vi "IETS_sweep routine_2021_subvis.vi"(0 "Yokogawa 7651":refnum<visa-resource-name>="GPIB0::13::INSTR", 1 "LIA1":refnum<visa-resource-name>="GPIB0::8::INSTR", 2 "Sens_LIA 1":dbl=0.2, 3 "AC amp":dbl=0.3, 4 "LIA2":refnum<visa-resource-name>="GPIB0::20::INSTR", 5 "file path 3":path=path "D:/MCBJ_DATA/IETS_new programm/ganz neu/S1_2021/AuAu/50mV/30_03_2021/cooldownsweep0128", 6 "pre-resistance":dbl=50.0 format="%#_13g", 7 "file path 2":path=path "D:/MCBJ_DATA/IETS_new programm/ganz neu/S1_2021/AuAu/50mV/30_03_2021/coolupsweep0128", 8 "Initail V":dbl=-0.52, 9 "CA gain":dbl=0.0001, 10 "LIA exp 2":dbl=100.0, 12 "Step (V)":dbl=0.001, 14 "Sensitivity 2":dbl=0.2, 15 "Set0 step (V)":dbl=0.002 format="%#.6g", 16 "Final V":dbl=0.52, 17 "Stop":bool, 18 "bias_in":dbl=0.05, 19 "Lia1_pase":dbl, 20 "file path":path=path "D:/MCBJ_DATA/IETS_new programm/ganz neu/S1_2021/AuAu/50mV/30_03_2021/coolIETS0128", 22 "LIA exp 1":dbl=1.0, 23 "Resistance":dbl=1832.6738253037915, 24 "motor-info":string="Data_Points   O/C_Cyles  Motor_Pos  lockin_phase  Temperature Voltage_drop LockAmpl timeLIA1 timeLIA2   OC_timestamp \r81800\t13\t333511\t90\t10.921\t234\t3\t8\t8\tH:06:31,1523\t", 26 "Cond (G0)":dbl=7.042390613771767) -> (13 "allchart_lia2":cluster{"x":dbl, "y":dbl}[](graph), 21 "VISA Agilent out":refnum<visa-resource-name>="GPIB0::10::INSTR", 25 "IV_allchart":cluster{"x":dbl, "y":dbl}[](graph), 27 "allchart_Lia1":cluster{"X":dbl, "Y":dbl}[](graph))   [LabVIEW 2016]
uses:
  Instance           2 12Saved   IETS .vi
  Agilent 3446X Series/Agilent 3446X Series.lvlib
  Keithley DMM6500 DAQ6500 Series/Keithley DMM6500 DAQ6500 Series.lvlib
  Agilent 34401/Agilent 34401.lvlib
panel:
  out "G_drop":dbl=0.054506536639635256
  out "Current mA":dbl=33.097697080199396
  out "LIA_DMM_G":dbl=-8.943673289039905
  out "sec ampl":dbl=-0.0004827649974186888
  out "Meas Bias":dbl=-0.0446874833
  out "Lia2_DMM":dbl=-0.168320844
  out "LIAI_1_DMM":dbl=-1.07675359
  out "stop last sweep":bool=TRUE
  out "Abort":bool=TRUE
  in  "Stop 2":bool
  out "Vspt":dbl=-0.052
  out "Vdrop":dbl=0.3437052
  in  "?":T1(tab)=enum."conditions"
  out "IV_chart":cluster{"x":dbl, "y":dbl}[](graph)=[{"x"=-0.338726307, "y"=884.433039501003}, {"x"=-0.338726307, "y"=884.433039501003}, {"x"=-0.338726307, "y"=884.433039501003}, {"x"=-0.338726307, "y"=884.433039501003}, {"x"=-0.338726307, "y"=884.433039501003}, {"x"=-0.338726307, "y"=884.433039501003}, {"x"=-0.338726307, "y"=884.433039501003}, {"x"=-0.338726307, "y"=884.433039501003}, {"x"=-0.338726307, "y"=884.433039501003}, {"x"=-0.338726307, "y"=884.433039501003}, {"x"=-0.338726307, "y"=884.433039501003}, {"x"=-0.338726307, "y"=884.433039501003}, {"x"=-0.338726307, "y"=884.433039501003}, {"x"=-0.338726307, "y"=884.433039501003}, {"x"=-0.338726307, "y"=884.433039501003}, {"x"=-0.338726307, "y"=884.433039501003}, {"x"=-0.338726307, "y"=884.433039501003}, {"x"=-0.338726307, "y"=884.433039501003}, {"x"=-0.338726307, "y"=884.433039501003}, {"x"=-0.338726307, "y"=884.433039501003}, {"x"=-0.338726307, "y"=884.433039501003}, {"x"=-0.338726307, "y"=884.433039501003}, {"x"=-0.338726307, "y"=884.433039501003}, {"x"=-0.338726307, "y"=884.433039501003}, {"x"=-0.338726307, "y"=884.433039501003}, {"x"=-0.338726307, "y"=884.433039501003}, {"x"=-0.338726307, "y"=884.433039501003}, {"x"=-0.338726307, "y"=884.433039501003}, {"x"=-0.338726307, "y"=884.433039501003}, {"x"=-0.338726307, "y"=884.433039501003}, {"x"=-0.338726307, "y"=884.433039501003}, {"x"=-0.338726307, "y"=884.433039501003}, {"x"=-0.338726307, "y"=884.433039501003}, {"x"=-0.338726307, "y"=884.433039501003}, {"x"=-0.338726307, "y"=884.433039501003}, {"x"=-0.338726307, "y"=884.433039501003}, {"x"=-0.338726307, "y"=884.433039501003}, {"x"=-0.338726307, "y"=884.433039501003}, {"x"=-0.338726307, "y"=884.433039501003}, {"x"=-0.338726307, "y"=884.433039501003}, {"x"=-0.338726307, "y"=884.433039501003}, {"x"=-0.338726307, "y"=884.433039501003}, {"x"=-0.338726307, "y"=884.433039501003}, {"x"=-0.338726307, "y"=884.433039501003}, {"x"=-0.338726307, "y"=884.433039501003}, {"x"=-0.338726307, "y"=884.433039501003}, {"x"=-0.338726307, "y"=884.433039501003}, {"x"=-0.338726307, "y"=884.433039501003}, {"x"=-0.338726307, "y"=884.433039501003}, {"x"=-0.338726307, "y"=884.433039501003}, {"x"=-0.338726307, "y"=884.433039501003}, {"x"=-0.338726307, "y"=884.433039501003}, {"x"=-0.338726307, "y"=884.433039501003}, {"x"=-0.338726307, "y"=884.433039501003}, {"x"=-0.338726307, "y"=884.433039501003}, {"x"=-0.338726307, "y"=884.433039501003}, {"x"=-0.338726307, "y"=884.433039501003}, {"x"=-0.338726307, "y"=884.433039501003}, {"x"=-0.338726307, "y"=884.433039501003}, {"x"=-0.338726307, "y"=884.433039501003}, {"x"=-0.338726307, "y"=884.433039501003}, {"x"=-0.338726307, "y"=884.433039501003}, {"x"=-0.338726307, "y"=884.433039501003}, {"x"=-0.338726307, "y"=884.433039501003}, {"x"=-0.338726307, "y"=884.433039501003}, {"x"=-0.338726307, "y"=884.433039501003}, {"x"=-0.338726307, "y"=884.433039501003}, {"x"=-0.338726307, "y"=884.433039501003}, {"x"=-0.338726307, "y"=884.433039501003}, {"x"=-0.338726307, "y"=884.433039501003}, {"x"=-0.338726307, "y"=884.433039501003}, {"x"=-0.338726307, "y"=884.433039501003}, {"x"=-0.338726307, "y"=884.433039501003}, {"x"=-0.338726307, "y"=884.433039501003}, {"x"=-0.338726307, "y"=884.433039501003}, {"x"=-0.338726307, "y"=884.433039501003}, {"x"=-0.338726307, "y"=884.433039501003}, {"x"=-0.338726307, "y"=884.433039501003}, {"x"=-0.338726307, "y"=884.433039501003}, {"x"=-0.338726307, "y"=884.433039501003}, {"x"=-0.338726307, "y"=884.433039501003}, {"x"=-0.338726307, "y"=884.433039501003}, {"x"=-0.338726307, "y"=884.433039501003}, {"x"=-0.338726307, "y"=884.433039501003}, {"x"=-0.338726307, "y"=884.433039501003}, {"x"=-0.338726307, "y"=884.433039501003}, {"x"=-0.338726307, "y"=884.433039501003}, {"x"=-0.338726307, "y"=884.433039501003}, {"x"=-0.338726307, "y"=884.433039501003}, {"x"=-0.338726307, "y"=884.433039501003}, {"x"=-0.338726307, "y"=884.433039501003}, {"x"=-0.338726307, "y"=884.433039501003}, {"x"=-0.338726307, "y"=884.433039501003}, {"x"=-0.338726307, "y"=884.433039501003}, {"x"=-0.338726307, "y"=884.433039501003}, {"x"=-0.338726307, "y"=884.433039501003}, {"x"=-0.338726307, "y"=884.433039501003}, {"x"=-0.338726307, "y"=884.433039501003}, {"x"=-0.338726307, "y"=884.433039501003}, {"x"=-0.338726307, "y"=884.433039501003}, {"x"=-0.338726307, "y"=884.433039501003}, {"x"=-0.338726307, "y"=884.433039501003}, {"x"=-0.338726307, "y"=884.433039501003}, {"x"=-0.338726307, "y"=884.433039501003}, {"x"=-0.338726307, "y"=884.433039501003}, {"x"=-0.338726307, "y"=884.433039501003}, {"x"=-0.338726307, "y"=884.433039501003}, {"x"=-0.338726307, "y"=884.433039501003}, {"x"=-0.338726307, "y"=884.433039501003}, {"x"=-0.338726307, "y"=884.433039501003}, {"x"=-0.338726307, "y"=884.433039501003}, {"x"=-0.338726307, "y"=884.433039501003}, {"x"=-0.338726307, "y"=884.433039501003}, {"x"=-0.338726307, "y"=884.433039501003}, {"x"=-0.338726307, "y"=884.433039501003}, {"x"=-0.338726307, "y"=884.433039501003}, {"x"=-0.338726307, "y"=884.433039501003}, {"x"=-0.338726307, "y"=884.433039501003}, {"x"=-0.338726307, "y"=884.433039501003}, {"x"=-0.338726307, "y"=884.433039501003}, {"x"=-0.338726307, "y"=884.433039501003}, {"x"=-0.338726307, "y"=884.433039501003}, {"x"=-0.338726307, "y"=884.433039501003}, {"x"=-0.338726307, "y"=884.433039501003}, {"x"=-0.338726307, "y"=884.433039501003}, {"x"=-0.338726307, "y"=884.433039501003}, {"x"=-0.338726307, "y"=884.433039501003}, {"x"=-0.338726307, "y"=884.433039501003}, {"x"=-0.338726307, "y"=884.433039501003}, {"x"=-0.338726307, "y"=884.433039501003}, {"x"=-0.338726307, "y"=884.433039501003}, {"x"=-0.338726307, "y"=884.433039501003}, {"x"=-0.338726307, "y"=884.433039501003}, {"x"=-0.338726307, "y"=884.433039501003}, {"x"=-0.338726307, "y"=884.433039501003}, {"x"=-0.338726307, "y"=884.433039501003}, {"x"=-0.338726307, "y"=884.433039501003}, {"x"=-0.338726307, "y"=884.433039501003}, {"x"=-0.338726307, "y"=884.433039501003}, {"x"=-0.338726307, "y"=884.433039501003}, {"x"=-0.338726307, "y"=884.433039501003}, {"x"=-0.338726307, "y"=884.433039501003}, {"x"=-0.338726307, "y"=884.433039501003}, {"x"=-0.338726307, "y"=884.433039501003}, {"x"=-0.338726307, "y"=884.433039501003}, {"x"=-0.338726307, "y"=884.433039501003}, {"x"=-0.338726307, "y"=884.433039501003}, {"x"=-0.338726307, "y"=884.433039501003}, {"x"=-0.338726307, "y"=884.433039501003}, {"x"=-0.338726307, "y"=884.433039501003}, {"x"=-0.338726307, "y"=884.433039501003}, {"x"=-0.338726307, "y"=884.433039501003}, {"x"=-0.338726307, "y"=884.433039501003}, {"x"=-0.338726307, "y"=884.433039501003}, {"x"=-0.338726307, "y"=884.433039501003}, {"x"=-0.338726307, "y"=884.433039501003}, {"x"=-0.338726307, "y"=884.433039501003}, {"x"=-0.338726307, "y"=884.433039501003}, {"x"=-0.338726307, "y"=884.433039501003}, {"x"=-0.338726307, "y"=884.433039501003}, {"x"=-0.338726307, "y"=884.433039501003}, {"x"=-0.338726307, "y"=884.433039501003}, {"x"=-0.338726307, "y"=884.433039501003}, {"x"=-0.338726307, "y"=884.433039501003}, {"x"=-0.338726307, "y"=884.433039501003}, {"x"=-0.338726307, "y"=884.433039501003}, {"x"=-0.338726307, "y"=884.433039501003}, {"x"=-0.338726307, "y"=884.433039501003}, {"x"=-0.338726307, "y"=884.433039501003}, {"x"=-0.338726307, "y"=884.433039501003}, {"x"=-0.338726307, "y"=884.433039501003}, {"x"=-0.338726307, "y"=884.433039501003}, {"x"=-0.338726307, "y"=884.433039501003}, {"x"=-0.338726307, "y"=884.433039501003}, {"x"=-0.338726307, "y"=884.433039501003}, {"x"=-0.338726307, "y"=884.433039501003}, {"x"=-0.338726307, "y"=884.433039501003}, {"x"=-0.338726307, "y"=884.433039501003}, {"x"=-0.338726307, "y"=884.433039501003}, {"x"=-0.338726307, "y"=884.433039501003}, {"x"=-0.338726307, "y"=884.433039501003}, {"x"=-0.338726307, "y"=884.433039501003}, {"x"=-0.338726307, "y"=884.433039501003}, {"x"=-0.338726307, "y"=884.433039501003}, {"x"=-0.338726307, "y"=884.433039501003}, {"x"=-0.338726307, "y"=884.433039501003}, {"x"=-0.338726307, "y"=884.433039501003}, {"x"=-0.338726307, "y"=884.433039501003}, {"x"=-0.338726307, "y"=884.433039501003}, {"x"=-0.338726307, "y"=884.433039501003}, {"x"=-0.338726307, "y"=884.433039501003}, {"x"=-0.338726307, "y"=884.433039501003}, {"x"=-0.338726307, "y"=884.433039501003}, {"x"=-0.338726307, "y"=884.433039501003}, {"x"=-0.338726307, "y"=884.433039501003}, {"x"=-0.338726307, "y"=884.433039501003}, {"x"=-0.338726307, "y"=884.433039501003}, {"x"=-0.338726307, "y"=884.433039501003}, {"x"=-0.338726307, "y"=884.433039501003}, {"x"=-0.338726307, "y"=884.433039501003}, {"x"=-0.338726307, "y"=884.433039501003}, {"x"=-0.338726307, "y"=884.433039501003}, {"x"=-0.338726307, "y"=884.433039501003}, {"x"=-0.338726307, "y"=884.433039501003}, {"x"=-0.338726307, "y"=884.433039501003}, {"x"=-0.338726307, "y"=884.433039501003}, {"x"=-0.338726307, "y"=884.433039501003}, {"x"=-0.338726307, "y"=884.433039501003}, {"x"=-0.338726307, "y"=884.433039501003}, {"x"=-0.338726307, "y"=884.433039501003}, {"x"=-0.338726307, "y"=884.433039501003}, {"x"=-0.338726307, "y"=884.433039501003}, {"x"=-0.338726307, "y"=884.433039501003}, {"x"=-0.338726307, "y"=884.433039501003}, {"x"=-0.338726307, "y"=884.433039501003}, {"x"=-0.338726307, "y"=884.433039501003}, {"x"=-0.338726307, "y"=884.433039501003}, {"x"=-0.338726307, "y"=884.433039501003}, {"x"=-0.338726307, "y"=884.433039501003}, {"x"=-0.338726307, "y"=884.433039501003}, {"x"=-0.338726307, "y"=884.433039501003}, {"x"=-0.338726307, "y"=884.433039501003}, {"x"=-0.338726307, "y"=884.433039501003}, {"x"=-0.338726307, "y"=884.433039501003}, {"x"=-0.338726307, "y"=884.433039501003}, {"x"=-0.338726307, "y"=884.433039501003}, {"x"=-0.338726307, "y"=884.433039501003}, {"x"=-0.338726307, "y"=884.433039501003}, {"x"=-0.338726307, "y"=884.433039501003}, {"x"=-0.338726307, "y"=884.433039501003}, {"x"=-0.338726307, "y"=884.433039501003}, {"x"=-0.338726307, "y"=884.433039501003}, {"x"=-0.338726307, "y"=884.433039501003}, {"x"=-0.338726307, "y"=884.433039501003}, {"x"=-0.338726307, "y"=884.433039501003}, {"x"=-0.338726307, "y"=884.433039501003}, {"x"=-0.338726307, "y"=884.433039501003}, {"x"=-0.338726307, "y"=884.433039501003}, {"x"=-0.338726307, "y"=884.433039501003}, {"x"=-0.338726307, "y"=884.433039501003}, {"x"=-0.338726307, "y"=884.433039501003}, {"x"=-0.338726307, "y"=884.433039501003}, {"x"=-0.338726307, "y"=884.433039501003}, {"x"=-0.338726307, "y"=884.433039501003}, {"x"=-0.338726307, "y"=884.433039501003}, {"x"=-0.338726307, "y"=884.433039501003}, {"x"=-0.338726307, "y"=884.433039501003}, {"x"=-0.338726307, "y"=884.433039501003}, {"x"=-0.338726307, "y"=884.433039501003}, {"x"=-0.338726307, "y"=884.433039501003}, {"x"=-0.338726307, "y"=884.433039501003}, {"x"=-0.338726307, "y"=884.433039501003}, {"x"=-0.338726307, "y"=884.433039501003}, {"x"=-0.338726307, "y"=884.433039501003}, {"x"=-0.338726307, "y"=884.433039501003}, {"x"=-0.338726307, "y"=884.433039501003}, {"x"=-0.338726307, "y"=884.433039501003}, {"x"=-0.338726307, "y"=884.433039501003}, {"x"=-0.338726307, "y"=884.433039501003}, {"x"=-0.338726307, "y"=884.433039501003}, {"x"=-0.338726307, "y"=884.433039501003}, {"x"=-0.338726307, "y"=884.433039501003}, {"x"=-0.338726307, "y"=884.433039501003}, {"x"=-0.338726307, "y"=884.433039501003}, {"x"=-0.338726307, "y"=884.433039501003}, {"x"=-0.338726307, "y"=884.433039501003}, {"x"=-0.338726307, "y"=884.433039501003}, {"x"=-0.338726307, "y"=884.433039501003}, {"x"=-0.338726307, "y"=884.433039501003}, {"x"=-0.338726307, "y"=884.433039501003}, {"x"=-0.338726307, "y"=884.433039501003}, {"x"=-0.338726307, "y"=884.433039501003}, {"x"=-0.338726307, "y"=884.433039501003}, {"x"=-0.338726307, "y"=884.433039501003}, {"x"=-0.338726307, "y"=884.433039501003}, {"x"=-0.338726307, "y"=884.433039501003}, {"x"=-0.338726307, "y"=884.433039501003}, {"x"=-0.338726307, "y"=884.433039501003}, {"x"=-0.338726307, "y"=884.433039501003}, {"x"=-0.338726307, "y"=884.433039501003}, {"x"=-0.338726307, "y"=884.433039501003}, {"x"=-0.338726307, "y"=884.433039501003}, {"x"=-0.338726307, "y"=884.433039501003}, {"x"=-0.338726307, "y"=884.433039501003}, {"x"=-0.338726307, "y"=884.433039501003}, {"x"=-0.338726307, "y"=884.433039501003}, {"x"=-0.338726307, "y"=884.433039501003}, {"x"=-0.338726307, "y"=884.433039501003}, {"x"=-0.338726307, "y"=884.433039501003}, {"x"=-0.338726307, "y"=884.433039501003}, {"x"=-0.338726307, "y"=884.433039501003}, {"x"=-0.338726307, "y"=884.433039501003}, {"x"=-0.338726307, "y"=884.433039501003}, {"x"=-0.338726307, "y"=884.433039501003}, {"x"=-0.338726307, "y"=884.433039501003}, {"x"=-0.338726307, "y"=884.433039501003}, {"x"=-0.338726307, "y"=884.433039501003}, {"x"=-0.338726307, "y"=884.433039501003}, {"x"=-0.338726307, "y"=884.433039501003}, {"x"=-0.338726307, "y"=884.433039501003}, {"x"=-0.338726307, "y"=884.433039501003}, {"x"=-0.338726307, "y"=884.433039501003}, {"x"=-0.338726307, "y"=884.433039501003}, {"x"=-0.338726307, "y"=884.433039501003}, {"x"=-0.338726307, "y"=884.433039501003}, {"x"=-0.338726307, "y"=884.433039501003}, {"x"=-0.338726307, "y"=884.433039501003}, {"x"=-0.338726307, "y"=884.433039501003}, {"x"=-0.338726307, "y"=884.433039501003}, {"x"=-0.338726307, "y"=884.433039501003}, {"x"=-0.338726307, "y"=884.433039501003}, {"x"=-0.338726307, "y"=884.433039501003}, {"x"=-0.338726307, "y"=884.433039501003}, {"x"=-0.338726307, "y"=884.433039501003}, {"x"=-0.338726307, "y"=884.433039501003}, {"x"=-0.338726307, "y"=884.433039501003}, {"x"=-0.338726307, "y"=884.433039501003}, {"x"=-0.338726307, "y"=884.433039501003}, {"x"=-0.338726307, "y"=884.433039501003}, {"x"=-0.338726307, "y"=884.433039501003}, {"x"=-0.338726307, "y"=884.433039501003}, {"x"=-0.338726307, "y"=884.433039501003}, {"x"=-0.338726307, "y"=884.433039501003}, {"x"=-0.338726307, "y"=884.433039501003}, {"x"=-0.338726307, "y"=884.433039501003}, {"x"=-0.338726307, "y"=884.433039501003}, {"x"=-0.338726307, "y"=884.433039501003}, {"x"=-0.338726307, "y"=884.433039501003}, {"x"=-0.338726307, "y"=884.433039501003}, {"x"=-0.338726307, "y"=884.433039501003}, {"x"=-0.338726307, "y"=884.433039501003}, {"x"=-0.338726307, "y"=884.433039501003}, {"x"=-0.338726307, "y"=884.433039501003}, {"x"=-0.338726307, "y"=884.433039501003}, {"x"=-0.338726307, "y"=884.433039501003}, {"x"=-0.338726307, "y"=884.433039501003}, {"x"=-0.338726307, "y"=884.433039501003}, {"x"=-0.338726307, "y"=884.433039501003}, {"x"=-0.338726307, "y"=884.433039501003}, {"x"=-0.338726307, "y"=884.433039501003}, {"x"=-0.338726307, "y"=884.433039501003}, {"x"=-0.338726307, "y"=884.433039501003}, {"x"=-0.338726307, "y"=884.433039501003}, {"x"=-0.338726307, "y"=884.433039501003}, {"x"=-0.338726307, "y"=884.433039501003}, {"x"=-0.338726307, "y"=884.433039501003}, {"x"=-0.338726307, "y"=884.433039501003}, {"x"=-0.338726307, "y"=884.433039501003}, {"x"=-0.338726307, "y"=884.433039501003}, {"x"=-0.338726307, "y"=884.433039501003}, {"x"=-0.338726307, "y"=884.433039501003}, {"x"=-0.338726307, "y"=884.433039501003}, {"x"=-0.338726307, "y"=884.433039501003}, {"x"=-0.338726307, "y"=884.433039501003}, {"x"=-0.338726307, "y"=884.433039501003}, {"x"=-0.338726307, "y"=884.433039501003}, {"x"=-0.338726307, "y"=884.433039501003}, {"x"=-0.338726307, "y"=884.433039501003}, {"x"=-0.338726307, "y"=884.433039501003}, {"x"=-0.338726307, "y"=884.433039501003}, {"x"=-0.338726307, "y"=884.433039501003}, {"x"=-0.338726307, "y"=884.433039501003}, {"x"=-0.338726307, "y"=884.433039501003}, {"x"=-0.338726307, "y"=884.433039501003}, {"x"=-0.338726307, "y"=884.433039501003}, {"x"=-0.338726307, "y"=884.433039501003}, {"x"=-0.338726307, "y"=884.433039501003}, {"x"=-0.338726307, "y"=884.433039501003}, {"x"=-0.338726307, "y"=884.433039501003}, {"x"=-0.338726307, "y"=884.433039501003}, {"x"=-0.338726307, "y"=884.433039501003}, {"x"=-0.338726307, "y"=884.433039501003}, {"x"=-0.338726307, "y"=884.433039501003}, {"x"=-0.338726307, "y"=884.433039501003}, {"x"=-0.338726307, "y"=884.433039501003}, {"x"=-0.338726307, "y"=884.433039501003}, {"x"=-0.338726307, "y"=884.433039501003}, {"x"=-0.338726307, "y"=884.433039501003}, {"x"=-0.338726307, "y"=884.433039501003}, {"x"=-0.338726307, "y"=884.433039501003}, {"x"=-0.338726307, "y"=884.433039501003}, {"x"=-0.338726307, "y"=884.433039501003}, {"x"=-0.338726307, "y"=884.433039501003}, {"x"=-0.338726307, "y"=884.433039501003}, {"x"=-0.338726307, "y"=884.433039501003}, {"x"=-0.338726307, "y"=884.433039501003}, {"x"=-0.338726307, "y"=884.433039501003}, {"x"=-0.338726307, "y"=884.433039501003}, {"x"=-0.338726307, "y"=884.433039501003}, {"x"=-0.338726307, "y"=884.433039501003}, {"x"=-0.338726307, "y"=884.433039501003}, {"x"=-0.338726307, "y"=884.433039501003}, {"x"=-0.338726307, "y"=884.433039501003}, {"x"=-0.338726307, "y"=884.433039501003}, {"x"=-0.338726307, "y"=884.433039501003}, {"x"=-0.338726307, "y"=884.433039501003}, {"x"=-0.338726307, "y"=884.433039501003}, {"x"=-0.338726307, "y"=884.433039501003}, {"x"=-0.338726307, "y"=884.433039501003}, {"x"=-0.338726307, "y"=884.433039501003}, {"x"=-0.338726307, "y"=884.433039501003}, {"x"=-0.338726307, "y"=884.433039501003}, {"x"=-0.338726307, "y"=884.433039501003}, {"x"=-0.338726307, "y"=884.433039501003}, {"x"=-0.338726307, "y"=884.433039501003}, {"x"=-0.338726307, "y"=884.433039501003}, {"x"=-0.338726307, "y"=884.433039501003}, {"x"=-0.338726307, "y"=884.433039501003}, {"x"=-0.338726307, "y"=884.433039501003}, {"x"=-0.338726307, "y"=884.433039501003}, {"x"=-0.338726307, "y"=884.433039501003}, {"x"=-0.338726307, "y"=884.433039501003}, {"x"=-0.338726307, "y"=884.433039501003}, {"x"=-0.338726307, "y"=884.433039501003}, {"x"=-0.338726307, "y"=884.433039501003}, {"x"=-0.338726307, "y"=884.433039501003}, {"x"=-0.338726307, "y"=884.433039501003}, {"x"=-0.338726307, "y"=884.433039501003}, {"x"=-0.338726307, "y"=884.433039501003}, {"x"=-0.338726307, "y"=884.433039501003}, {"x"=-0.338726307, "y"=884.433039501003}, {"x"=-0.338726307, "y"=884.433039501003}, {"x"=-0.338726307, "y"=884.433039501003}, {"x"=-0.338726307, "y"=884.433039501003}, {"x"=-0.338726307, "y"=884.433039501003}, {"x"=-0.338726307, "y"=884.433039501003}, {"x"=-0.338726307, "y"=884.433039501003}, {"x"=-0.338726307, "y"=884.433039501003}, {"x"=-0.338726307, "y"=884.433039501003}, {"x"=-0.338726307, "y"=884.433039501003}, {"x"=-0.338726307, "y"=884.433039501003}, {"x"=-0.338726307, "y"=884.433039501003}, {"x"=-0.338726307, "y"=884.433039501003}, {"x"=-0.338726307, "y"=884.433039501003}, {"x"=-0.338726307, "y"=884.433039501003}, {"x"=-0.338726307, "y"=884.433039501003}, {"x"=-0.338726307, "y"=884.433039501003}, {"x"=-0.338726307, "y"=884.433039501003}, {"x"=-0.338726307, "y"=884.433039501003}, {"x"=-0.338726307, "y"=884.433039501003}, {"x"=-0.338726307, "y"=884.433039501003}, {"x"=-0.338726307, "y"=884.433039501003}, {"x"=-0.338726307, "y"=884.433039501003}, {"x"=-0.338726307, "y"=884.433039501003}, {"x"=-0.338726307, "y"=884.433039501003}, {"x"=-0.338726307, "y"=884.433039501003}, {"x"=-0.338726307, "y"=884.433039501003}, {"x"=-0.338726307, "y"=884.433039501003}, {"x"=-0.338726307, "y"=884.433039501003}, {"x"=-0.338726307, "y"=884.433039501003}, {"x"=-0.338726307, "y"=884.433039501003}, {"x"=-0.338726307, "y"=884.433039501003}, {"x"=-0.338726307, "y"=884.433039501003}, {"x"=-0.338726307, "y"=884.433039501003}, {"x"=-0.338726307, "y"=884.433039501003}, {"x"=-0.338726307, "y"=884.433039501003}, {"x"=-0.338726307, "y"=884.433039501003}, {"x"=-0.338726307, "y"=884.433039501003}, {"x"=-0.338726307, "y"=884.433039501003}, {"x"=-0.338726307, "y"=884.433039501003}, {"x"=-0.338726307, "y"=884.433039501003}, {"x"=-0.338726307, "y"=884.433039501003}, {"x"=-0.338726307, "y"=884.433039501003}, {"x"=-0.338726307, "y"=884.433039501003}, {"x"=-0.338726307, "y"=884.433039501003}, {"x"=-0.338726307, "y"=884.433039501003}, {"x"=-0.338726307, "y"=884.433039501003}, {"x"=-0.338726307, "y"=884.433039501003}, {"x"=-0.338726307, "y"=884.433039501003}, {"x"=-0.338726307, "y"=884.433039501003}, {"x"=-0.338726307, "y"=884.433039501003}, {"x"=-0.338726307, "y"=884.433039501003}, {"x"=-0.338726307, "y"=884.433039501003}, {"x"=-0.338726307, "y"=884.433039501003}, {"x"=-0.338726307, "y"=884.433039501003}, {"x"=-0.338726307, "y"=884.433039501003}, {"x"=-0.338726307, "y"=884.433039501003}, {"x"=-0.338726307, "y"=884.433039501003}, {"x"=-0.338726307, "y"=884.433039501003}, {"x"=-0.338726307, "y"=884.433039501003}, {"x"=-0.338726307, "y"=884.433039501003}, {"x"=-0.338726307, "y"=884.433039501003}, {"x"=-0.338726307, "y"=884.433039501003}, {"x"=-0.338726307, "y"=884.433039501003}, {"x"=-0.338726307, "y"=884.433039501003}, {"x"=-0.338726307, "y"=884.433039501003}, {"x"=-0.338726307, "y"=884.433039501003}, {"x"=-0.338726307, "y"=884.433039501003}, {"x"=-0.338726307, "y"=884.433039501003}, {"x"=-0.338726307, "y"=884.433039501003}, {"x"=-0.338726307, "y"=884.433039501003}, {"x"=-0.338726307, "y"=884.433039501003}, {"x"=-0.338726307, "y"=884.433039501003}, {"x"=-0.338726307, "y"=884.433039501003}, {"x"=-0.338726307, "y"=884.433039501003}, {"x"=-0.338726307, "y"=884.433039501003}, {"x"=-0.338726307, "y"=884.433039501003}, {"x"=-0.338726307, "y"=884.433039501003}, {"x"=-0.338726307, "y"=884.433039501003}, {"x"=-0.338726307, "y"=884.433039501003}, {"x"=-0.338726307, "y"=884.433039501003}, {"x"=-0.338726307, "y"=884.433039501003}, {"x"=-0.338726307, "y"=884.433039501003}, {"x"=-0.338726307, "y"=884.433039501003}, {"x"=-0.338726307, "y"=884.433039501003}, {"x"=-0.338726307, "y"=884.433039501003}, {"x"=-0.338726307, "y"=884.433039501003}, {"x"=-0.338726307, "y"=884.433039501003}, {"x"=-0.338726307, "y"=884.433039501003}, {"x"=-0.338726307, "y"=884.433039501003}, {"x"=-0.338726307, "y"=884.433039501003}, {"x"=-0.338726307, "y"=884.433039501003}, {"x"=-0.338726307, "y"=884.433039501003}, {"x"=-0.338726307, "y"=884.433039501003}, {"x"=-0.338726307, "y"=884.433039501003}, {"x"=-0.338726307, "y"=884.433039501003}, {"x"=-0.338726307, "y"=884.433039501003}, {"x"=-0.338726307, "y"=884.433039501003}, {"x"=-0.338726307, "y"=884.433039501003}, {"x"=-0.338726307, "y"=884.433039501003}, {"x"=-0.338726307, "y"=884.433039501003}, {"x"=-0.338726307, "y"=884.433039501003}, {"x"=-0.338726307, "y"=884.433039501003}, {"x"=-0.338726307, "y"=884.433039501003}, {"x"=-0.338726307, "y"=884.433039501003}, {"x"=-0.338726307, "y"=884.433039501003}, {"x"=-0.338726307, "y"=884.433039501003}, {"x"=-0.338726307, "y"=884.433039501003}, {"x"=-0.338726307, "y"=884.433039501003}, {"x"=-0.338726307, "y"=884.433039501003}, {"x"=-0.338726307, "y"=884.433039501003}, {"x"=-0.338726307, "y"=884.433039501003}, {"x"=-0.338726307, "y"=884.433039501003}, {"x"=-0.338726307, "y"=884.433039501003}, {"x"=-0.338726307, "y"=884.433039501003}, {"x"=-0.338726307, "y"=884.433039501003}, {"x"=-0.338726307, "y"=884.433039501003}, {"x"=-0.338726307, "y"=884.433039501003}, {"x"=-0.338726307, "y"=884.433039501003}, {"x"=-0.338726307, "y"=884.433039501003}, {"x"=-0.338726307, "y"=884.433039501003}, {"x"=-0.338726307, "y"=884.433039501003}, {"x"=-0.338726307, "y"=884.433039501003}, {"x"=-0.338726307, "y"=884.433039501003}, {"x"=-0.338726307, "y"=884.433039501003}, {"x"=-0.338726307, "y"=884.433039501003}, {"x"=-0.338726307, "y"=884.433039501003}, {"x"=-0.338726307, "y"=884.433039501003}, {"x"=-0.338726307, "y"=884.433039501003}, {"x"=-0.338726307, "y"=884.433039501003}, {"x"=-0.338726307, "y"=884.433039501003}, {"x"=-0.338726307, "y"=884.433039501003}, {"x"=-0.338726307, "y"=884.433039501003}, {"x"=-0.338726307, "y"=884.433039501003}, {"x"=-0.338726307, "y"=884.433039501003}, {"x"=-0.338726307, "y"=884.433039501003}, {"x"=-0.338726307, "y"=884.433039501003}, {"x"=-0.338726307, "y"=884.433039501003}, {"x"=-0.338726307, "y"=884.433039501003}, {"x"=-0.338726307, "y"=884.433039501003}, {"x"=-0.338726307, "y"=884.433039501003}, {"x"=-0.338726307, "y"=884.433039501003}, {"x"=-0.338726307, "y"=884.433039501003}, {"x"=-0.338726307, "y"=884.433039501003}, {"x"=-0.338726307, "y"=884.433039501003}, {"x"=-0.338726307, "y"=884.433039501003}, {"x"=-0.338726307, "y"=884.433039501003}, {"x"=-0.338726307, "y"=884.433039501003}, {"x"=-0.338726307, "y"=884.433039501003}, {"x"=-0.338726307, "y"=884.433039501003}, {"x"=-0.338726307, "y"=884.433039501003}, {"x"=-0.338726307, "y"=884.433039501003}, {"x"=-0.338726307, "y"=884.433039501003}, {"x"=-0.338726307, "y"=884.433039501003}, {"x"=-0.338726307, "y"=884.433039501003}, {"x"=-0.338726307, "y"=884.433039501003}, {"x"=-0.338726307, "y"=884.433039501003}, {"x"=-0.338726307, "y"=884.433039501003}, {"x"=-0.338726307, "y"=884.433039501003}, {"x"=-0.338726307, "y"=884.433039501003}, {"x"=-0.336933848, "y"=878.6315369129212}, {"x"=-0.335312612, "y"=870.2341761881793}, {"x"=-0.333588895, "y"=868.8284717376354}, {"x"=-0.331523407, "y"=864.9467907076084}, {"x"=-0.32981741, "y"=856.3034258660856}, {"x"=-0.328028071, "y"=851.4532355828264}, {"x"=-0.326401821, "y"=849.2069663743162}, {"x"=-0.324984329, "y"=843.4416914313405}, {"x"=-0.323264419, "y"=841.27699630987}, {"x"=-0.321215795, "y"=836.2042971720443}, {"x"=-0.319429341, "y"=827.7556209399958}, {"x"=-0.317705652, "y"=823.465213421341}, {"x"=-0.316252294, "y"=819.2137418357268}, {"x"=-0.314273418, "y"=816.7089313501546}, {"x"=-0.312616976, "y"=810.4377738352456}, {"x"=-0.311250279, "y"=807.151900897537}, {"x"=-0.309309309, "y"=801.9697038340424}, {"x"=-0.307867444, "y"=793.7500524601983}, {"x"=-0.306006106, "y"=792.2596298269306}, {"x"=-0.304098247, "y"=783.6878259685263}, {"x"=-0.302632408, "y"=782.0449362480502}, {"x"=-0.300806821, "y"=779.3858612529581}, {"x"=-0.298836948, "y"=768.389686546151}, {"x"=-0.297571904, "y"=761.601659519925}, {"x"=-0.295886637, "y"=757.027500643989}, {"x"=-0.294614436, "y"=750.4714902752004}, {"x"=-0.293054135, "y"=743.5964132428034}, {"x"=-0.291070233, "y"=740.3679999962712}, {"x"=-0.289213666, "y"=733.2359858337485}, {"x"=-0.287506173, "y"=726.6372672848719}, {"x"=-0.286004532, "y"=724.1858820319453}, {"x"=-0.284008765, "y"=717.4925726626853}, {"x"=-0.282480195, "y"=715.2206920381815}, {"x"=-0.281034734, "y"=709.2766484696162}, {"x"=-0.278962449, "y"=701.4105996989882}, {"x"=-0.277211169, "y"=697.7460783305388}, {"x"=-0.275869818, "y"=692.9338443400146}, {"x"=-0.275858707, "y"=656.812131569311}, {"x"=-0.274265871, "y"=651.9570324753463}, {"x"=-0.272790832, "y"=650.3414574320853}, {"x"=-0.271063181, "y"=645.5461485391778}, {"x"=-0.2691099, "y"=641.7852878364986}, {"x"=-0.267199649, "y"=637.6817084240137}, {"x"=-0.265874043, "y"=633.434404621396}, {"x"=-0.26388427, "y"=627.8543056844669}, {"x"=-0.262478602, "y"=621.1195700605116}, {"x"=-0.260488689, "y"=616.1956585273862}, {"x"=-0.261151761, "y"=569.7271362953551}, {"x"=-0.260207725, "y"=559.1766129217405}, {"x"=-0.258501565, "y"=558.2552349952078}, {"x"=-0.256827198, "y"=553.8490674131216}, {"x"=-0.254823982, "y"=547.4679157419873}, {"x"=-0.257024388, "y"=476.6525346227702}, {"x"=-0.255086829, "y"=476.0674076303325}, {"x"=-0.253267682, "y"=471.57516553726913}, {"x"=-0.251461911, "y"=468.3739488640223}, {"x"=-0.250102396, "y"=464.5242209686317}, {"x"=-0.25231274, "y"=392.29336822120626}, {"x"=-0.250012497, "y"=397.2081087829067}, {"x"=-0.248991208, "y"=384.77785120881987}, {"x"=-0.248949448, "y"=351.2979233538393}, {"x"=-0.246512783, "y"=354.1023849578145}, {"x"=-0.244667033, "y"=350.43285381813115}, {"x"=-0.243755129, "y"=334.0716336780838}, {"x"=-0.241992414, "y"=331.8495016063616}, {"x"=-0.239839622, "y"=332.61098600567306}, {"x"=-0.239282604, "y"=300.7760053233296}, {"x"=-0.239071311, "y"=278.11074601327704}, {"x"=-0.237169503, "y"=276.63379913569963}, {"x"=-0.235139523, "y"=273.64566188343497}, {"x"=-0.233476595, "y"=273.29937333732425}, {"x"=-0.231414947, "y"=270.9825325456654}, {"x"=-0.229720153, "y"=268.35668825992377}, {"x"=-0.227508415, "y"=266.1578875520864}, {"x"=-0.225529067, "y"=262.03990366716744}, {"x"=-0.223780059, "y"=258.22605303456197}, {"x"=-0.22195849, "y"=259.5725321192493}, {"x"=-0.219702213, "y"=260.3257782483435}, {"x"=-0.218086488, "y"=257.40323165302226}, {"x"=-0.216224865, "y"=255.6425981475356}, {"x"=-0.214102332, "y"=250.63126761883427}, {"x"=-0.212315332, "y"=248.55661023533193}, {"x"=-0.210746278, "y"=245.52401700210828}, {"x"=-0.208862816, "y"=245.13763637143063}, {"x"=-0.206678716, "y"=241.53982789700575}, {"x"=-0.205282319, "y"=238.79461272479952}, {"x"=-0.203265687, "y"=236.2560099513591}, {"x"=-0.2015471, "y"=234.2936817559461}, {"x"=-0.199490385, "y"=231.11328706150005}, {"x"=-0.199987848, "y"=189.59262801142557}, {"x"=-0.19790616, "y"=183.6388721456731}, {"x"=-0.196052649, "y"=183.70235996298914}, {"x"=-0.194518356, "y"=181.6136734463117}, {"x"=-0.19240891, "y"=179.79870540579597}, {"x"=-0.190259549, "y"=177.00383496541102}, {"x"=-0.188408297, "y"=175.04089472846053}, {"x"=-0.186784842, "y"=173.04569516827976}, {"x"=-0.185015955, "y"=172.1818032639124}, {"x"=-0.182885565, "y"=170.27643456927112}, {"x"=-0.18075409, "y"=168.2637476055619}, {"x"=-0.178960146, "y"=165.64333944558462}, {"x"=-0.176972854, "y"=164.5934150575789}, {"x"=-0.17499795, "y"=163.59436038866156}, {"x"=-0.173542057, "y"=161.61717696512895}, {"x"=-0.171253542, "y"=161.24454958621828}, {"x"=-0.169640817, "y"=158.4490123635685}, {"x"=-0.167536408, "y"=156.6010898208051}, {"x"=-0.165963029, "y"=154.3672572482624}, {"x"=-0.163859733, "y"=152.5098843911307}, {"x"=-0.162155989, "y"=150.9579961504818}, {"x"=-0.16020872, "y"=148.07993776324042}, {"x"=-0.158036963, "y"=145.7504395072006}, {"x"=-0.15598597, "y"=144.11481510573208}, {"x"=-0.155628749, "y"=117.73567482270747}, {"x"=-0.153581019, "y"=116.39902388642128}, {"x"=-0.151648848, "y"=115.34923542660412}, {"x"=-0.149635681, "y"=113.44684701785175}, {"x"=-0.147979192, "y"=111.62248815187075}, {"x"=-0.145805958, "y"=111.55579752109708}, {"x"=-0.144300464, "y"=108.68465837109206}, {"x"=-0.142056117, "y"=106.95790848873648}, {"x"=-0.140047045, "y"=106.49555771905415}, {"x"=-0.138373454, "y"=104.73814025025277}, {"x"=-0.136218379, "y"=104.21907977365443}, {"x"=-0.134380383, "y"=100.61334709416637}, {"x"=-0.132730532, "y"=101.26051979500001}, {"x"=-0.130530307, "y"=98.16114706336471}, {"x"=-0.128886387, "y"=96.75645391958109}, {"x"=-0.126604636, "y"=95.68279145746963}, {"x"=-0.124698588, "y"=95.04740194524018}, {"x"=-0.122838797, "y"=93.47118636020363}, {"x"=-0.121222399, "y"=90.18477155087398}, {"x"=-0.118909575, "y"=90.45232786178038}, {"x"=-0.117473761, "y"=87.24684115974961}, {"x"=-0.115477579, "y"=87.33224137389547}, {"x"=-0.110103078, "y"=82.29670344693739}, {"x"=-0.108224772, "y"=80.24829648793096}, {"x"=-0.105929355, "y"=80.77725976576434}, {"x"=-0.104081993, "y"=77.63467176812065}, {"x"=-0.102250618, "y"=76.14571250090528}, {"x"=-0.100195133, "y"=75.0904213439085}, {"x"=-0.098527987, "y"=73.94544533856087}, {"x"=-0.0965328678, "y"=71.80756604913604}, {"x"=-0.0942980484, "y"=70.6516825421272}, {"x"=-0.0922350638, "y"=69.55625774576487}, {"x"=-0.0906668875, "y"=66.86516145735212}, {"x"=-0.088716553, "y"=65.75792223441633}, {"x"=-0.0863975638, "y"=64.61812762593823}, {"x"=-0.0846814559, "y"=63.71176382058571}, {"x"=-0.083004609, "y"=62.489492327253366}, {"x"=-0.0810332006, "y"=61.10906351947249}, {"x"=-0.0788357726, "y"=58.94394208569196}, {"x"=-0.0772556174, "y"=57.054852364518965}, {"x"=-0.075003195, "y"=55.79258741343977}, {"x"=-0.0734207429, "y"=54.213390544110126}, {"x"=-0.0712544511, "y"=53.80434816292922}, {"x"=-0.069650716, "y"=51.589419468513135}, {"x"=-0.0674068702, "y"=50.91918936208645}, {"x"=-0.0658028379, "y"=49.19151681473346}, {"x"=-0.0638702748, "y"=47.76309444621361}, {"x"=-0.0619029191, "y"=46.45586011453577}, {"x"=-0.0597272892, "y"=43.69222224725441}, {"x"=-0.0578072933, "y"=43.081868185747716}, {"x"=-0.0562117806, "y"=41.59481648220949}, {"x"=-0.05445193, "y"=39.84913494778545}, {"x"=-0.0525810858, "y"=39.435874891246385}, {"x"=-0.0502857008, "y"=37.59417718014978}, {"x"=-0.0486110902, "y"=36.68503622500141}, {"x"=-0.0464787007, "y"=35.04369485697346}, {"x"=-0.0446874833, "y"=33.097697080199396}]
  out "LIA1_chart":cluster{"x":dbl, "y":dbl}[](graph)=[{"x"=-0.338726307, "y"=-31.443668419022938}, {"x"=-0.338726307, "y"=-31.443668419022938}, {"x"=-0.338726307, "y"=-31.443668419022938}, {"x"=-0.338726307, "y"=-31.443668419022938}, {"x"=-0.338726307, "y"=-31.443668419022938}, {"x"=-0.338726307, "y"=-31.443668419022938}, {"x"=-0.338726307, "y"=-31.443668419022938}, {"x"=-0.338726307, "y"=-31.443668419022938}, {"x"=-0.338726307, "y"=-31.443668419022938}, {"x"=-0.338726307, "y"=-31.443668419022938}, {"x"=-0.338726307, "y"=-31.443668419022938}, {"x"=-0.338726307, "y"=-31.443668419022938}, {"x"=-0.338726307, "y"=-31.443668419022938}, {"x"=-0.338726307, "y"=-31.443668419022938}, {"x"=-0.338726307, "y"=-31.443668419022938}, {"x"=-0.338726307, "y"=-31.443668419022938}, {"x"=-0.338726307, "y"=-31.443668419022938}, {"x"=-0.338726307, "y"=-31.443668419022938}, {"x"=-0.338726307, "y"=-31.443668419022938}, {"x"=-0.338726307, "y"=-31.443668419022938}, {"x"=-0.338726307, "y"=-31.443668419022938}, {"x"=-0.338726307, "y"=-31.443668419022938}, {"x"=-0.338726307, "y"=-31.443668419022938}, {"x"=-0.338726307, "y"=-31.443668419022938}, {"x"=-0.338726307, "y"=-31.443668419022938}, {"x"=-0.338726307, "y"=-31.443668419022938}, {"x"=-0.338726307, "y"=-31.443668419022938}, {"x"=-0.338726307, "y"=-31.443668419022938}, {"x"=-0.338726307, "y"=-31.443668419022938}, {"x"=-0.338726307, "y"=-31.443668419022938}, {"x"=-0.338726307, "y"=-31.443668419022938}, {"x"=-0.338726307, "y"=-31.443668419022938}, {"x"=-0.338726307, "y"=-31.443668419022938}, {"x"=-0.338726307, "y"=-31.443668419022938}, {"x"=-0.338726307, "y"=-31.443668419022938}, {"x"=-0.338726307, "y"=-31.443668419022938}, {"x"=-0.338726307, "y"=-31.443668419022938}, {"x"=-0.338726307, "y"=-31.443668419022938}, {"x"=-0.338726307, "y"=-31.443668419022938}, {"x"=-0.338726307, "y"=-31.443668419022938}, {"x"=-0.338726307, "y"=-31.443668419022938}, {"x"=-0.338726307, "y"=-31.443668419022938}, {"x"=-0.338726307, "y"=-31.443668419022938}, {"x"=-0.338726307, "y"=-31.443668419022938}, {"x"=-0.338726307, "y"=-31.443668419022938}, {"x"=-0.338726307, "y"=-31.443668419022938}, {"x"=-0.338726307, "y"=-31.443668419022938}, {"x"=-0.338726307, "y"=-31.443668419022938}, {"x"=-0.338726307, "y"=-31.443668419022938}, {"x"=-0.338726307, "y"=-31.443668419022938}, {"x"=-0.338726307, "y"=-31.443668419022938}, {"x"=-0.338726307, "y"=-31.443668419022938}, {"x"=-0.338726307, "y"=-31.443668419022938}, {"x"=-0.338726307, "y"=-31.443668419022938}, {"x"=-0.338726307, "y"=-31.443668419022938}, {"x"=-0.338726307, "y"=-31.443668419022938}, {"x"=-0.338726307, "y"=-31.443668419022938}, {"x"=-0.338726307, "y"=-31.443668419022938}, {"x"=-0.338726307, "y"=-31.443668419022938}, {"x"=-0.338726307, "y"=-31.443668419022938}, {"x"=-0.338726307, "y"=-31.443668419022938}, {"x"=-0.338726307, "y"=-31.443668419022938}, {"x"=-0.338726307, "y"=-31.443668419022938}, {"x"=-0.338726307, "y"=-31.443668419022938}, {"x"=-0.338726307, "y"=-31.443668419022938}, {"x"=-0.338726307, "y"=-31.443668419022938}, {"x"=-0.338726307, "y"=-31.443668419022938}, {"x"=-0.338726307, "y"=-31.443668419022938}, {"x"=-0.338726307, "y"=-31.443668419022938}, {"x"=-0.338726307, "y"=-31.443668419022938}, {"x"=-0.338726307, "y"=-31.443668419022938}, {"x"=-0.338726307, "y"=-31.443668419022938}, {"x"=-0.338726307, "y"=-31.443668419022938}, {"x"=-0.338726307, "y"=-31.443668419022938}, {"x"=-0.338726307, "y"=-31.443668419022938}, {"x"=-0.338726307, "y"=-31.443668419022938}, {"x"=-0.338726307, "y"=-31.443668419022938}, {"x"=-0.338726307, "y"=-31.443668419022938}, {"x"=-0.338726307, "y"=-31.443668419022938}, {"x"=-0.338726307, "y"=-31.443668419022938}, {"x"=-0.338726307, "y"=-31.443668419022938}, {"x"=-0.338726307, "y"=-31.443668419022938}, {"x"=-0.338726307, "y"=-31.443668419022938}, {"x"=-0.338726307, "y"=-31.443668419022938}, {"x"=-0.338726307, "y"=-31.443668419022938}, {"x"=-0.338726307, "y"=-31.443668419022938}, {"x"=-0.338726307, "y"=-31.443668419022938}, {"x"=-0.338726307, "y"=-31.443668419022938}, {"x"=-0.338726307, "y"=-31.443668419022938}, {"x"=-0.338726307, "y"=-31.443668419022938}, {"x"=-0.338726307, "y"=-31.443668419022938}, {"x"=-0.338726307, "y"=-31.443668419022938}, {"x"=-0.338726307, "y"=-31.443668419022938}, {"x"=-0.338726307, "y"=-31.443668419022938}, {"x"=-0.338726307, "y"=-31.443668419022938}, {"x"=-0.338726307, "y"=-31.443668419022938}, {"x"=-0.338726307, "y"=-31.443668419022938}, {"x"=-0.338726307, "y"=-31.443668419022938}, {"x"=-0.338726307, "y"=-31.443668419022938}, {"x"=-0.338726307, "y"=-31.443668419022938}, {"x"=-0.338726307, "y"=-31.443668419022938}, {"x"=-0.338726307, "y"=-31.443668419022938}, {"x"=-0.338726307, "y"=-31.443668419022938}, {"x"=-0.338726307, "y"=-31.443668419022938}, {"x"=-0.338726307, "y"=-31.443668419022938}, {"x"=-0.338726307, "y"=-31.443668419022938}, {"x"=-0.338726307, "y"=-31.443668419022938}, {"x"=-0.338726307, "y"=-31.443668419022938}, {"x"=-0.338726307, "y"=-31.443668419022938}, {"x"=-0.338726307, "y"=-31.443668419022938}, {"x"=-0.338726307, "y"=-31.443668419022938}, {"x"=-0.338726307, "y"=-31.443668419022938}, {"x"=-0.338726307, "y"=-31.443668419022938}, {"x"=-0.338726307, "y"=-31.443668419022938}, {"x"=-0.338726307, "y"=-31.443668419022938}, {"x"=-0.338726307, "y"=-31.443668419022938}, {"x"=-0.338726307, "y"=-31.443668419022938}, {"x"=-0.338726307, "y"=-31.443668419022938}, {"x"=-0.338726307, "y"=-31.443668419022938}, {"x"=-0.338726307, "y"=-31.443668419022938}, {"x"=-0.338726307, "y"=-31.443668419022938}, {"x"=-0.338726307, "y"=-31.443668419022938}, {"x"=-0.338726307, "y"=-31.443668419022938}, {"x"=-0.338726307, "y"=-31.443668419022938}, {"x"=-0.338726307, "y"=-31.443668419022938}, {"x"=-0.338726307, "y"=-31.443668419022938}, {"x"=-0.338726307, "y"=-31.443668419022938}, {"x"=-0.338726307, "y"=-31.443668419022938}, {"x"=-0.338726307, "y"=-31.443668419022938}, {"x"=-0.338726307, "y"=-31.443668419022938}, {"x"=-0.338726307, "y"=-31.443668419022938}, {"x"=-0.338726307, "y"=-31.443668419022938}, {"x"=-0.338726307, "y"=-31.443668419022938}, {"x"=-0.338726307, "y"=-31.443668419022938}, {"x"=-0.338726307, "y"=-31.443668419022938}, {"x"=-0.338726307, "y"=-31.443668419022938}, {"x"=-0.338726307, "y"=-31.443668419022938}, {"x"=-0.338726307, "y"=-31.443668419022938}, {"x"=-0.338726307, "y"=-31.443668419022938}, {"x"=-0.338726307, "y"=-31.443668419022938}, {"x"=-0.338726307, "y"=-31.443668419022938}, {"x"=-0.338726307, "y"=-31.443668419022938}, {"x"=-0.338726307, "y"=-31.443668419022938}, {"x"=-0.338726307, "y"=-31.443668419022938}, {"x"=-0.338726307, "y"=-31.443668419022938}, {"x"=-0.338726307, "y"=-31.443668419022938}, {"x"=-0.338726307, "y"=-31.443668419022938}, {"x"=-0.338726307, "y"=-31.443668419022938}, {"x"=-0.338726307, "y"=-31.443668419022938}, {"x"=-0.338726307, "y"=-31.443668419022938}, {"x"=-0.338726307, "y"=-31.443668419022938}, {"x"=-0.338726307, "y"=-31.443668419022938}, {"x"=-0.338726307, "y"=-31.443668419022938}, {"x"=-0.338726307, "y"=-31.443668419022938}, {"x"=-0.338726307, "y"=-31.443668419022938}, {"x"=-0.338726307, "y"=-31.443668419022938}, {"x"=-0.338726307, "y"=-31.443668419022938}, {"x"=-0.338726307, "y"=-31.443668419022938}, {"x"=-0.338726307, "y"=-31.443668419022938}, {"x"=-0.338726307, "y"=-31.443668419022938}, {"x"=-0.338726307, "y"=-31.443668419022938}, {"x"=-0.338726307, "y"=-31.443668419022938}, {"x"=-0.338726307, "y"=-31.443668419022938}, {"x"=-0.338726307, "y"=-31.443668419022938}, {"x"=-0.338726307, "y"=-31.443668419022938}, {"x"=-0.338726307, "y"=-31.443668419022938}, {"x"=-0.338726307, "y"=-31.443668419022938}, {"x"=-0.338726307, "y"=-31.443668419022938}, {"x"=-0.338726307, "y"=-31.443668419022938}, {"x"=-0.338726307, "y"=-31.443668419022938}, {"x"=-0.338726307, "y"=-31.443668419022938}, {"x"=-0.338726307, "y"=-31.443668419022938}, {"x"=-0.338726307, "y"=-31.443668419022938}, {"x"=-0.338726307, "y"=-31.443668419022938}, {"x"=-0.338726307, "y"=-31.443668419022938}, {"x"=-0.338726307, "y"=-31.443668419022938}, {"x"=-0.338726307, "y"=-31.443668419022938}, {"x"=-0.338726307, "y"=-31.443668419022938}, {"x"=-0.338726307, "y"=-31.443668419022938}, {"x"=-0.338726307, "y"=-31.443668419022938}, {"x"=-0.338726307, "y"=-31.443668419022938}, {"x"=-0.338726307, "y"=-31.443668419022938}, {"x"=-0.338726307, "y"=-31.443668419022938}, {"x"=-0.338726307, "y"=-31.443668419022938}, {"x"=-0.338726307, "y"=-31.443668419022938}, {"x"=-0.338726307, "y"=-31.443668419022938}, {"x"=-0.338726307, "y"=-31.443668419022938}, {"x"=-0.338726307, "y"=-31.443668419022938}, {"x"=-0.338726307, "y"=-31.443668419022938}, {"x"=-0.338726307, "y"=-31.443668419022938}, {"x"=-0.338726307, "y"=-31.443668419022938}, {"x"=-0.338726307, "y"=-31.443668419022938}, {"x"=-0.338726307, "y"=-31.443668419022938}, {"x"=-0.338726307, "y"=-31.443668419022938}, {"x"=-0.338726307, "y"=-31.443668419022938}, {"x"=-0.338726307, "y"=-31.443668419022938}, {"x"=-0.338726307, "y"=-31.443668419022938}, {"x"=-0.338726307, "y"=-31.443668419022938}, {"x"=-0.338726307, "y"=-31.443668419022938}, {"x"=-0.338726307, "y"=-31.443668419022938}, {"x"=-0.338726307, "y"=-31.443668419022938}, {"x"=-0.338726307, "y"=-31.443668419022938}, {"x"=-0.338726307, "y"=-31.443668419022938}, {"x"=-0.338726307, "y"=-31.443668419022938}, {"x"=-0.338726307, "y"=-31.443668419022938}, {"x"=-0.338726307, "y"=-31.443668419022938}, {"x"=-0.338726307, "y"=-31.443668419022938}, {"x"=-0.338726307, "y"=-31.443668419022938}, {"x"=-0.338726307, "y"=-31.443668419022938}, {"x"=-0.338726307, "y"=-31.443668419022938}, {"x"=-0.338726307, "y"=-31.443668419022938}, {"x"=-0.338726307, "y"=-31.443668419022938}, {"x"=-0.338726307, "y"=-31.443668419022938}, {"x"=-0.338726307, "y"=-31.443668419022938}, {"x"=-0.338726307, "y"=-31.443668419022938}, {"x"=-0.338726307, "y"=-31.443668419022938}, {"x"=-0.338726307, "y"=-31.443668419022938}, {"x"=-0.338726307, "y"=-31.443668419022938}, {"x"=-0.338726307, "y"=-31.443668419022938}, {"x"=-0.338726307, "y"=-31.443668419022938}, {"x"=-0.338726307, "y"=-31.443668419022938}, {"x"=-0.338726307, "y"=-31.443668419022938}, {"x"=-0.338726307, "y"=-31.443668419022938}, {"x"=-0.338726307, "y"=-31.443668419022938}, {"x"=-0.338726307, "y"=-31.443668419022938}, {"x"=-0.338726307, "y"=-31.443668419022938}, {"x"=-0.338726307, "y"=-31.443668419022938}, {"x"=-0.338726307, "y"=-31.443668419022938}, {"x"=-0.338726307, "y"=-31.443668419022938}, {"x"=-0.338726307, "y"=-31.443668419022938}, {"x"=-0.338726307, "y"=-31.443668419022938}, {"x"=-0.338726307, "y"=-31.443668419022938}, {"x"=-0.338726307, "y"=-31.443668419022938}, {"x"=-0.338726307, "y"=-31.443668419022938}, {"x"=-0.338726307, "y"=-31.443668419022938}, {"x"=-0.338726307, "y"=-31.443668419022938}, {"x"=-0.338726307, "y"=-31.443668419022938}, {"x"=-0.338726307, "y"=-31.443668419022938}, {"x"=-0.338726307, "y"=-31.443668419022938}, {"x"=-0.338726307, "y"=-31.443668419022938}, {"x"=-0.338726307, "y"=-31.443668419022938}, {"x"=-0.338726307, "y"=-31.443668419022938}, {"x"=-0.338726307, "y"=-31.443668419022938}, {"x"=-0.338726307, "y"=-31.443668419022938}, {"x"=-0.338726307, "y"=-31.443668419022938}, {"x"=-0.338726307, "y"=-31.443668419022938}, {"x"=-0.338726307, "y"=-31.443668419022938}, {"x"=-0.338726307, "y"=-31.443668419022938}, {"x"=-0.338726307, "y"=-31.443668419022938}, {"x"=-0.338726307, "y"=-31.443668419022938}, {"x"=-0.338726307, "y"=-31.443668419022938}, {"x"=-0.338726307, "y"=-31.443668419022938}, {"x"=-0.338726307, "y"=-31.443668419022938}, {"x"=-0.338726307, "y"=-31.443668419022938}, {"x"=-0.338726307, "y"=-31.443668419022938}, {"x"=-0.338726307, "y"=-31.443668419022938}, {"x"=-0.338726307, "y"=-31.443668419022938}, {"x"=-0.338726307, "y"=-31.443668419022938}, {"x"=-0.338726307, "y"=-31.443668419022938}, {"x"=-0.338726307, "y"=-31.443668419022938}, {"x"=-0.338726307, "y"=-31.443668419022938}, {"x"=-0.338726307, "y"=-31.443668419022938}, {"x"=-0.338726307, "y"=-31.443668419022938}, {"x"=-0.338726307, "y"=-31.443668419022938}, {"x"=-0.338726307, "y"=-31.443668419022938}, {"x"=-0.338726307, "y"=-31.443668419022938}, {"x"=-0.338726307, "y"=-31.443668419022938}, {"x"=-0.338726307, "y"=-31.443668419022938}, {"x"=-0.338726307, "y"=-31.443668419022938}, {"x"=-0.338726307, "y"=-31.443668419022938}, {"x"=-0.338726307, "y"=-31.443668419022938}, {"x"=-0.338726307, "y"=-31.443668419022938}, {"x"=-0.338726307, "y"=-31.443668419022938}, {"x"=-0.338726307, "y"=-31.443668419022938}, {"x"=-0.338726307, "y"=-31.443668419022938}, {"x"=-0.338726307, "y"=-31.443668419022938}, {"x"=-0.338726307, "y"=-31.443668419022938}, {"x"=-0.338726307, "y"=-31.443668419022938}, {"x"=-0.338726307, "y"=-31.443668419022938}, {"x"=-0.338726307, "y"=-31.443668419022938}, {"x"=-0.338726307, "y"=-31.443668419022938}, {"x"=-0.338726307, "y"=-31.443668419022938}, {"x"=-0.338726307, "y"=-31.443668419022938}, {"x"=-0.338726307, "y"=-31.443668419022938}, {"x"=-0.338726307, "y"=-31.443668419022938}, {"x"=-0.338726307, "y"=-31.443668419022938}, {"x"=-0.338726307, "y"=-31.443668419022938}, {"x"=-0.338726307, "y"=-31.443668419022938}, {"x"=-0.338726307, "y"=-31.443668419022938}, {"x"=-0.338726307, "y"=-31.443668419022938}, {"x"=-0.338726307, "y"=-31.443668419022938}, {"x"=-0.338726307, "y"=-31.443668419022938}, {"x"=-0.338726307, "y"=-31.443668419022938}, {"x"=-0.338726307, "y"=-31.443668419022938}, {"x"=-0.338726307, "y"=-31.443668419022938}, {"x"=-0.338726307, "y"=-31.443668419022938}, {"x"=-0.338726307, "y"=-31.443668419022938}, {"x"=-0.338726307, "y"=-31.443668419022938}, {"x"=-0.338726307, "y"=-31.443668419022938}, {"x"=-0.338726307, "y"=-31.443668419022938}, {"x"=-0.338726307, "y"=-31.443668419022938}, {"x"=-0.338726307, "y"=-31.443668419022938}, {"x"=-0.338726307, "y"=-31.443668419022938}, {"x"=-0.338726307, "y"=-31.443668419022938}, {"x"=-0.338726307, "y"=-31.443668419022938}, {"x"=-0.338726307, "y"=-31.443668419022938}, {"x"=-0.338726307, "y"=-31.443668419022938}, {"x"=-0.338726307, "y"=-31.443668419022938}, {"x"=-0.338726307, "y"=-31.443668419022938}, {"x"=-0.338726307, "y"=-31.443668419022938}, {"x"=-0.338726307, "y"=-31.443668419022938}, {"x"=-0.338726307, "y"=-31.443668419022938}, {"x"=-0.338726307, "y"=-31.443668419022938}, {"x"=-0.338726307, "y"=-31.443668419022938}, {"x"=-0.338726307, "y"=-31.443668419022938}, {"x"=-0.338726307, "y"=-31.443668419022938}, {"x"=-0.338726307, "y"=-31.443668419022938}, {"x"=-0.338726307, "y"=-31.443668419022938}, {"x"=-0.338726307, "y"=-31.443668419022938}, {"x"=-0.338726307, "y"=-31.443668419022938}, {"x"=-0.338726307, "y"=-31.443668419022938}, {"x"=-0.338726307, "y"=-31.443668419022938}, {"x"=-0.338726307, "y"=-31.443668419022938}, {"x"=-0.338726307, "y"=-31.443668419022938}, {"x"=-0.338726307, "y"=-31.443668419022938}, {"x"=-0.338726307, "y"=-31.443668419022938}, {"x"=-0.338726307, "y"=-31.443668419022938}, {"x"=-0.338726307, "y"=-31.443668419022938}, {"x"=-0.338726307, "y"=-31.443668419022938}, {"x"=-0.338726307, "y"=-31.443668419022938}, {"x"=-0.338726307, "y"=-31.443668419022938}, {"x"=-0.338726307, "y"=-31.443668419022938}, {"x"=-0.338726307, "y"=-31.443668419022938}, {"x"=-0.338726307, "y"=-31.443668419022938}, {"x"=-0.338726307, "y"=-31.443668419022938}, {"x"=-0.338726307, "y"=-31.443668419022938}, {"x"=-0.338726307, "y"=-31.443668419022938}, {"x"=-0.338726307, "y"=-31.443668419022938}, {"x"=-0.338726307, "y"=-31.443668419022938}, {"x"=-0.338726307, "y"=-31.443668419022938}, {"x"=-0.338726307, "y"=-31.443668419022938}, {"x"=-0.338726307, "y"=-31.443668419022938}, {"x"=-0.338726307, "y"=-31.443668419022938}, {"x"=-0.338726307, "y"=-31.443668419022938}, {"x"=-0.338726307, "y"=-31.443668419022938}, {"x"=-0.338726307, "y"=-31.443668419022938}, {"x"=-0.338726307, "y"=-31.443668419022938}, {"x"=-0.338726307, "y"=-31.443668419022938}, {"x"=-0.338726307, "y"=-31.443668419022938}, {"x"=-0.338726307, "y"=-31.443668419022938}, {"x"=-0.338726307, "y"=-31.443668419022938}, {"x"=-0.338726307, "y"=-31.443668419022938}, {"x"=-0.338726307, "y"=-31.443668419022938}, {"x"=-0.338726307, "y"=-31.443668419022938}, {"x"=-0.338726307, "y"=-31.443668419022938}, {"x"=-0.338726307, "y"=-31.443668419022938}, {"x"=-0.338726307, "y"=-31.443668419022938}, {"x"=-0.338726307, "y"=-31.443668419022938}, {"x"=-0.338726307, "y"=-31.443668419022938}, {"x"=-0.338726307, "y"=-31.443668419022938}, {"x"=-0.338726307, "y"=-31.443668419022938}, {"x"=-0.338726307, "y"=-31.443668419022938}, {"x"=-0.338726307, "y"=-31.443668419022938}, {"x"=-0.338726307, "y"=-31.443668419022938}, {"x"=-0.338726307, "y"=-31.443668419022938}, {"x"=-0.338726307, "y"=-31.443668419022938}, {"x"=-0.338726307, "y"=-31.443668419022938}, {"x"=-0.338726307, "y"=-31.443668419022938}, {"x"=-0.338726307, "y"=-31.443668419022938}, {"x"=-0.338726307, "y"=-31.443668419022938}, {"x"=-0.338726307, "y"=-31.443668419022938}, {"x"=-0.338726307, "y"=-31.443668419022938}, {"x"=-0.338726307, "y"=-31.443668419022938}, {"x"=-0.338726307, "y"=-31.443668419022938}, {"x"=-0.338726307, "y"=-31.443668419022938}, {"x"=-0.338726307, "y"=-31.443668419022938}, {"x"=-0.338726307, "y"=-31.443668419022938}, {"x"=-0.338726307, "y"=-31.443668419022938}, {"x"=-0.338726307, "y"=-31.443668419022938}, {"x"=-0.338726307, "y"=-31.443668419022938}, {"x"=-0.338726307, "y"=-31.443668419022938}, {"x"=-0.338726307, "y"=-31.443668419022938}, {"x"=-0.338726307, "y"=-31.443668419022938}, {"x"=-0.338726307, "y"=-31.443668419022938}, {"x"=-0.338726307, "y"=-31.443668419022938}, {"x"=-0.338726307, "y"=-31.443668419022938}, {"x"=-0.338726307, "y"=-31.443668419022938}, {"x"=-0.338726307, "y"=-31.443668419022938}, {"x"=-0.338726307, "y"=-31.443668419022938}, {"x"=-0.338726307, "y"=-31.443668419022938}, {"x"=-0.338726307, "y"=-31.443668419022938}, {"x"=-0.338726307, "y"=-31.443668419022938}, {"x"=-0.338726307, "y"=-31.443668419022938}, {"x"=-0.338726307, "y"=-31.443668419022938}, {"x"=-0.338726307, "y"=-31.443668419022938}, {"x"=-0.338726307, "y"=-31.443668419022938}, {"x"=-0.338726307, "y"=-31.443668419022938}, {"x"=-0.338726307, "y"=-31.443668419022938}, {"x"=-0.338726307, "y"=-31.443668419022938}, {"x"=-0.338726307, "y"=-31.443668419022938}, {"x"=-0.338726307, "y"=-31.443668419022938}, {"x"=-0.338726307, "y"=-31.443668419022938}, {"x"=-0.338726307, "y"=-31.443668419022938}, {"x"=-0.338726307, "y"=-31.443668419022938}, {"x"=-0.338726307, "y"=-31.443668419022938}, {"x"=-0.338726307, "y"=-31.443668419022938}, {"x"=-0.338726307, "y"=-31.443668419022938}, {"x"=-0.338726307, "y"=-31.443668419022938}, {"x"=-0.338726307, "y"=-31.443668419022938}, {"x"=-0.338726307, "y"=-31.443668419022938}, {"x"=-0.338726307, "y"=-31.443668419022938}, {"x"=-0.338726307, "y"=-31.443668419022938}, {"x"=-0.338726307, "y"=-31.443668419022938}, {"x"=-0.338726307, "y"=-31.443668419022938}, {"x"=-0.338726307, "y"=-31.443668419022938}, {"x"=-0.338726307, "y"=-31.443668419022938}, {"x"=-0.338726307, "y"=-31.443668419022938}, {"x"=-0.338726307, "y"=-31.443668419022938}, {"x"=-0.338726307, "y"=-31.443668419022938}, {"x"=-0.338726307, "y"=-31.443668419022938}, {"x"=-0.338726307, "y"=-31.443668419022938}, {"x"=-0.338726307, "y"=-31.443668419022938}, {"x"=-0.338726307, "y"=-31.443668419022938}, {"x"=-0.338726307, "y"=-31.443668419022938}, {"x"=-0.338726307, "y"=-31.443668419022938}, {"x"=-0.338726307, "y"=-31.443668419022938}, {"x"=-0.338726307, "y"=-31.443668419022938}, {"x"=-0.338726307, "y"=-31.443668419022938}, {"x"=-0.338726307, "y"=-31.443668419022938}, {"x"=-0.338726307, "y"=-31.443668419022938}, {"x"=-0.338726307, "y"=-31.443668419022938}, {"x"=-0.338726307, "y"=-31.443668419022938}, {"x"=-0.338726307, "y"=-31.443668419022938}, {"x"=-0.338726307, "y"=-31.443668419022938}, {"x"=-0.338726307, "y"=-31.443668419022938}, {"x"=-0.338726307, "y"=-31.443668419022938}, {"x"=-0.338726307, "y"=-31.443668419022938}, {"x"=-0.338726307, "y"=-31.443668419022938}, {"x"=-0.338726307, "y"=-31.443668419022938}, {"x"=-0.338726307, "y"=-31.443668419022938}, {"x"=-0.338726307, "y"=-31.443668419022938}, {"x"=-0.338726307, "y"=-31.443668419022938}, {"x"=-0.338726307, "y"=-31.443668419022938}, {"x"=-0.338726307, "y"=-31.443668419022938}, {"x"=-0.338726307, "y"=-31.443668419022938}, {"x"=-0.338726307, "y"=-31.443668419022938}, {"x"=-0.338726307, "y"=-31.443668419022938}, {"x"=-0.338726307, "y"=-31.443668419022938}, {"x"=-0.338726307, "y"=-31.443668419022938}, {"x"=-0.338726307, "y"=-31.443668419022938}, {"x"=-0.338726307, "y"=-31.443668419022938}, {"x"=-0.338726307, "y"=-31.443668419022938}, {"x"=-0.338726307, "y"=-31.443668419022938}, {"x"=-0.338726307, "y"=-31.443668419022938}, {"x"=-0.338726307, "y"=-31.443668419022938}, {"x"=-0.338726307, "y"=-31.443668419022938}, {"x"=-0.338726307, "y"=-31.443668419022938}, {"x"=-0.338726307, "y"=-31.443668419022938}, {"x"=-0.338726307, "y"=-31.443668419022938}, {"x"=-0.338726307, "y"=-31.443668419022938}, {"x"=-0.338726307, "y"=-31.443668419022938}, {"x"=-0.338726307, "y"=-31.443668419022938}, {"x"=-0.338726307, "y"=-31.443668419022938}, {"x"=-0.338726307, "y"=-31.443668419022938}, {"x"=-0.338726307, "y"=-31.443668419022938}, {"x"=-0.338726307, "y"=-31.443668419022938}, {"x"=-0.338726307, "y"=-31.443668419022938}, {"x"=-0.338726307, "y"=-31.443668419022938}, {"x"=-0.338726307, "y"=-31.443668419022938}, {"x"=-0.338726307, "y"=-31.443668419022938}, {"x"=-0.338726307, "y"=-31.443668419022938}, {"x"=-0.338726307, "y"=-31.443668419022938}, {"x"=-0.338726307, "y"=-31.443668419022938}, {"x"=-0.338726307, "y"=-31.443668419022938}, {"x"=-0.338726307, "y"=-31.443668419022938}, {"x"=-0.338726307, "y"=-31.443668419022938}, {"x"=-0.338726307, "y"=-31.443668419022938}, {"x"=-0.338726307, "y"=-31.443668419022938}, {"x"=-0.338726307, "y"=-31.443668419022938}, {"x"=-0.338726307, "y"=-31.443668419022938}, {"x"=-0.338726307, "y"=-31.443668419022938}, {"x"=-0.338726307, "y"=-31.443668419022938}, {"x"=-0.338726307, "y"=-31.443668419022938}, {"x"=-0.338726307, "y"=-31.443668419022938}, {"x"=-0.338726307, "y"=-31.443668419022938}, {"x"=-0.338726307, "y"=-31.443668419022938}, {"x"=-0.338726307, "y"=-31.443668419022938}, {"x"=-0.338726307, "y"=-31.443668419022938}, {"x"=-0.338726307, "y"=-31.443668419022938}, {"x"=-0.338726307, "y"=-31.443668419022938}, {"x"=-0.338726307, "y"=-31.443668419022938}, {"x"=-0.338726307, "y"=-31.443668419022938}, {"x"=-0.338726307, "y"=-31.443668419022938}, {"x"=-0.338726307, "y"=-31.443668419022938}, {"x"=-0.338726307, "y"=-31.443668419022938}, {"x"=-0.338726307, "y"=-31.443668419022938}, {"x"=-0.338726307, "y"=-31.443668419022938}, {"x"=-0.338726307, "y"=-31.443668419022938}, {"x"=-0.338726307, "y"=-31.443668419022938}, {"x"=-0.338726307, "y"=-31.443668419022938}, {"x"=-0.338726307, "y"=-31.443668419022938}, {"x"=-0.338726307, "y"=-31.443668419022938}, {"x"=-0.338726307, "y"=-31.443668419022938}, {"x"=-0.338726307, "y"=-31.443668419022938}, {"x"=-0.338726307, "y"=-31.443668419022938}, {"x"=-0.338726307, "y"=-31.443668419022938}, {"x"=-0.338726307, "y"=-31.443668419022938}, {"x"=-0.338726307, "y"=-31.443668419022938}, {"x"=-0.338726307, "y"=-31.443668419022938}, {"x"=-0.338726307, "y"=-31.443668419022938}, {"x"=-0.338726307, "y"=-31.443668419022938}, {"x"=-0.338726307, "y"=-31.443668419022938}, {"x"=-0.338726307, "y"=-31.443668419022938}, {"x"=-0.338726307, "y"=-31.443668419022938}, {"x"=-0.338726307, "y"=-31.443668419022938}, {"x"=-0.338726307, "y"=-31.443668419022938}, {"x"=-0.338726307, "y"=-31.443668419022938}, {"x"=-0.338726307, "y"=-31.443668419022938}, {"x"=-0.338726307, "y"=-31.443668419022938}, {"x"=-0.338726307, "y"=-31.443668419022938}, {"x"=-0.338726307, "y"=-31.443668419022938}, {"x"=-0.338726307, "y"=-31.443668419022938}, {"x"=-0.338726307, "y"=-31.443668419022938}, {"x"=-0.338726307, "y"=-31.443668419022938}, {"x"=-0.338726307, "y"=-31.443668419022938}, {"x"=-0.338726307, "y"=-31.443668419022938}, {"x"=-0.338726307, "y"=-31.443668419022938}, {"x"=-0.338726307, "y"=-31.443668419022938}, {"x"=-0.338726307, "y"=-31.443668419022938}, {"x"=-0.338726307, "y"=-31.443668419022938}, {"x"=-0.338726307, "y"=-31.443668419022938}, {"x"=-0.338726307, "y"=-31.443668419022938}, {"x"=-0.338726307, "y"=-31.443668419022938}, {"x"=-0.338726307, "y"=-31.443668419022938}, {"x"=-0.338726307, "y"=-31.443668419022938}, {"x"=-0.338726307, "y"=-31.443668419022938}, {"x"=-0.338726307, "y"=-31.443668419022938}, {"x"=-0.338726307, "y"=-31.443668419022938}, {"x"=-0.338726307, "y"=-31.443668419022938}, {"x"=-0.338726307, "y"=-31.443668419022938}, {"x"=-0.338726307, "y"=-31.443668419022938}, {"x"=-0.338726307, "y"=-31.443668419022938}, {"x"=-0.338726307, "y"=-31.443668419022938}, {"x"=-0.338726307, "y"=-31.443668419022938}, {"x"=-0.338726307, "y"=-31.443668419022938}, {"x"=-0.338726307, "y"=-31.443668419022938}, {"x"=-0.338726307, "y"=-31.443668419022938}, {"x"=-0.338726307, "y"=-31.443668419022938}, {"x"=-0.338726307, "y"=-31.443668419022938}, {"x"=-0.338726307, "y"=-31.443668419022938}, {"x"=-0.338726307, "y"=-31.443668419022938}, {"x"=-0.338726307, "y"=-31.443668419022938}, {"x"=-0.338726307, "y"=-31.443668419022938}, {"x"=-0.338726307, "y"=-31.443668419022938}, {"x"=-0.338726307, "y"=-31.443668419022938}, {"x"=-0.338726307, "y"=-31.443668419022938}, {"x"=-0.338726307, "y"=-31.443668419022938}, {"x"=-0.338726307, "y"=-31.443668419022938}, {"x"=-0.338726307, "y"=-31.443668419022938}, {"x"=-0.338726307, "y"=-31.443668419022938}, {"x"=-0.338726307, "y"=-31.443668419022938}, {"x"=-0.338726307, "y"=-31.443668419022938}, {"x"=-0.338726307, "y"=-31.443668419022938}, {"x"=-0.338726307, "y"=-31.443668419022938}, {"x"=-0.338726307, "y"=-31.443668419022938}, {"x"=-0.338726307, "y"=-31.443668419022938}, {"x"=-0.338726307, "y"=-31.443668419022938}, {"x"=-0.338726307, "y"=-31.443668419022938}, {"x"=-0.338726307, "y"=-31.443668419022938}, {"x"=-0.338726307, "y"=-31.443668419022938}, {"x"=-0.338726307, "y"=-31.443668419022938}, {"x"=-0.338726307, "y"=-31.443668419022938}, {"x"=-0.338726307, "y"=-31.443668419022938}, {"x"=-0.338726307, "y"=-31.443668419022938}, {"x"=-0.338726307, "y"=-31.443668419022938}, {"x"=-0.338726307, "y"=-31.443668419022938}, {"x"=-0.338726307, "y"=-31.443668419022938}, {"x"=-0.338726307, "y"=-31.443668419022938}, {"x"=-0.338726307, "y"=-31.443668419022938}, {"x"=-0.338726307, "y"=-31.443668419022938}, {"x"=-0.336933848, "y"=-31.687398408578932}, {"x"=-0.335312612, "y"=-31.81384306962391}, {"x"=-0.333588895, "y"=-31.814611553058327}, {"x"=-0.331523407, "y"=-31.619710251749}, {"x"=-0.32981741, "y"=-31.388083851011785}, {"x"=-0.328028071, "y"=-31.193573995063158}, {"x"=-0.326401821, "y"=-31.151938553210528}, {"x"=-0.324984329, "y"=-31.13248132945212}, {"x"=-0.323264419, "y"=-31.255403678115563}, {"x"=-0.321215795, "y"=-31.18358732230867}, {"x"=-0.319429341, "y"=-31.213743248380514}, {"x"=-0.317705652, "y"=-31.24711869507252}, {"x"=-0.316252294, "y"=-31.330343101384567}, {"x"=-0.314273418, "y"=-31.34573660278746}, {"x"=-0.312616976, "y"=-31.404666549614237}, {"x"=-0.311250279, "y"=-31.462738084144487}, {"x"=-0.309309309, "y"=-31.499930900697308}, {"x"=-0.307867444, "y"=-31.46661460550039}, {"x"=-0.306006106, "y"=-31.53802276885712}, {"x"=-0.304098247, "y"=-31.56168757897241}, {"x"=-0.302632408, "y"=-31.586661654067818}, {"x"=-0.300806821, "y"=-31.69429873106421}, {"x"=-0.298836948, "y"=-31.777823127787805}, {"x"=-0.297571904, "y"=-31.62017429369452}, {"x"=-0.295886637, "y"=-31.73691111080999}, {"x"=-0.294614436, "y"=-31.47034212427606}, {"x"=-0.293054135, "y"=-31.6096301872449}, {"x"=-0.291070233, "y"=-31.60442025184292}, {"x"=-0.289213666, "y"=-31.677155969514594}, {"x"=-0.287506173, "y"=-31.663907476083885}, {"x"=-0.286004532, "y"=-31.793193852720535}, {"x"=-0.284008765, "y"=-31.865199602157134}, {"x"=-0.282480195, "y"=-31.95773422101328}, {"x"=-0.281034734, "y"=-32.027163726132656}, {"x"=-0.278962449, "y"=-32.10755575533051}, {"x"=-0.277211169, "y"=-32.256522548973514}, {"x"=-0.275869818, "y"=-32.34927004612998}, {"x"=-0.275858707, "y"=-30.741544920324372}, {"x"=-0.274265871, "y"=-30.749621176651807}, {"x"=-0.272790832, "y"=-30.685697544685272}, {"x"=-0.271063181, "y"=-30.71551069031757}, {"x"=-0.2691099, "y"=-30.878168505751063}, {"x"=-0.267199649, "y"=-30.983174218773573}, {"x"=-0.265874043, "y"=-31.02417619462207}, {"x"=-0.26388427, "y"=-31.128628437833633}, {"x"=-0.262478602, "y"=-31.183256969829074}, {"x"=-0.260488689, "y"=-31.356575438798753}, {"x"=-0.261151761, "y"=-29.04139971090095}, {"x"=-0.260207725, "y"=-28.904900989375047}, {"x"=-0.258501565, "y"=-28.628217133220407}, {"x"=-0.256827198, "y"=-28.599323338391198}, {"x"=-0.254823982, "y"=-28.807732796689834}, {"x"=-0.257024388, "y"=-12.557498454606375}, {"x"=-0.255086829, "y"=-25.819879895991118}, {"x"=-0.253267682, "y"=-25.64589927565081}, {"x"=-0.251461911, "y"=-25.858305111650743}, {"x"=-0.250102396, "y"=-25.881491064801253}, {"x"=-0.25231274, "y"=-18.97034535510902}, {"x"=-0.250012497, "y"=-22.998376832344686}, {"x"=-0.248991208, "y"=-22.086778356110106}, {"x"=-0.248949448, "y"=-19.088305394180544}, {"x"=-0.246512783, "y"=-19.39654251676086}, {"x"=-0.244667033, "y"=-19.644351286387284}, {"x"=-0.243755129, "y"=-22.00523188781722}, {"x"=-0.241992414, "y"=-20.20003869618346}, {"x"=-0.239839622, "y"=-27.414064594586257}, {"x"=-0.239282604, "y"=-17.1800117151204}, {"x"=-0.239071311, "y"=-15.636676906376605}, {"x"=-0.237169503, "y"=-15.637713704538129}, {"x"=-0.235139523, "y"=-15.627070497397005}, {"x"=-0.233476595, "y"=-15.628164028447836}, {"x"=-0.231414947, "y"=-15.607055010709452}, {"x"=-0.229720153, "y"=-15.626905099966917}, {"x"=-0.227508415, "y"=-15.637658728792582}, {"x"=-0.225529067, "y"=-15.595247006620788}, {"x"=-0.223780059, "y"=-15.645978310547974}, {"x"=-0.22195849, "y"=-15.851516475563567}, {"x"=-0.219702213, "y"=-16.186268830780307}, {"x"=-0.218086488, "y"=-16.207980688482966}, {"x"=-0.216224865, "y"=-16.443836271207775}, {"x"=-0.214102332, "y"=-16.698924698968135}, {"x"=-0.212315332, "y"=-16.65307668447819}, {"x"=-0.210746278, "y"=-16.647570487434987}, {"x"=-0.208862816, "y"=-16.40818470296183}, {"x"=-0.206678716, "y"=-16.25995911924522}, {"x"=-0.205282319, "y"=-16.155328462407144}, {"x"=-0.203265687, "y"=-16.115913611715634}, {"x"=-0.2015471, "y"=-16.162704625503345}, {"x"=-0.199490385, "y"=-16.273920531166386}, {"x"=-0.199987848, "y"=-13.657293833790169}, {"x"=-0.19790616, "y"=-12.247681682151477}, {"x"=-0.196052649, "y"=-12.233474933152753}, {"x"=-0.194518356, "y"=-12.199575132637067}, {"x"=-0.19240891, "y"=-12.203130042354495}, {"x"=-0.190259549, "y"=-12.160331057380922}, {"x"=-0.188408297, "y"=-12.136818748978692}, {"x"=-0.186784842, "y"=-12.124647264781446}, {"x"=-0.185015955, "y"=-12.099285003701898}, {"x"=-0.182885565, "y"=-12.027083411343195}, {"x"=-0.18075409, "y"=-11.963146010325628}, {"x"=-0.178960146, "y"=-11.925224456962443}, {"x"=-0.176972854, "y"=-12.321740426012932}, {"x"=-0.17499795, "y"=-12.298729698874375}, {"x"=-0.173542057, "y"=-12.28963830298726}, {"x"=-0.171253542, "y"=-13.780167130703385}, {"x"=-0.169640817, "y"=-13.67881522436341}, {"x"=-0.167536408, "y"=-13.279035230212866}, {"x"=-0.165963029, "y"=-12.654090983830391}, {"x"=-0.163859733, "y"=-12.266557712321813}, {"x"=-0.162155989, "y"=-12.041059469488694}, {"x"=-0.16020872, "y"=-11.967680243269623}, {"x"=-0.158036963, "y"=-11.937987666696385}, {"x"=-0.15598597, "y"=-11.87896479510058}, {"x"=-0.155628749, "y"=-9.867622982843738}, {"x"=-0.153581019, "y"=-9.855987491632385}, {"x"=-0.151648848, "y"=-9.841394665559763}, {"x"=-0.149635681, "y"=-9.827464996962604}, {"x"=-0.147979192, "y"=-9.813314478664438}, {"x"=-0.145805958, "y"=-9.788467131444659}, {"x"=-0.144300464, "y"=-9.77802475128812}, {"x"=-0.142056117, "y"=-9.758111126897195}, {"x"=-0.140047045, "y"=-9.750913614985409}, {"x"=-0.138373454, "y"=-9.730787285232527}, {"x"=-0.136218379, "y"=-9.7123359680795}, {"x"=-0.134380383, "y"=-9.706943175202188}, {"x"=-0.132730532, "y"=-9.683489919672118}, {"x"=-0.130530307, "y"=-9.679373405248999}, {"x"=-0.128886387, "y"=-9.660026256076684}, {"x"=-0.126604636, "y"=-9.645155319278135}, {"x"=-0.124698588, "y"=-9.63200390693386}, {"x"=-0.122838797, "y"=-9.618219723182417}, {"x"=-0.121222399, "y"=-9.609306143847354}, {"x"=-0.118909575, "y"=-9.594134481712851}, {"x"=-0.117473761, "y"=-9.57768615270607}, {"x"=-0.115477579, "y"=-9.559831394561952}, {"x"=-0.110103078, "y"=-9.853801725713708}, {"x"=-0.108224772, "y"=-9.785489725331223}, {"x"=-0.105929355, "y"=-9.744056511483272}, {"x"=-0.104081993, "y"=-9.687758375648313}, {"x"=-0.102250618, "y"=-9.64453778782022}, {"x"=-0.100195133, "y"=-9.603012061093347}, {"x"=-0.098527987, "y"=-9.565131644119583}, {"x"=-0.0965328678, "y"=-9.531304812453788}, {"x"=-0.0942980484, "y"=-9.498858162931938}, {"x"=-0.0922350638, "y"=-9.467645383179287}, {"x"=-0.0906668875, "y"=-9.438656541481148}, {"x"=-0.088716553, "y"=-9.408184516535403}, {"x"=-0.0863975638, "y"=-9.381075347256218}, {"x"=-0.0846814559, "y"=-9.352956472251948}, {"x"=-0.083004609, "y"=-9.330056144735604}, {"x"=-0.0810332006, "y"=-9.30484974523799}, {"x"=-0.0788357726, "y"=-9.28312341103608}, {"x"=-0.0772556174, "y"=-9.254622939510874}, {"x"=-0.075003195, "y"=-9.239707754113846}, {"x"=-0.0734207429, "y"=-9.210458268226876}, {"x"=-0.0712544511, "y"=-9.199372841160555}, {"x"=-0.069650716, "y"=-9.177946053402758}, {"x"=-0.0674068702, "y"=-9.152724671265235}, {"x"=-0.0658028379, "y"=-9.134563658305348}, {"x"=-0.0638702748, "y"=-9.124918047931322}, {"x"=-0.0619029191, "y"=-9.096713517293592}, {"x"=-0.0597272892, "y"=-9.07634461508018}, {"x"=-0.0578072933, "y"=-9.05732409085398}, {"x"=-0.0562117806, "y"=-9.038383828425308}, {"x"=-0.05445193, "y"=-9.028159925841303}, {"x"=-0.0525810858, "y"=-9.010033628377995}, {"x"=-0.0502857008, "y"=-8.993484087714844}, {"x"=-0.0486110902, "y"=-8.978788007462112}, {"x"=-0.0464787007, "y"=-8.960562806217089}, {"x"=-0.0446874833, "y"=-8.943673289039905}]
  in  "invert":bool
  out "XY Graph  sec":cluster{"x":dbl, "y":dbl}[](graph)=[{"x"=-0.338726307, "y"=2.71843765}, {"x"=-0.338726307, "y"=2.71843765}, {"x"=-0.338726307, "y"=2.71843765}, {"x"=-0.338726307, "y"=2.71843765}, {"x"=-0.338726307, "y"=2.71843765}, {"x"=-0.338726307, "y"=2.71843765}, {"x"=-0.338726307, "y"=2.71843765}, {"x"=-0.338726307, "y"=2.71843765}, {"x"=-0.338726307, "y"=2.71843765}, {"x"=-0.338726307, "y"=2.71843765}, {"x"=-0.338726307, "y"=2.71843765}, {"x"=-0.338726307, "y"=2.71843765}, {"x"=-0.338726307, "y"=2.71843765}, {"x"=-0.338726307, "y"=2.71843765}, {"x"=-0.338726307, "y"=2.71843765}, {"x"=-0.338726307, "y"=2.71843765}, {"x"=-0.338726307, "y"=2.71843765}, {"x"=-0.338726307, "y"=2.71843765}, {"x"=-0.338726307, "y"=2.71843765}, {"x"=-0.338726307, "y"=2.71843765}, {"x"=-0.338726307, "y"=2.71843765}, {"x"=-0.338726307, "y"=2.71843765}, {"x"=-0.338726307, "y"=2.71843765}, {"x"=-0.338726307, "y"=2.71843765}, {"x"=-0.338726307, "y"=2.71843765}, {"x"=-0.338726307, "y"=2.71843765}, {"x"=-0.338726307, "y"=2.71843765}, {"x"=-0.338726307, "y"=2.71843765}, {"x"=-0.338726307, "y"=2.71843765}, {"x"=-0.338726307, "y"=2.71843765}, {"x"=-0.338726307, "y"=2.71843765}, {"x"=-0.338726307, "y"=2.71843765}, {"x"=-0.338726307, "y"=2.71843765}, {"x"=-0.338726307, "y"=2.71843765}, {"x"=-0.338726307, "y"=2.71843765}, {"x"=-0.338726307, "y"=2.71843765}, {"x"=-0.338726307, "y"=2.71843765}, {"x"=-0.338726307, "y"=2.71843765}, {"x"=-0.338726307, "y"=2.71843765}, {"x"=-0.338726307, "y"=2.71843765}, {"x"=-0.338726307, "y"=2.71843765}, {"x"=-0.338726307, "y"=2.71843765}, {"x"=-0.338726307, "y"=2.71843765}, {"x"=-0.338726307, "y"=2.71843765}, {"x"=-0.338726307, "y"=2.71843765}, {"x"=-0.338726307, "y"=2.71843765}, {"x"=-0.338726307, "y"=2.71843765}, {"x"=-0.338726307, "y"=2.71843765}, {"x"=-0.338726307, "y"=2.71843765}, {"x"=-0.338726307, "y"=2.71843765}, {"x"=-0.338726307, "y"=2.71843765}, {"x"=-0.338726307, "y"=2.71843765}, {"x"=-0.338726307, "y"=2.71843765}, {"x"=-0.338726307, "y"=2.71843765}, {"x"=-0.338726307, "y"=2.71843765}, {"x"=-0.338726307, "y"=2.71843765}, {"x"=-0.338726307, "y"=2.71843765}, {"x"=-0.338726307, "y"=2.71843765}, {"x"=-0.338726307, "y"=2.71843765}, {"x"=-0.338726307, "y"=2.71843765}, {"x"=-0.338726307, "y"=2.71843765}, {"x"=-0.338726307, "y"=2.71843765}, {"x"=-0.338726307, "y"=2.71843765}, {"x"=-0.338726307, "y"=2.71843765}, {"x"=-0.338726307, "y"=2.71843765}, {"x"=-0.338726307, "y"=2.71843765}, {"x"=-0.338726307, "y"=2.71843765}, {"x"=-0.338726307, "y"=2.71843765}, {"x"=-0.338726307, "y"=2.71843765}, {"x"=-0.338726307, "y"=2.71843765}, {"x"=-0.338726307, "y"=2.71843765}, {"x"=-0.338726307, "y"=2.71843765}, {"x"=-0.338726307, "y"=2.71843765}, {"x"=-0.338726307, "y"=2.71843765}, {"x"=-0.338726307, "y"=2.71843765}, {"x"=-0.338726307, "y"=2.71843765}, {"x"=-0.338726307, "y"=2.71843765}, {"x"=-0.338726307, "y"=2.71843765}, {"x"=-0.338726307, "y"=2.71843765}, {"x"=-0.338726307, "y"=2.71843765}, {"x"=-0.338726307, "y"=2.71843765}, {"x"=-0.338726307, "y"=2.71843765}, {"x"=-0.338726307, "y"=2.71843765}, {"x"=-0.338726307, "y"=2.71843765}, {"x"=-0.338726307, "y"=2.71843765}, {"x"=-0.338726307, "y"=2.71843765}, {"x"=-0.338726307, "y"=2.71843765}, {"x"=-0.338726307, "y"=2.71843765}, {"x"=-0.338726307, "y"=2.71843765}, {"x"=-0.338726307, "y"=2.71843765}, {"x"=-0.338726307, "y"=2.71843765}, {"x"=-0.338726307, "y"=2.71843765}, {"x"=-0.338726307, "y"=2.71843765}, {"x"=-0.338726307, "y"=2.71843765}, {"x"=-0.338726307, "y"=2.71843765}, {"x"=-0.338726307, "y"=2.71843765}, {"x"=-0.338726307, "y"=2.71843765}, {"x"=-0.338726307, "y"=2.71843765}, {"x"=-0.338726307, "y"=2.71843765}, {"x"=-0.338726307, "y"=2.71843765}, {"x"=-0.338726307, "y"=2.71843765}, {"x"=-0.338726307, "y"=2.71843765}, {"x"=-0.338726307, "y"=2.71843765}, {"x"=-0.338726307, "y"=2.71843765}, {"x"=-0.338726307, "y"=2.71843765}, {"x"=-0.338726307, "y"=2.71843765}, {"x"=-0.338726307, "y"=2.71843765}, {"x"=-0.338726307, "y"=2.71843765}, {"x"=-0.338726307, "y"=2.71843765}, {"x"=-0.338726307, "y"=2.71843765}, {"x"=-0.338726307, "y"=2.71843765}, {"x"=-0.338726307, "y"=2.71843765}, {"x"=-0.338726307, "y"=2.71843765}, {"x"=-0.338726307, "y"=2.71843765}, {"x"=-0.338726307, "y"=2.71843765}, {"x"=-0.338726307, "y"=2.71843765}, {"x"=-0.338726307, "y"=2.71843765}, {"x"=-0.338726307, "y"=2.71843765}, {"x"=-0.338726307, "y"=2.71843765}, {"x"=-0.338726307, "y"=2.71843765}, {"x"=-0.338726307, "y"=2.71843765}, {"x"=-0.338726307, "y"=2.71843765}, {"x"=-0.338726307, "y"=2.71843765}, {"x"=-0.338726307, "y"=2.71843765}, {"x"=-0.338726307, "y"=2.71843765}, {"x"=-0.338726307, "y"=2.71843765}, {"x"=-0.338726307, "y"=2.71843765}, {"x"=-0.338726307, "y"=2.71843765}, {"x"=-0.338726307, "y"=2.71843765}, {"x"=-0.338726307, "y"=2.71843765}, {"x"=-0.338726307, "y"=2.71843765}, {"x"=-0.338726307, "y"=2.71843765}, {"x"=-0.338726307, "y"=2.71843765}, {"x"=-0.338726307, "y"=2.71843765}, {"x"=-0.338726307, "y"=2.71843765}, {"x"=-0.338726307, "y"=2.71843765}, {"x"=-0.338726307, "y"=2.71843765}, {"x"=-0.338726307, "y"=2.71843765}, {"x"=-0.338726307, "y"=2.71843765}, {"x"=-0.338726307, "y"=2.71843765}, {"x"=-0.338726307, "y"=2.71843765}, {"x"=-0.338726307, "y"=2.71843765}, {"x"=-0.338726307, "y"=2.71843765}, {"x"=-0.338726307, "y"=2.71843765}, {"x"=-0.338726307, "y"=2.71843765}, {"x"=-0.338726307, "y"=2.71843765}, {"x"=-0.338726307, "y"=2.71843765}, {"x"=-0.338726307, "y"=2.71843765}, {"x"=-0.338726307, "y"=2.71843765}, {"x"=-0.338726307, "y"=2.71843765}, {"x"=-0.338726307, "y"=2.71843765}, {"x"=-0.338726307, "y"=2.71843765}, {"x"=-0.338726307, "y"=2.71843765}, {"x"=-0.338726307, "y"=2.71843765}, {"x"=-0.338726307, "y"=2.71843765}, {"x"=-0.338726307, "y"=2.71843765}, {"x"=-0.338726307, "y"=2.71843765}, {"x"=-0.338726307, "y"=2.71843765}, {"x"=-0.338726307, "y"=2.71843765}, {"x"=-0.338726307, "y"=2.71843765}, {"x"=-0.338726307, "y"=2.71843765}, {"x"=-0.338726307, "y"=2.71843765}, {"x"=-0.338726307, "y"=2.71843765}, {"x"=-0.338726307, "y"=2.71843765}, {"x"=-0.338726307, "y"=2.71843765}, {"x"=-0.338726307, "y"=2.71843765}, {"x"=-0.338726307, "y"=2.71843765}, {"x"=-0.338726307, "y"=2.71843765}, {"x"=-0.338726307, "y"=2.71843765}, {"x"=-0.338726307, "y"=2.71843765}, {"x"=-0.338726307, "y"=2.71843765}, {"x"=-0.338726307, "y"=2.71843765}, {"x"=-0.338726307, "y"=2.71843765}, {"x"=-0.338726307, "y"=2.71843765}, {"x"=-0.338726307, "y"=2.71843765}, {"x"=-0.338726307, "y"=2.71843765}, {"x"=-0.338726307, "y"=2.71843765}, {"x"=-0.338726307, "y"=2.71843765}, {"x"=-0.338726307, "y"=2.71843765}, {"x"=-0.338726307, "y"=2.71843765}, {"x"=-0.338726307, "y"=2.71843765}, {"x"=-0.338726307, "y"=2.71843765}, {"x"=-0.338726307, "y"=2.71843765}, {"x"=-0.338726307, "y"=2.71843765}, {"x"=-0.338726307, "y"=2.71843765}, {"x"=-0.338726307, "y"=2.71843765}, {"x"=-0.338726307, "y"=2.71843765}, {"x"=-0.338726307, "y"=2.71843765}, {"x"=-0.338726307, "y"=2.71843765}, {"x"=-0.338726307, "y"=2.71843765}, {"x"=-0.338726307, "y"=2.71843765}, {"x"=-0.338726307, "y"=2.71843765}, {"x"=-0.338726307, "y"=2.71843765}, {"x"=-0.338726307, "y"=2.71843765}, {"x"=-0.338726307, "y"=2.71843765}, {"x"=-0.338726307, "y"=2.71843765}, {"x"=-0.338726307, "y"=2.71843765}, {"x"=-0.338726307, "y"=2.71843765}, {"x"=-0.338726307, "y"=2.71843765}, {"x"=-0.338726307, "y"=2.71843765}, {"x"=-0.338726307, "y"=2.71843765}, {"x"=-0.338726307, "y"=2.71843765}, {"x"=-0.338726307, "y"=2.71843765}, {"x"=-0.338726307, "y"=2.71843765}, {"x"=-0.338726307, "y"=2.71843765}, {"x"=-0.338726307, "y"=2.71843765}, {"x"=-0.338726307, "y"=2.71843765}, {"x"=-0.338726307, "y"=2.71843765}, {"x"=-0.338726307, "y"=2.71843765}, {"x"=-0.338726307, "y"=2.71843765}, {"x"=-0.338726307, "y"=2.71843765}, {"x"=-0.338726307, "y"=2.71843765}, {"x"=-0.338726307, "y"=2.71843765}, {"x"=-0.338726307, "y"=2.71843765}, {"x"=-0.338726307, "y"=2.71843765}, {"x"=-0.338726307, "y"=2.71843765}, {"x"=-0.338726307, "y"=2.71843765}, {"x"=-0.338726307, "y"=2.71843765}, {"x"=-0.338726307, "y"=2.71843765}, {"x"=-0.338726307, "y"=2.71843765}, {"x"=-0.338726307, "y"=2.71843765}, {"x"=-0.338726307, "y"=2.71843765}, {"x"=-0.338726307, "y"=2.71843765}, {"x"=-0.338726307, "y"=2.71843765}, {"x"=-0.338726307, "y"=2.71843765}, {"x"=-0.338726307, "y"=2.71843765}, {"x"=-0.338726307, "y"=2.71843765}, {"x"=-0.338726307, "y"=2.71843765}, {"x"=-0.338726307, "y"=2.71843765}, {"x"=-0.338726307, "y"=2.71843765}, {"x"=-0.338726307, "y"=2.71843765}, {"x"=-0.338726307, "y"=2.71843765}, {"x"=-0.338726307, "y"=2.71843765}, {"x"=-0.338726307, "y"=2.71843765}, {"x"=-0.338726307, "y"=2.71843765}, {"x"=-0.338726307, "y"=2.71843765}, {"x"=-0.338726307, "y"=2.71843765}, {"x"=-0.338726307, "y"=2.71843765}, {"x"=-0.338726307, "y"=2.71843765}, {"x"=-0.338726307, "y"=2.71843765}, {"x"=-0.338726307, "y"=2.71843765}, {"x"=-0.338726307, "y"=2.71843765}, {"x"=-0.338726307, "y"=2.71843765}, {"x"=-0.338726307, "y"=2.71843765}, {"x"=-0.338726307, "y"=2.71843765}, {"x"=-0.338726307, "y"=2.71843765}, {"x"=-0.338726307, "y"=2.71843765}, {"x"=-0.338726307, "y"=2.71843765}, {"x"=-0.338726307, "y"=2.71843765}, {"x"=-0.338726307, "y"=2.71843765}, {"x"=-0.338726307, "y"=2.71843765}, {"x"=-0.338726307, "y"=2.71843765}, {"x"=-0.338726307, "y"=2.71843765}, {"x"=-0.338726307, "y"=2.71843765}, {"x"=-0.338726307, "y"=2.71843765}, {"x"=-0.338726307, "y"=2.71843765}, {"x"=-0.338726307, "y"=2.71843765}, {"x"=-0.338726307, "y"=2.71843765}, {"x"=-0.338726307, "y"=2.71843765}, {"x"=-0.338726307, "y"=2.71843765}, {"x"=-0.338726307, "y"=2.71843765}, {"x"=-0.338726307, "y"=2.71843765}, {"x"=-0.338726307, "y"=2.71843765}, {"x"=-0.338726307, "y"=2.71843765}, {"x"=-0.338726307, "y"=2.71843765}, {"x"=-0.338726307, "y"=2.71843765}, {"x"=-0.338726307, "y"=2.71843765}, {"x"=-0.338726307, "y"=2.71843765}, {"x"=-0.338726307, "y"=2.71843765}, {"x"=-0.338726307, "y"=2.71843765}, {"x"=-0.338726307, "y"=2.71843765}, {"x"=-0.338726307, "y"=2.71843765}, {"x"=-0.338726307, "y"=2.71843765}, {"x"=-0.338726307, "y"=2.71843765}, {"x"=-0.338726307, "y"=2.71843765}, {"x"=-0.338726307, "y"=2.71843765}, {"x"=-0.338726307, "y"=2.71843765}, {"x"=-0.338726307, "y"=2.71843765}, {"x"=-0.338726307, "y"=2.71843765}, {"x"=-0.338726307, "y"=2.71843765}, {"x"=-0.338726307, "y"=2.71843765}, {"x"=-0.338726307, "y"=2.71843765}, {"x"=-0.338726307, "y"=2.71843765}, {"x"=-0.338726307, "y"=2.71843765}, {"x"=-0.338726307, "y"=2.71843765}, {"x"=-0.338726307, "y"=2.71843765}, {"x"=-0.338726307, "y"=2.71843765}, {"x"=-0.338726307, "y"=2.71843765}, {"x"=-0.338726307, "y"=2.71843765}, {"x"=-0.338726307, "y"=2.71843765}, {"x"=-0.338726307, "y"=2.71843765}, {"x"=-0.338726307, "y"=2.71843765}, {"x"=-0.338726307, "y"=2.71843765}, {"x"=-0.338726307, "y"=2.71843765}, {"x"=-0.338726307, "y"=2.71843765}, {"x"=-0.338726307, "y"=2.71843765}, {"x"=-0.338726307, "y"=2.71843765}, {"x"=-0.338726307, "y"=2.71843765}, {"x"=-0.338726307, "y"=2.71843765}, {"x"=-0.338726307, "y"=2.71843765}, {"x"=-0.338726307, "y"=2.71843765}, {"x"=-0.338726307, "y"=2.71843765}, {"x"=-0.338726307, "y"=2.71843765}, {"x"=-0.338726307, "y"=2.71843765}, {"x"=-0.338726307, "y"=2.71843765}, {"x"=-0.338726307, "y"=2.71843765}, {"x"=-0.338726307, "y"=2.71843765}, {"x"=-0.338726307, "y"=2.71843765}, {"x"=-0.338726307, "y"=2.71843765}, {"x"=-0.338726307, "y"=2.71843765}, {"x"=-0.338726307, "y"=2.71843765}, {"x"=-0.338726307, "y"=2.71843765}, {"x"=-0.338726307, "y"=2.71843765}, {"x"=-0.338726307, "y"=2.71843765}, {"x"=-0.338726307, "y"=2.71843765}, {"x"=-0.338726307, "y"=2.71843765}, {"x"=-0.338726307, "y"=2.71843765}, {"x"=-0.338726307, "y"=2.71843765}, {"x"=-0.338726307, "y"=2.71843765}, {"x"=-0.338726307, "y"=2.71843765}, {"x"=-0.338726307, "y"=2.71843765}, {"x"=-0.338726307, "y"=2.71843765}, {"x"=-0.338726307, "y"=2.71843765}, {"x"=-0.338726307, "y"=2.71843765}, {"x"=-0.338726307, "y"=2.71843765}, {"x"=-0.338726307, "y"=2.71843765}, {"x"=-0.338726307, "y"=2.71843765}, {"x"=-0.338726307, "y"=2.71843765}, {"x"=-0.338726307, "y"=2.71843765}, {"x"=-0.338726307, "y"=2.71843765}, {"x"=-0.338726307, "y"=2.71843765}, {"x"=-0.338726307, "y"=2.71843765}, {"x"=-0.338726307, "y"=2.71843765}, {"x"=-0.338726307, "y"=2.71843765}, {"x"=-0.338726307, "y"=2.71843765}, {"x"=-0.338726307, "y"=2.71843765}, {"x"=-0.338726307, "y"=2.71843765}, {"x"=-0.338726307, "y"=2.71843765}, {"x"=-0.338726307, "y"=2.71843765}, {"x"=-0.338726307, "y"=2.71843765}, {"x"=-0.338726307, "y"=2.71843765}, {"x"=-0.338726307, "y"=2.71843765}, {"x"=-0.338726307, "y"=2.71843765}, {"x"=-0.338726307, "y"=2.71843765}, {"x"=-0.338726307, "y"=2.71843765}, {"x"=-0.338726307, "y"=2.71843765}, {"x"=-0.338726307, "y"=2.71843765}, {"x"=-0.338726307, "y"=2.71843765}, {"x"=-0.338726307, "y"=2.71843765}, {"x"=-0.338726307, "y"=2.71843765}, {"x"=-0.338726307, "y"=2.71843765}, {"x"=-0.338726307, "y"=2.71843765}, {"x"=-0.338726307, "y"=2.71843765}, {"x"=-0.338726307, "y"=2.71843765}, {"x"=-0.338726307, "y"=2.71843765}, {"x"=-0.338726307, "y"=2.71843765}, {"x"=-0.338726307, "y"=2.71843765}, {"x"=-0.338726307, "y"=2.71843765}, {"x"=-0.338726307, "y"=2.71843765}, {"x"=-0.338726307, "y"=2.71843765}, {"x"=-0.338726307, "y"=2.71843765}, {"x"=-0.338726307, "y"=2.71843765}, {"x"=-0.338726307, "y"=2.71843765}, {"x"=-0.338726307, "y"=2.71843765}, {"x"=-0.338726307, "y"=2.71843765}, {"x"=-0.338726307, "y"=2.71843765}, {"x"=-0.338726307, "y"=2.71843765}, {"x"=-0.338726307, "y"=2.71843765}, {"x"=-0.338726307, "y"=2.71843765}, {"x"=-0.338726307, "y"=2.71843765}, {"x"=-0.338726307, "y"=2.71843765}, {"x"=-0.338726307, "y"=2.71843765}, {"x"=-0.338726307, "y"=2.71843765}, {"x"=-0.338726307, "y"=2.71843765}, {"x"=-0.338726307, "y"=2.71843765}, {"x"=-0.338726307, "y"=2.71843765}, {"x"=-0.338726307, "y"=2.71843765}, {"x"=-0.338726307, "y"=2.71843765}, {"x"=-0.338726307, "y"=2.71843765}, {"x"=-0.338726307, "y"=2.71843765}, {"x"=-0.338726307, "y"=2.71843765}, {"x"=-0.338726307, "y"=2.71843765}, {"x"=-0.338726307, "y"=2.71843765}, {"x"=-0.338726307, "y"=2.71843765}, {"x"=-0.338726307, "y"=2.71843765}, {"x"=-0.338726307, "y"=2.71843765}, {"x"=-0.338726307, "y"=2.71843765}, {"x"=-0.338726307, "y"=2.71843765}, {"x"=-0.338726307, "y"=2.71843765}, {"x"=-0.338726307, "y"=2.71843765}, {"x"=-0.338726307, "y"=2.71843765}, {"x"=-0.338726307, "y"=2.71843765}, {"x"=-0.338726307, "y"=2.71843765}, {"x"=-0.338726307, "y"=2.71843765}, {"x"=-0.338726307, "y"=2.71843765}, {"x"=-0.338726307, "y"=2.71843765}, {"x"=-0.338726307, "y"=2.71843765}, {"x"=-0.338726307, "y"=2.71843765}, {"x"=-0.338726307, "y"=2.71843765}, {"x"=-0.338726307, "y"=2.71843765}, {"x"=-0.338726307, "y"=2.71843765}, {"x"=-0.338726307, "y"=2.71843765}, {"x"=-0.338726307, "y"=2.71843765}, {"x"=-0.338726307, "y"=2.71843765}, {"x"=-0.338726307, "y"=2.71843765}, {"x"=-0.338726307, "y"=2.71843765}, {"x"=-0.338726307, "y"=2.71843765}, {"x"=-0.338726307, "y"=2.71843765}, {"x"=-0.338726307, "y"=2.71843765}, {"x"=-0.338726307, "y"=2.71843765}, {"x"=-0.338726307, "y"=2.71843765}, {"x"=-0.338726307, "y"=2.71843765}, {"x"=-0.338726307, "y"=2.71843765}, {"x"=-0.338726307, "y"=2.71843765}, {"x"=-0.338726307, "y"=2.71843765}, {"x"=-0.338726307, "y"=2.71843765}, {"x"=-0.338726307, "y"=2.71843765}, {"x"=-0.338726307, "y"=2.71843765}, {"x"=-0.338726307, "y"=2.71843765}, {"x"=-0.338726307, "y"=2.71843765}, {"x"=-0.338726307, "y"=2.71843765}, {"x"=-0.338726307, "y"=2.71843765}, {"x"=-0.338726307, "y"=2.71843765}, {"x"=-0.338726307, "y"=2.71843765}, {"x"=-0.338726307, "y"=2.71843765}, {"x"=-0.338726307, "y"=2.71843765}, {"x"=-0.338726307, "y"=2.71843765}, {"x"=-0.338726307, "y"=2.71843765}, {"x"=-0.338726307, "y"=2.71843765}, {"x"=-0.338726307, "y"=2.71843765}, {"x"=-0.338726307, "y"=2.71843765}, {"x"=-0.338726307, "y"=2.71843765}, {"x"=-0.338726307, "y"=2.71843765}, {"x"=-0.338726307, "y"=2.71843765}, {"x"=-0.338726307, "y"=2.71843765}, {"x"=-0.338726307, "y"=2.71843765}, {"x"=-0.338726307, "y"=2.71843765}, {"x"=-0.338726307, "y"=2.71843765}, {"x"=-0.338726307, "y"=2.71843765}, {"x"=-0.338726307, "y"=2.71843765}, {"x"=-0.338726307, "y"=2.71843765}, {"x"=-0.338726307, "y"=2.71843765}, {"x"=-0.338726307, "y"=2.71843765}, {"x"=-0.338726307, "y"=2.71843765}, {"x"=-0.338726307, "y"=2.71843765}, {"x"=-0.338726307, "y"=2.71843765}, {"x"=-0.338726307, "y"=2.71843765}, {"x"=-0.338726307, "y"=2.71843765}, {"x"=-0.338726307, "y"=2.71843765}, {"x"=-0.338726307, "y"=2.71843765}, {"x"=-0.338726307, "y"=2.71843765}, {"x"=-0.338726307, "y"=2.71843765}, {"x"=-0.338726307, "y"=2.71843765}, {"x"=-0.338726307, "y"=2.71843765}, {"x"=-0.338726307, "y"=2.71843765}, {"x"=-0.338726307, "y"=2.71843765}, {"x"=-0.338726307, "y"=2.71843765}, {"x"=-0.338726307, "y"=2.71843765}, {"x"=-0.338726307, "y"=2.71843765}, {"x"=-0.338726307, "y"=2.71843765}, {"x"=-0.338726307, "y"=2.71843765}, {"x"=-0.338726307, "y"=2.71843765}, {"x"=-0.338726307, "y"=2.71843765}, {"x"=-0.338726307, "y"=2.71843765}, {"x"=-0.338726307, "y"=2.71843765}, {"x"=-0.338726307, "y"=2.71843765}, {"x"=-0.338726307, "y"=2.71843765}, {"x"=-0.338726307, "y"=2.71843765}, {"x"=-0.338726307, "y"=2.71843765}, {"x"=-0.338726307, "y"=2.71843765}, {"x"=-0.338726307, "y"=2.71843765}, {"x"=-0.338726307, "y"=2.71843765}, {"x"=-0.338726307, "y"=2.71843765}, {"x"=-0.338726307, "y"=2.71843765}, {"x"=-0.338726307, "y"=2.71843765}, {"x"=-0.338726307, "y"=2.71843765}, {"x"=-0.338726307, "y"=2.71843765}, {"x"=-0.338726307, "y"=2.71843765}, {"x"=-0.338726307, "y"=2.71843765}, {"x"=-0.338726307, "y"=2.71843765}, {"x"=-0.338726307, "y"=2.71843765}, {"x"=-0.338726307, "y"=2.71843765}, {"x"=-0.338726307, "y"=2.71843765}, {"x"=-0.338726307, "y"=2.71843765}, {"x"=-0.338726307, "y"=2.71843765}, {"x"=-0.338726307, "y"=2.71843765}, {"x"=-0.338726307, "y"=2.71843765}, {"x"=-0.338726307, "y"=2.71843765}, {"x"=-0.338726307, "y"=2.71843765}, {"x"=-0.338726307, "y"=2.71843765}, {"x"=-0.338726307, "y"=2.71843765}, {"x"=-0.338726307, "y"=2.71843765}, {"x"=-0.338726307, "y"=2.71843765}, {"x"=-0.338726307, "y"=2.71843765}, {"x"=-0.338726307, "y"=2.71843765}, {"x"=-0.338726307, "y"=2.71843765}, {"x"=-0.338726307, "y"=2.71843765}, {"x"=-0.338726307, "y"=2.71843765}, {"x"=-0.338726307, "y"=2.71843765}, {"x"=-0.338726307, "y"=2.71843765}, {"x"=-0.338726307, "y"=2.71843765}, {"x"=-0.338726307, "y"=2.71843765}, {"x"=-0.338726307, "y"=2.71843765}, {"x"=-0.338726307, "y"=2.71843765}, {"x"=-0.338726307, "y"=2.71843765}, {"x"=-0.338726307, "y"=2.71843765}, {"x"=-0.338726307, "y"=2.71843765}, {"x"=-0.338726307, "y"=2.71843765}, {"x"=-0.338726307, "y"=2.71843765}, {"x"=-0.338726307, "y"=2.71843765}, {"x"=-0.338726307, "y"=2.71843765}, {"x"=-0.338726307, "y"=2.71843765}, {"x"=-0.338726307, "y"=2.71843765}, {"x"=-0.338726307, "y"=2.71843765}, {"x"=-0.338726307, "y"=2.71843765}, {"x"=-0.338726307, "y"=2.71843765}, {"x"=-0.338726307, "y"=2.71843765}, {"x"=-0.338726307, "y"=2.71843765}, {"x"=-0.338726307, "y"=2.71843765}, {"x"=-0.338726307, "y"=2.71843765}, {"x"=-0.338726307, "y"=2.71843765}, {"x"=-0.338726307, "y"=2.71843765}, {"x"=-0.338726307, "y"=2.71843765}, {"x"=-0.338726307, "y"=2.71843765}, {"x"=-0.338726307, "y"=2.71843765}, {"x"=-0.338726307, "y"=2.71843765}, {"x"=-0.338726307, "y"=2.71843765}, {"x"=-0.338726307, "y"=2.71843765}, {"x"=-0.338726307, "y"=2.71843765}, {"x"=-0.338726307, "y"=2.71843765}, {"x"=-0.338726307, "y"=2.71843765}, {"x"=-0.338726307, "y"=2.71843765}, {"x"=-0.338726307, "y"=2.71843765}, {"x"=-0.338726307, "y"=2.71843765}, {"x"=-0.338726307, "y"=2.71843765}, {"x"=-0.338726307, "y"=2.71843765}, {"x"=-0.338726307, "y"=2.71843765}, {"x"=-0.338726307, "y"=2.71843765}, {"x"=-0.338726307, "y"=2.71843765}, {"x"=-0.338726307, "y"=2.71843765}, {"x"=-0.338726307, "y"=2.71843765}, {"x"=-0.338726307, "y"=2.71843765}, {"x"=-0.338726307, "y"=2.71843765}, {"x"=-0.338726307, "y"=2.71843765}, {"x"=-0.338726307, "y"=2.71843765}, {"x"=-0.338726307, "y"=2.71843765}, {"x"=-0.338726307, "y"=2.71843765}, {"x"=-0.338726307, "y"=2.71843765}, {"x"=-0.338726307, "y"=2.71843765}, {"x"=-0.338726307, "y"=2.71843765}, {"x"=-0.338726307, "y"=2.71843765}, {"x"=-0.338726307, "y"=2.71843765}, {"x"=-0.338726307, "y"=2.71843765}, {"x"=-0.338726307, "y"=2.71843765}, {"x"=-0.338726307, "y"=2.71843765}, {"x"=-0.338726307, "y"=2.71843765}, {"x"=-0.338726307, "y"=2.71843765}, {"x"=-0.338726307, "y"=2.71843765}, {"x"=-0.338726307, "y"=2.71843765}, {"x"=-0.338726307, "y"=2.71843765}, {"x"=-0.338726307, "y"=2.71843765}, {"x"=-0.338726307, "y"=2.71843765}, {"x"=-0.338726307, "y"=2.71843765}, {"x"=-0.338726307, "y"=2.71843765}, {"x"=-0.338726307, "y"=2.71843765}, {"x"=-0.338726307, "y"=2.71843765}, {"x"=-0.338726307, "y"=2.71843765}, {"x"=-0.338726307, "y"=2.71843765}, {"x"=-0.338726307, "y"=2.71843765}, {"x"=-0.338726307, "y"=2.71843765}, {"x"=-0.338726307, "y"=2.71843765}, {"x"=-0.338726307, "y"=2.71843765}, {"x"=-0.338726307, "y"=2.71843765}, {"x"=-0.338726307, "y"=2.71843765}, {"x"=-0.338726307, "y"=2.71843765}, {"x"=-0.338726307, "y"=2.71843765}, {"x"=-0.338726307, "y"=2.71843765}, {"x"=-0.338726307, "y"=2.71843765}, {"x"=-0.338726307, "y"=2.71843765}, {"x"=-0.338726307, "y"=2.71843765}, {"x"=-0.336933848, "y"=2.53841287}, {"x"=-0.335312612, "y"=0.957440033}, {"x"=-0.333588895, "y"=-2.11920563}, {"x"=-0.331523407, "y"=-3.29997227}, {"x"=-0.32981741, "y"=-2.50462157}, {"x"=-0.328028071, "y"=-0.600986385}, {"x"=-0.326401821, "y"=0.185229271}, {"x"=-0.324984329, "y"=-0.311110549}, {"x"=-0.323264419, "y"=0.0920550346}, {"x"=-0.321215795, "y"=0.285897603}, {"x"=-0.319429341, "y"=0.22674854}, {"x"=-0.317705652, "y"=0.419837853}, {"x"=-0.316252294, "y"=0.314007692}, {"x"=-0.314273418, "y"=0.420077193}, {"x"=-0.312616976, "y"=0.530936767}, {"x"=-0.311250279, "y"=0.248903901}, {"x"=-0.309309309, "y"=0.165523235}, {"x"=-0.307867444, "y"=0.389272628}, {"x"=-0.306006106, "y"=0.364371082}, {"x"=-0.304098247, "y"=0.357789935}, {"x"=-0.302632408, "y"=0.430571969}, {"x"=-0.300806821, "y"=0.337107933}, {"x"=-0.298836948, "y"=0.680734923}, {"x"=-0.297571904, "y"=0.937623806}, {"x"=-0.295886637, "y"=0.711285838}, {"x"=-0.294614436, "y"=0.423014721}, {"x"=-0.293054135, "y"=0.789236856}, {"x"=-0.291070233, "y"=0.58537723}, {"x"=-0.289213666, "y"=0.693597183}, {"x"=-0.287506173, "y"=0.621446269}, {"x"=-0.286004532, "y"=0.892992474}, {"x"=-0.284008765, "y"=0.661426689}, {"x"=-0.282480195, "y"=0.476718609}, {"x"=-0.281034734, "y"=0.885150794}, {"x"=-0.278962449, "y"=0.905555931}, {"x"=-0.277211169, "y"=0.952591217}, {"x"=-0.275869818, "y"=1.35292651}, {"x"=-0.275858707, "y"=0.668744253}, {"x"=-0.274265871, "y"=0.155038672}, {"x"=-0.272790832, "y"=0.659625967}, {"x"=-0.271063181, "y"=0.449749147}, {"x"=-0.2691099, "y"=0.645274129}, {"x"=-0.267199649, "y"=0.771423289}, {"x"=-0.265874043, "y"=0.769640096}, {"x"=-0.26388427, "y"=0.99062462}, {"x"=-0.262478602, "y"=1.2144784}, {"x"=-0.260488689, "y"=1.17029433}, {"x"=-0.261151761, "y"=0.577930014}, {"x"=-0.260207725, "y"=0.863591163}, {"x"=-0.258501565, "y"=0.433013753}, {"x"=-0.256827198, "y"=0.931273417}, {"x"=-0.254823982, "y"=2.74699644}, {"x"=-0.257024388, "y"=-2.34465656}, {"x"=-0.255086829, "y"=0.190576651}, {"x"=-0.253267682, "y"=0.289655606}, {"x"=-0.251461911, "y"=0.650823613}, {"x"=-0.250102396, "y"=2.47684618}, {"x"=-0.25231274, "y"=-1.20387603}, {"x"=-0.250012497, "y"=1.41505565}, {"x"=-0.248991208, "y"=0.707675098}, {"x"=-0.248949448, "y"=-0.58390308}, {"x"=-0.246512783, "y"=1.2636665}, {"x"=-0.244667033, "y"=0.163295648}, {"x"=-0.243755129, "y"=-10.9455898}, {"x"=-0.241992414, "y"=1.45615999}, {"x"=-0.239839622, "y"=12.7631946}, {"x"=-0.239282604, "y"=0.236264971}, {"x"=-0.239071311, "y"=-0.182707639}, {"x"=-0.237169503, "y"=-0.165837769}, {"x"=-0.235139523, "y"=-0.318912661}, {"x"=-0.233476595, "y"=-0.176520131}, {"x"=-0.231414947, "y"=-0.0611011856}, {"x"=-0.229720153, "y"=0.172041676}, {"x"=-0.227508415, "y"=-0.123725396}, {"x"=-0.225529067, "y"=0.2232642}, {"x"=-0.223780059, "y"=-0.039148826}, {"x"=-0.22195849, "y"=0.410138853}, {"x"=-0.219702213, "y"=0.990695309}, {"x"=-0.218086488, "y"=1.65893613}, {"x"=-0.216224865, "y"=1.67252742}, {"x"=-0.214102332, "y"=0.982262366}, {"x"=-0.212315332, "y"=-0.485409998}, {"x"=-0.210746278, "y"=-1.04161482}, {"x"=-0.208862816, "y"=-1.58423487}, {"x"=-0.206678716, "y"=-0.832278667}, {"x"=-0.205282319, "y"=-0.0643462524}, {"x"=-0.203265687, "y"=-0.24310895}, {"x"=-0.2015471, "y"=0.401973454}, {"x"=-0.199490385, "y"=0.972209636}, {"x"=-0.199987848, "y"=-0.847812845}, {"x"=-0.19790616, "y"=-0.155396713}, {"x"=-0.196052649, "y"=-0.214249789}, {"x"=-0.194518356, "y"=-0.307722264}, {"x"=-0.19240891, "y"=-0.265259967}, {"x"=-0.190259549, "y"=-0.190930548}, {"x"=-0.188408297, "y"=-0.291804041}, {"x"=-0.186784842, "y"=-0.283603018}, {"x"=-0.185015955, "y"=-0.281067341}, {"x"=-0.182885565, "y"=-0.232877931}, {"x"=-0.18075409, "y"=-0.210029172}, {"x"=-0.178960146, "y"=-0.38453723}, {"x"=-0.176972854, "y"=-0.253307769}, {"x"=-0.17499795, "y"=-0.138967565}, {"x"=-0.173542057, "y"=-0.118840825}, {"x"=-0.171253542, "y"=-0.556553259}, {"x"=-0.169640817, "y"=-2.92005214}, {"x"=-0.167536408, "y"=-5.34303885}, {"x"=-0.165963029, "y"=-3.72848227}, {"x"=-0.163859733, "y"=-1.68214928}, {"x"=-0.162155989, "y"=-0.832957476}, {"x"=-0.16020872, "y"=-0.436744417}, {"x"=-0.158036963, "y"=-0.453113558}, {"x"=-0.15598597, "y"=-0.331085778}, {"x"=-0.155628749, "y"=-0.155152315}, {"x"=-0.153581019, "y"=-0.2117661}, {"x"=-0.151648848, "y"=-0.238660682}, {"x"=-0.149635681, "y"=-0.202118977}, {"x"=-0.147979192, "y"=-0.199871861}, {"x"=-0.145805958, "y"=-0.189630425}, {"x"=-0.144300464, "y"=-0.175867395}, {"x"=-0.142056117, "y"=-0.167481453}, {"x"=-0.140047045, "y"=-0.115747958}, {"x"=-0.138373454, "y"=-0.18791052}, {"x"=-0.136218379, "y"=-0.199324358}, {"x"=-0.134380383, "y"=-0.10791104}, {"x"=-0.132730532, "y"=-0.131513531}, {"x"=-0.130530307, "y"=-0.162132487}, {"x"=-0.128886387, "y"=-0.165394795}, {"x"=-0.126604636, "y"=-0.113909096}, {"x"=-0.124698588, "y"=-0.150031346}, {"x"=-0.122838797, "y"=-0.137792362}, {"x"=-0.121222399, "y"=-0.140428671}, {"x"=-0.118909575, "y"=-0.147887272}, {"x"=-0.117473761, "y"=-0.15345956}, {"x"=-0.115477579, "y"=-0.0537408067}, {"x"=-0.110103078, "y"=-0.51812207}, {"x"=-0.108224772, "y"=-0.383537237}, {"x"=-0.105929355, "y"=-0.378554574}, {"x"=-0.104081993, "y"=-0.349164045}, {"x"=-0.102250618, "y"=-0.351347918}, {"x"=-0.100195133, "y"=-0.302506258}, {"x"=-0.098527987, "y"=-0.314469817}, {"x"=-0.0965328678, "y"=-0.26084746}, {"x"=-0.0942980484, "y"=-0.28866776}, {"x"=-0.0922350638, "y"=-0.240243495}, {"x"=-0.0906668875, "y"=-0.252330628}, {"x"=-0.088716553, "y"=-0.262475152}, {"x"=-0.0863975638, "y"=-0.201562207}, {"x"=-0.0846814559, "y"=-0.261808254}, {"x"=-0.083004609, "y"=-0.218121001}, {"x"=-0.0810332006, "y"=-0.176934212}, {"x"=-0.0788357726, "y"=-0.198935934}, {"x"=-0.0772556174, "y"=-0.237208821}, {"x"=-0.075003195, "y"=-0.183099547}, {"x"=-0.0734207429, "y"=-0.216572388}, {"x"=-0.0712544511, "y"=-0.240701398}, {"x"=-0.069650716, "y"=-0.194500916}, {"x"=-0.0674068702, "y"=-0.174178397}, {"x"=-0.0658028379, "y"=-0.177556083}, {"x"=-0.0638702748, "y"=-0.0925812449}, {"x"=-0.0619029191, "y"=-0.215873948}, {"x"=-0.0597272892, "y"=-0.21184952}, {"x"=-0.0578072933, "y"=-0.190323053}, {"x"=-0.0562117806, "y"=-0.06001647}, {"x"=-0.05445193, "y"=-0.170254777}, {"x"=-0.0525810858, "y"=-0.170367168}, {"x"=-0.0502857008, "y"=-0.168181742}, {"x"=-0.0486110902, "y"=-0.175558466}, {"x"=-0.0464787007, "y"=-0.154948503}, {"x"=-0.0446874833, "y"=-0.168320844}]
  in  "invert 2":bool
  out "LIA2_theta":dbl=180.0
  out "XY Graph X/Y":cluster{"x":dbl, "y":dbl}[](graph)=[{"x"=-0.322787043, "y"=-54.954062263791286}, {"x"=-0.321199055, "y"=-44.382202743822724}, {"x"=-0.319641519, "y"=-42.338230946085666}, {"x"=-0.317848839, "y"=-82.52956220596431}, {"x"=-0.31637601, "y"=-56.41110515283047}, {"x"=-0.314583461, "y"=-40.07471293650691}, {"x"=-0.313190171, "y"=-78.68494292093445}, {"x"=-0.311269881, "y"=-23.226077657558548}, {"x"=-0.310025963, "y"=-19.966963847008827}, {"x"=-0.308131051, "y"=-15.333694852532867}, {"x"=-0.308761592, "y"=-94.33152114454859}, {"x"=-0.307439513, "y"=619.2989448442777}, {"x"=-0.305470965, "y"=-94.97501399277904}, {"x"=-0.304147589, "y"=-30.895223817713603}, {"x"=-0.30246256, "y"=-13.124504883523791}, {"x"=-0.300928863, "y"=-35.02498710517724}, {"x"=-0.298812364, "y"=-30.241674638720056}, {"x"=-0.297199715, "y"=-18.718885951483564}, {"x"=-0.295602105, "y"=-24.368174524293902}, {"x"=-0.293851787, "y"=-21.217731006347954}, {"x"=-0.294151813, "y"=1282.8343046094901}, {"x"=-0.29243944, "y"=-78.2787413355453}, {"x"=-0.290686595, "y"=-181.7803240369281}, {"x"=-0.289023945, "y"=-25.484886562688622}, {"x"=-0.287751596, "y"=125.84934801359096}, {"x"=-0.285984261, "y"=-69.01678049924826}, {"x"=-0.283979079, "y"=-118.31654712042481}, {"x"=-0.282580621, "y"=-46.17344088829248}, {"x"=-0.281093408, "y"=-58.945441204173044}, {"x"=-0.27914764, "y"=-65.72450863198935}, {"x"=-0.277614392, "y"=154.0616598723568}, {"x"=-0.275925137, "y"=-18.678978228503762}, {"x"=-0.274419773, "y"=-41.38183581177788}, {"x"=-0.272372558, "y"=-37.22892393002484}, {"x"=-0.270866655, "y"=30.94619410534774}, {"x"=-0.27152378, "y"=18.332516301379716}, {"x"=-0.269752421, "y"=-49.44857716979914}, {"x"=-0.267939402, "y"=-73.4937484196125}, {"x"=-0.266275686, "y"=-45.80079701486099}, {"x"=-0.264833262, "y"=-41.522759255787754}, {"x"=-0.26326455, "y"=-37.15243143415766}, {"x"=-0.264128599, "y"=-23.279047609885776}, {"x"=-0.262445142, "y"=-10.962735906069408}, {"x"=-0.262336879, "y"=83.1306656961754}, {"x"=-0.26062821, "y"=-20.52303760457062}, {"x"=-0.260051182, "y"=16.814689635294517}, {"x"=-0.258002652, "y"=14.108232802011756}, {"x"=-0.256503799, "y"=65.44076927112037}, {"x"=-0.254967984, "y"=-106.69776804594856}, {"x"=-0.253217838, "y"=-52.93600960496794}, {"x"=-0.25154484, "y"=-84.417510340573}, {"x"=-0.253570898, "y"=5.290484688288777}, {"x"=-0.252252554, "y"=79.33474487979012}, {"x"=-0.250357981, "y"=6.646024897997372}, {"x"=-0.24887687, "y"=13.708371075138297}, {"x"=-0.246973812, "y"=528.9891327449716}, {"x"=-0.245080569, "y"=-41.352261319504954}, {"x"=-0.243618403, "y"=-25.325258331478693}, {"x"=-0.241717931, "y"=-34.38865144450782}, {"x"=-0.240140401, "y"=-75.20229116933318}, {"x"=-0.244515509, "y"=10.744033776238929}, {"x"=-0.242688576, "y"=-41.35787460523785}, {"x"=-0.241456536, "y"=-76.97442412009084}, {"x"=-0.239744527, "y"=126.60376582834924}, {"x"=-0.237643408, "y"=168.98277906185868}, {"x"=-0.235660832, "y"=52.95651902444204}, {"x"=-0.234236103, "y"=55.66734908392923}, {"x"=-0.232251152, "y"=108.5214142796427}, {"x"=-0.230610525, "y"=-31.523398625077085}, {"x"=-0.228509072, "y"=741.8582345223543}, {"x"=-0.22754545, "y"=64.46676419959584}, {"x"=-0.225364111, "y"=23.76895153145993}, {"x"=-0.223780753, "y"=37.30726008592463}, {"x"=-0.221965858, "y"=-62.63597387286001}, {"x"=-0.220091044, "y"=-54.20666218083831}, {"x"=-0.217913064, "y"=-39.22086565720801}, {"x"=-0.220177401, "y"=38.576501745187045}, {"x"=-0.218057431, "y"=-24.34275804665822}, {"x"=-0.216143206, "y"=-40.55945036737629}, {"x"=-0.214330114, "y"=-20.56035834991586}, {"x"=-0.212765963, "y"=-21.82869948965116}, {"x"=-0.210667467, "y"=-11.25956454921926}, {"x"=-0.209045893, "y"=-1.8092621372105033}, {"x"=-0.206809284, "y"=-2.1111917323644205}, {"x"=-0.207721331, "y"=42.73447694526836}, {"x"=-0.205660287, "y"=272.87479119764254}, {"x"=-0.203941355, "y"=38.52567333996761}, {"x"=-0.201753575, "y"=-51.207622198383326}, {"x"=-0.200135187, "y"=69.62170923959259}, {"x"=-0.198155268, "y"=106.72090845577159}, {"x"=-0.195939038, "y"=77.26131943321536}, {"x"=-0.194445954, "y"=85.73298830237643}, {"x"=-0.192305117, "y"=125.46443646917616}, {"x"=-0.190397445, "y"=51.19129597267371}, {"x"=-0.188313238, "y"=114.96198510561544}, {"x"=-0.186454084, "y"=81.24194818424023}, {"x"=-0.184557859, "y"=52.69960552527118}, {"x"=-0.182594798, "y"=82.57886750953743}, {"x"=-0.180976242, "y"=56.03986086899129}, {"x"=-0.179275991, "y"=90.6807369397616}, {"x"=-0.177012006, "y"=65.70535353607593}, {"x"=-0.175604006, "y"=301.78324414439805}, {"x"=-0.173247242, "y"=270.6477237847764}, {"x"=-0.171303705, "y"=680.5525937876657}, {"x"=-0.169543718, "y"=88.17470297928111}, {"x"=-0.167560653, "y"=266.0898048051324}, {"x"=-0.165965036, "y"=-81.88076888899009}, {"x"=-0.164151719, "y"=44.24638036483849}, {"x"=-0.162022405, "y"=245.1785357681447}, {"x"=-0.159981357, "y"=118.67361426916217}, {"x"=-0.158425623, "y"=121.0665783049249}, {"x"=-0.156254606, "y"=78.54242455388818}, {"x"=-0.154643268, "y"=1110.4917461507775}, {"x"=-0.152282509, "y"=662.2292058682173}, {"x"=-0.150781991, "y"=86.48155914030846}, {"x"=-0.148833689, "y"=47.72765600833068}, {"x"=-0.146586605, "y"=55.20468008805976}, {"x"=-0.14560995, "y"=45.427787471974376}, {"x"=-0.143964455, "y"=36.84356312110366}, {"x"=-0.141626495, "y"=31.661824694743363}, {"x"=-0.139881026, "y"=48.41626221510616}, {"x"=-0.137779717, "y"=57.10495060725086}, {"x"=-0.136030143, "y"=52.75201540919181}, {"x"=-0.13419042, "y"=55.5143311694662}, {"x"=-0.132711144, "y"=54.61027958843574}, {"x"=-0.130451074, "y"=81.37557911834018}, {"x"=-0.128810501, "y"=77.0113733737781}, {"x"=-0.126958394, "y"=55.9380391637756}, {"x"=-0.12473916, "y"=89.72649071069219}, {"x"=-0.123088683, "y"=73.27273097360022}, {"x"=-0.121186876, "y"=64.57757769614778}, {"x"=-0.118801661, "y"=96.59140339581516}, {"x"=-0.117223427, "y"=41.81174815054659}, {"x"=-0.115411257, "y"=68.60167125264736}, {"x"=-0.113408483, "y"=69.93793908533165}, {"x"=-0.108301375, "y"=20.009353226822693}, {"x"=-0.106018714, "y"=21.967617635245094}, {"x"=-0.104142091, "y"=27.10652630077251}, {"x"=-0.102086436, "y"=29.521880304545792}, {"x"=-0.100572828, "y"=28.44640783335457}, {"x"=-0.0983704144, "y"=29.99749821094508}, {"x"=-0.0965622226, "y"=33.30519343719728}, {"x"=-0.0946816698, "y"=39.547178601088646}, {"x"=-0.0925342996, "y"=35.59577755688429}, {"x"=-0.090322695, "y"=38.586417509129504}, {"x"=-0.088411526, "y"=54.313304493027324}, {"x"=-0.0865955332, "y"=61.78134518421936}, {"x"=-0.0845164829, "y"=43.726508400392774}, {"x"=-0.0829999518, "y"=38.319537964012675}, {"x"=-0.0808891903, "y"=37.14747315972461}, {"x"=-0.0791214438, "y"=49.63213009745526}, {"x"=-0.0768329643, "y"=46.566444310864846}, {"x"=-0.0750250485, "y"=55.16373291243214}, {"x"=-0.0733882392, "y"=54.71534539747113}, {"x"=-0.0714707316, "y"=60.89642647672887}, {"x"=-0.0696832844, "y"=43.177456310256346}, {"x"=-0.0675760949, "y"=48.56396505250542}, {"x"=-0.0654008533, "y"=52.32464995837036}, {"x"=-0.0637381165, "y"=67.38842287949616}, {"x"=-0.0620785275, "y"=52.57953036011127}, {"x"=-0.0598791047, "y"=64.79899870766555}, {"x"=-0.0582539961, "y"=45.395077238185166}, {"x"=-0.0560150441, "y"=46.0442708780103}, {"x"=-0.054387143, "y"=53.4853682386828}, {"x"=-0.0526325672, "y"=55.087282955547394}, {"x"=-0.0504881694, "y"=55.64850517014705}, {"x"=-0.0483964309, "y"=62.40730674164013}, {"x"=-0.0466539884, "y"=59.9038235670925}, {"x"=-0.045046612, "y"=52.73845345216831}, {"x"=-0.33546486, "y"=192.24582409997203}, {"x"=-0.333745786, "y"=-54.96599193227588}, {"x"=-0.332027408, "y"=-41.0201976954244}, {"x"=-0.33031564, "y"=-138.26581006025427}, {"x"=-0.328486109, "y"=-699.4609311863442}, {"x"=-0.326560143, "y"=-56.97406570728075}, {"x"=-0.32512298, "y"=-73.52627063179571}, {"x"=-0.323181196, "y"=-62.13788203055595}, {"x"=-0.321392607, "y"=-123.22793555983822}, {"x"=-0.319879104, "y"=-136.07015083898946}, {"x"=-0.31796566, "y"=-62.94114125893015}, {"x"=-0.316529991, "y"=-126.75770419994832}, {"x"=-0.314809426, "y"=-98.32773773561513}, {"x"=-0.312919112, "y"=180.515768459127}, {"x"=-0.311386684, "y"=596.5088776898192}, {"x"=-0.310231483, "y"=-38.41984459915608}, {"x"=-0.30840411, "y"=-27.71611843173893}, {"x"=-0.306923182, "y"=-23.36966631358744}, {"x"=-0.305284299, "y"=-26.938852210939984}, {"x"=-0.303978001, "y"=424.50157026616967}, {"x"=-0.302407437, "y"=-31.868649826757842}, {"x"=-0.300353654, "y"=-52.835022665326655}, {"x"=-0.299009745, "y"=-51.07797252505597}, {"x"=-0.297135444, "y"=-66.66580167378167}, {"x"=-0.295633444, "y"=-60.11245447654392}, {"x"=-0.29351129, "y"=-49.125061358788834}, {"x"=-0.29195779, "y"=-47.92058618772724}, {"x"=-0.290072575, "y"=-42.56746547273237}, {"x"=-0.288616403, "y"=-29.715147356335834}, {"x"=-0.28685982, "y"=-23.645701443523652}, {"x"=-0.284981802, "y"=-24.061655711921723}, {"x"=-0.286155601, "y"=-71.30942046163656}, {"x"=-0.28456383, "y"=-42.31514690105571}, {"x"=-0.282983103, "y"=-33.55122201531537}, {"x"=-0.281048017, "y"=-48.07149133606031}, {"x"=-0.279525482, "y"=-31.249128659340137}, {"x"=-0.277522001, "y"=-28.24192045540498}, {"x"=-0.275692755, "y"=-22.522113405170884}, {"x"=-0.277391098, "y"=-28.02722964741073}, {"x"=-0.276047316, "y"=-25.731022917697015}, {"x"=-0.27421589, "y"=-12.253216171887546}, {"x"=-0.272343889, "y"=-17.620550045887075}, {"x"=-0.274813497, "y"=2.738634286537641}, {"x"=-0.272726147, "y"=2.4164599438750107}, {"x"=-0.271212771, "y"=6.248253715849401}, {"x"=-0.272350618, "y"=2.84387870101219}, {"x"=-0.287880604, "y"=26.336155764141125}, {"x"=-0.286170652, "y"=-47.682519147523124}, {"x"=-0.284573849, "y"=-692.8418465947557}, {"x"=-0.282597084, "y"=-38.586015881584366}, {"x"=-0.280618361, "y"=22.54207174802097}, {"x"=-0.278619809, "y"=556.8770211048375}, {"x"=-0.27633614, "y"=37.3873627612659}, {"x"=-0.274407004, "y"=-3.8729432399128862}, {"x"=-0.272763788, "y"=-7.795232922454721}, {"x"=-0.270651555, "y"=-7.79237670651501}, {"x"=-0.269080381, "y"=-12.159668262214675}, {"x"=-0.267149812, "y"=-15.557198480981407}, {"x"=-0.264833714, "y"=-30.018379765797242}, {"x"=-0.263101554, "y"=-57.53663217272394}, {"x"=-0.261011053, "y"=-48.29199497822009}, {"x"=-0.259431161, "y"=-19.091976961624862}, {"x"=-0.257198556, "y"=-1.5281114828071407}, {"x"=-0.255303332, "y"=-0.8671772490019715}, {"x"=-0.253603289, "y"=-1.4620545032646717}, {"x"=-0.25143457, "y"=1.8893550360360751}, {"x"=-0.249252673, "y"=1.0680829780344825}, {"x"=-0.247462245, "y"=2.8356830554904295}, {"x"=-0.245835108, "y"=13.08447051612279}, {"x"=-0.243873961, "y"=-169.51546255793343}, {"x"=-0.241739098, "y"=30.393531353775344}, {"x"=-0.240041187, "y"=167.08148153282843}, {"x"=-0.238007002, "y"=-79.44423325911522}, {"x"=-0.235249673, "y"=5.544999241613793}, {"x"=-0.227840785, "y"=86.60075716689221}, {"x"=-0.225940127, "y"=-452.39583072937245}, {"x"=-0.223825652, "y"=108.03691624260614}, {"x"=-0.221970814, "y"=67.03612996437109}, {"x"=-0.220014541, "y"=110.69916058810655}, {"x"=-0.217799738, "y"=157.08938445519172}, {"x"=-0.215881379, "y"=40.52771096143696}, {"x"=-0.213892054, "y"=463.1029753718033}, {"x"=-0.2121817, "y"=69.46817819146207}, {"x"=-0.210212025, "y"=-373.727663945333}, {"x"=-0.207986748, "y"=38.81506762272053}, {"x"=-0.206042782, "y"=28.470540741037425}, {"x"=-0.203913947, "y"=52.375646847692856}, {"x"=-0.202084169, "y"=-77.45440332532891}, {"x"=-0.200067279, "y"=104.6477010136639}, {"x"=-0.198512359, "y"=2729.8777168284096}, {"x"=-0.196275716, "y"=179.5902327978076}, {"x"=-0.194173193, "y"=153.58147615330157}, {"x"=-0.192465034, "y"=76.43581355504264}, {"x"=-0.190561227, "y"=75.15644308908968}, {"x"=-0.18842698, "y"=67.23564222837244}, {"x"=-0.186699678, "y"=33.85035007507106}, {"x"=-0.184462355, "y"=36.096467851638494}, {"x"=-0.182505268, "y"=306.990419875238}, {"x"=-0.180845258, "y"=16.982430056112925}, {"x"=-0.179114495, "y"=24.280746119096236}, {"x"=-0.176981756, "y"=68.59492258075707}, {"x"=-0.174716301, "y"=37.474362382159754}, {"x"=-0.173089533, "y"=82.76520809178132}, {"x"=-0.170918962, "y"=17.167444657643383}, {"x"=-0.169286517, "y"=115.31114853062137}, {"x"=-0.167154998, "y"=31.534411795468642}, {"x"=-0.165491932, "y"=18.715847137849515}, {"x"=-0.163230759, "y"=-20.29646619972446}, {"x"=-0.161303356, "y"=-34.11273325765365}, {"x"=-0.159692251, "y"=-74.58140399942359}, {"x"=-0.15733545, "y"=29.767254804144045}, {"x"=-0.15541656, "y"=-454.0356366264771}, {"x"=-0.153584974, "y"=-561.3279813376836}, {"x"=-0.151892049, "y"=-116.29127474774658}, {"x"=-0.149952556, "y"=-23.330621058698462}, {"x"=-0.147572331, "y"=188.1666351348057}, {"x"=-0.145838915, "y"=-20.727702254195822}, {"x"=-0.143868593, "y"=48.68735044229641}, {"x"=-0.141802589, "y"=-25.612315598598414}, {"x"=-0.139841049, "y"=-91.12080589455445}, {"x"=-0.138219334, "y"=102.93115924394965}, {"x"=-0.136394404, "y"=69.09293817440374}, {"x"=-0.13405063, "y"=-61.552972494949486}, {"x"=-0.132167455, "y"=41.57656740775237}, {"x"=-0.130170797, "y"=201.41419987898894}, {"x"=-0.128312485, "y"=-119.49009502702616}, {"x"=-0.126696194, "y"=-101.00646717992929}, {"x"=-0.124831877, "y"=5752.5242047844085}, {"x"=-0.122771378, "y"=100.39840935206801}, {"x"=-0.120647398, "y"=513.6954596505265}, {"x"=-0.118563562, "y"=200.86306363618817}, {"x"=-0.116871469, "y"=-261.9240849026062}, {"x"=-0.11469853, "y"=40.566052053572065}, {"x"=-0.113263185, "y"=105.5398662080192}, {"x"=-0.111279785, "y"=124.02060424332954}, {"x"=-0.109080486, "y"=78.89475773632094}, {"x"=-0.107491191, "y"=47.647395491886044}, {"x"=-0.105162271, "y"=98.41287300390553}, {"x"=-0.10312842, "y"=91.48808096758368}, {"x"=-0.101222318, "y"=54.52160358528141}, {"x"=-0.0997517275, "y"=62.22133844228142}, {"x"=-0.0977370158, "y"=172.54069936865835}, {"x"=-0.0954946324, "y"=66.03714496286209}, {"x"=-0.093983814, "y"=65.76927876156292}, {"x"=-0.0917944442, "y"=71.12574376708972}, {"x"=-0.0896674925, "y"=75.10896958434388}, {"x"=-0.0877880269, "y"=102.03468909471547}, {"x"=-0.0861468046, "y"=95.93028493205813}, {"x"=-0.0838770832, "y"=67.35577493802852}, {"x"=-0.0821798867, "y"=67.99481206327647}, {"x"=-0.0800045894, "y"=245.83439863704533}, {"x"=-0.0784491118, "y"=76.00263175205639}, {"x"=-0.0761974652, "y"=93.37329096585214}, {"x"=-0.0742721754, "y"=86.87771099319131}, {"x"=-0.0725907591, "y"=105.73670787781829}, {"x"=-0.0704837339, "y"=81.89384916766575}, {"x"=-0.0684716502, "y"=80.51956352731239}, {"x"=-0.0667799036, "y"=58.43527727474232}, {"x"=-0.0645956838, "y"=94.13592845205737}, {"x"=-0.0628243791, "y"=98.23268906636554}, {"x"=-0.061197419, "y"=94.77994897263673}, {"x"=-0.0592657311, "y"=80.98940659840474}, {"x"=-0.0572713287, "y"=76.56873234697629}, {"x"=-0.0550249622, "y"=76.52127162151098}, {"x"=-0.0533176284, "y"=88.0682413374226}, {"x"=-0.0511257474, "y"=68.16895417137137}, {"x"=-0.0496148763, "y"=77.52533760016064}, {"x"=-0.0474064899, "y"=100.97172070739667}, {"x"=-0.0458457776, "y"=99.08314031433615}, {"x"=-0.0436728396, "y"=76.60401217898679}, {"x"=-0.335300985, "y"=-160.8038088219164}, {"x"=-0.333358443, "y"=-45.1335667714711}, {"x"=-0.331994923, "y"=-58.07843227726001}, {"x"=-0.329879283, "y"=-195.9223251349081}, {"x"=-0.328221987, "y"=-62.32787793185222}, {"x"=-0.326820179, "y"=-165.77125323697084}, {"x"=-0.325145707, "y"=-75.11208896329323}, {"x"=-0.323297249, "y"=74.01977569660731}, {"x"=-0.321341372, "y"=22.863735703224936}, {"x"=-0.320043967, "y"=6.662035333699096}, {"x"=-0.318258686, "y"=4.827656843351891}, {"x"=-0.316277219, "y"=6.604145481891222}, {"x"=-0.314496083, "y"=-16.090660207652647}, {"x"=-0.312915343, "y"=-4.575130065868565}, {"x"=-0.3114785, "y"=-4.377745947053211}, {"x"=-0.309584272, "y"=-6.483108475742563}, {"x"=-0.307655174, "y"=-11.358639604194375}, {"x"=-0.306259845, "y"=-9.377456729991852}, {"x"=-0.305776428, "y"=16.059838900197235}, {"x"=-0.304183555, "y"=203.8875694792229}, {"x"=-0.302462318, "y"=-38.02679825913215}, {"x"=-0.300622776, "y"=-36.18049688721548}, {"x"=-0.299315977, "y"=-38.61965069146352}, {"x"=-0.297270442, "y"=-36.53623997467315}, {"x"=-0.295672569, "y"=-35.70864883753923}, {"x"=-0.294238957, "y"=-28.725901147709582}, {"x"=-0.292131459, "y"=-22.88054304078593}, {"x"=-0.290527277, "y"=-25.155711198301073}, {"x"=-0.291216476, "y"=-54.616932071006985}, {"x"=-0.289302491, "y"=-35.98032497647735}, {"x"=-0.287725507, "y"=-50.42153942028024}, {"x"=-0.285879009, "y"=-68.1631524871292}, {"x"=-0.284403058, "y"=-42.831397703682185}, {"x"=-0.282416097, "y"=-42.14465974388012}, {"x"=-0.28068587, "y"=-71.08395049234112}, {"x"=-0.282424738, "y"=2.006227336859227}, {"x"=-0.280266782, "y"=-51.00031565246628}, {"x"=-0.278483947, "y"=-490.9442431116294}, {"x"=-0.277039123, "y"=-60.48651985427588}, {"x"=-0.27504806, "y"=-27.80573991260645}, {"x"=-0.273495057, "y"=-19.148527354267966}, {"x"=-0.274880326, "y"=10.403076937523322}, {"x"=-0.273413063, "y"=-15.047998357408279}, {"x"=-0.271467164, "y"=-2.2583037666962498}, {"x"=-0.269896948, "y"=-2.4409818628391227}, {"x"=-0.271869291, "y"=-17.196592121958915}, {"x"=-0.270139462, "y"=-12.793219045418718}, {"x"=-0.268232076, "y"=-8.960693969946325}, {"x"=-0.266588994, "y"=-6.050557020472703}, {"x"=-0.264785425, "y"=-5.835838584154999}, {"x"=-0.27683418, "y"=27.200933066173796}, {"x"=-0.274849151, "y"=39.435239814102324}, {"x"=-0.272729394, "y"=-3.5821106191968823}, {"x"=-0.270232483, "y"=-2.018616295944517}, {"x"=-0.268513891, "y"=-2.4716304003110627}, {"x"=-0.265417755, "y"=22.715343620148754}, {"x"=-0.263370988, "y"=-33.77282980269312}, {"x"=-0.261654961, "y"=-9.503967602014454}, {"x"=-0.259956656, "y"=-6.597709649641318}, {"x"=-0.257690691, "y"=9.8643103872448}, {"x"=-0.255804833, "y"=23.266703080649318}, {"x"=-0.253856049, "y"=7.258216089924982}, {"x"=-0.251715583, "y"=5.3383266198166375}, {"x"=-0.249536187, "y"=-696.2148288834427}, {"x"=-0.248038815, "y"=32.09318698073028}, {"x"=-0.245953065, "y"=11.006412138082647}, {"x"=-0.243651513, "y"=20.25155489381619}, {"x"=-0.241777916, "y"=11.469655268364335}, {"x"=-0.2397567, "y"=9.767987679393606}, {"x"=-0.237955861, "y"=34.827843024387114}, {"x"=-0.236195076, "y"=16.288509798066197}, {"x"=-0.234019395, "y"=17.14436474865723}, {"x"=-0.232135587, "y"=-13.851690058402328}, {"x"=-0.230261758, "y"=-13.757938743765502}, {"x"=-0.227995713, "y"=16.889609745269055}, {"x"=-0.22640226, "y"=-46.147732238787185}, {"x"=-0.224489787, "y"=14.732155619386027}, {"x"=-0.222937216, "y"=13.169530505713686}, {"x"=-0.220707299, "y"=48.54534149198434}, {"x"=-0.21902656, "y"=599.762005102874}, {"x"=-0.216914885, "y"=74.48693497456928}, {"x"=-0.215144185, "y"=13.127712144878949}, {"x"=-0.213000597, "y"=-11.293947431122028}, {"x"=-0.210835011, "y"=704.6891302116978}, {"x"=-0.208732451, "y"=52.7177922338507}, {"x"=-0.206836672, "y"=158.46669292493416}, {"x"=-0.204888076, "y"=132.30477142562452}, {"x"=-0.202883788, "y"=-1492.0124957227617}, {"x"=-0.20117002, "y"=-78.77639165693378}, {"x"=-0.199454378, "y"=-332.8090384293103}, {"x"=-0.197207422, "y"=-69.46747123292634}, {"x"=-0.195086354, "y"=-33.04372263052362}, {"x"=-0.19314994, "y"=-21.002479250417974}, {"x"=-0.191593151, "y"=-11.547957314672013}, {"x"=-0.189528581, "y"=-264.4694522925105}, {"x"=-0.187456389, "y"=4.294228098091214}, {"x"=-0.185256834, "y"=4.044495391096901}, {"x"=-0.183457199, "y"=2.7469909517215676}, {"x"=-0.181519272, "y"=3.554037958655317}, {"x"=-0.179406659, "y"=12.477945469509988}, {"x"=-0.177541575, "y"=40.960582703798366}, {"x"=-0.175778757, "y"=37.59448556962528}, {"x"=-0.173726813, "y"=-5.099819310057324}, {"x"=-0.171597052, "y"=-2.2365464556590173}, {"x"=-0.169672896, "y"=-1.4504244879269654}, {"x"=-0.168003407, "y"=-1.1333453104289672}, {"x"=-0.166273217, "y"=-2.216364476385738}, {"x"=-0.163954349, "y"=-2.8491081209748326}, {"x"=-0.162151276, "y"=-1.2836195172834841}, {"x"=-0.160035162, "y"=-5.383042160598753}, {"x"=-0.158433476, "y"=6.3781180295382995}, {"x"=-0.156545796, "y"=-10.978080784529709}, {"x"=-0.154240853, "y"=4.326285980531332}, {"x"=-0.152571786, "y"=4.99637284572679}, {"x"=-0.150578709, "y"=78.01102114157896}, {"x"=-0.14877761, "y"=-22.04395980293144}, {"x"=-0.146343706, "y"=-9.536383441379888}, {"x"=-0.144622141, "y"=-22.040675992758217}, {"x"=-0.14242199, "y"=-8.024128639141123}, {"x"=-0.140620239, "y"=-13.56549097595987}, {"x"=-0.13852428, "y"=-4.874242414909319}, {"x"=-0.137051714, "y"=-10.077994090034533}, {"x"=-0.134867378, "y"=-8.16664151727311}, {"x"=-0.132636495, "y"=3.502473535333689}, {"x"=-0.131045293, "y"=46.88972738272575}, {"x"=-0.12899907, "y"=2.9623238096845563}, {"x"=-0.126784688, "y"=3.508112408519507}, {"x"=-0.125174281, "y"=3.98127759222838}, {"x"=-0.122927589, "y"=5.464761322581351}, {"x"=-0.12089258, "y"=7.4372121972431895}, {"x"=-0.119164564, "y"=10.734365258173556}, {"x"=-0.117458919, "y"=19.684595407547206}, {"x"=-0.11536099, "y"=14.410438305833166}, {"x"=-0.113352547, "y"=53.62157269067614}, {"x"=-0.111574727, "y"=36.04429778827072}, {"x"=-0.109547957, "y"=44.04694515993814}, {"x"=-0.107303376, "y"=60.088545387653355}, {"x"=-0.105703842, "y"=43.80365296467063}, {"x"=-0.103545383, "y"=80.7414556582182}, {"x"=-0.101585481, "y"=48.3057533942954}, {"x"=-0.0995221016, "y"=54.32783918981812}, {"x"=-0.0974260343, "y"=53.89637606935303}, {"x"=-0.0955153682, "y"=46.45027869032277}, {"x"=-0.093576077, "y"=43.21537687288188}, {"x"=-0.0915771446, "y"=42.81825466208823}, {"x"=-0.0898800944, "y"=56.46831012018703}, {"x"=-0.0876324226, "y"=35.4104972300929}, {"x"=-0.0858551057, "y"=42.57653600404335}, {"x"=-0.0837586556, "y"=59.02579334589803}, {"x"=-0.0817462905, "y"=46.68551936107214}, {"x"=-0.0800427965, "y"=59.0913402134093}, {"x"=-0.0783492425, "y"=45.25092108742939}, {"x"=-0.0763397978, "y"=38.67625592661037}, {"x"=-0.074115245, "y"=86.17269037112229}, {"x"=-0.0719559478, "y"=45.98615827209259}, {"x"=-0.0702906117, "y"=37.97436437084765}, {"x"=-0.0680818369, "y"=62.723466739163776}, {"x"=-0.066455871, "y"=38.12258199790152}, {"x"=-0.0642113441, "y"=29.99813173595266}, {"x"=-0.0622005869, "y"=41.5090394913788}, {"x"=-0.0604427976, "y"=46.22506040652222}, {"x"=-0.0587854654, "y"=53.05099520991607}, {"x"=-0.0566201468, "y"=46.812537355421796}, {"x"=-0.0547194201, "y"=55.661205004776335}, {"x"=-0.0528823607, "y"=54.153134538824176}, {"x"=-0.0507147264, "y"=50.60697241529042}, {"x"=-0.0484772375, "y"=69.2303595813946}, {"x"=-0.0466248086, "y"=67.43479838752678}, {"x"=-0.0449897343, "y"=53.79773961834569}, {"x"=-0.0430836992, "y"=73.46586787160733}, {"x"=-0.33682919, "y"=23.138655830309666}, {"x"=-0.335313862, "y"=13.438401039532495}, {"x"=-0.333552779, "y"=14.179734224122827}, {"x"=-0.33207168, "y"=33.396886265013464}, {"x"=-0.329993812, "y"=-161.4631384349433}, {"x"=-0.328495231, "y"=343.54930851472056}, {"x"=-0.326605364, "y"=-61.63634808073303}, {"x"=-0.325195679, "y"=-78.76751799014822}, {"x"=-0.323214139, "y"=-43.487574936215495}, {"x"=-0.321402015, "y"=-47.331254156180535}, {"x"=-0.31979714, "y"=-60.30525497837613}, {"x"=-0.318284733, "y"=-50.7417214640801}, {"x"=-0.316682905, "y"=-75.68273546293615}, {"x"=-0.31470433, "y"=-61.430073716348325}, {"x"=-0.31293092, "y"=-71.16211599544366}, {"x"=-0.311211422, "y"=-125.44411209770509}, {"x"=-0.309797672, "y"=-75.90733523027511}, {"x"=-0.307884355, "y"=-34.55663353075861}, {"x"=-0.306366118, "y"=-35.400432367595755}, {"x"=-0.304629401, "y"=-57.296890794025174}, {"x"=-0.302746113, "y"=-79.73957109614717}, {"x"=-0.301229582, "y"=-32.88577620549041}, {"x"=-0.299409617, "y"=-43.087525393362036}, {"x"=-0.297772288, "y"=-35.27364713484051}, {"x"=-0.296075782, "y"=-31.319841464696644}, {"x"=-0.295629285, "y"=-64.33646088763226}, {"x"=-0.293901675, "y"=-54.85602338486247}, {"x"=-0.292224269, "y"=-35.51132144193735}, {"x"=-0.290168079, "y"=-30.036813908841122}, {"x"=-0.288631256, "y"=-26.93277917656821}, {"x"=-0.287109328, "y"=-25.348799297989483}, {"x"=-0.285270679, "y"=-25.06232832750102}, {"x"=-0.283521525, "y"=-22.95638390839481}, {"x"=-0.281608898, "y"=-21.02418256815754}, {"x"=-0.280040753, "y"=-20.082800095750535}, {"x"=-0.281208104, "y"=22.337244093273448}, {"x"=-0.279477566, "y"=-81.12420551887385}, {"x"=-0.277562802, "y"=-53.43131334598029}, {"x"=-0.275810682, "y"=-70.41007799701278}, {"x"=-0.274340632, "y"=-33.6029560756409}, {"x"=-0.272315401, "y"=-38.34980075391038}, {"x"=-0.270811509, "y"=-34.321384183810686}, {"x"=-0.268855133, "y"=-19.240427896660197}, {"x"=-0.267570983, "y"=-3.536477864993775}, {"x"=-0.269258717, "y"=2.3395603368437374}, {"x"=-0.267393552, "y"=-4.669232129140092}, {"x"=-0.265561271, "y"=-6.48751637899932}, {"x"=-0.264067518, "y"=13.03504099600386}, {"x"=-0.26622104, "y"=2.3655678640335336}, {"x"=-0.264309492, "y"=2.14685057130977}, {"x"=-0.261641646, "y"=-23.909619524889766}, {"x"=-0.259693672, "y"=-30.992263361320784}, {"x"=-0.257814117, "y"=-24.25629531870238}, {"x"=-0.264146579, "y"=-95.90429911346197}, {"x"=-0.262532862, "y"=17.221786921260488}, {"x"=-0.260533953, "y"=25.856032146416748}, {"x"=-0.259042779, "y"=86.12402730615784}, {"x"=-0.256603823, "y"=-1.4085259216029777}, {"x"=-0.25530149, "y"=5.409881302326991}, {"x"=-0.253134282, "y"=-18.123488507184934}, {"x"=-0.253997112, "y"=45.54966334026043}, {"x"=-0.251880021, "y"=-58.45669243789711}, {"x"=-0.25012447, "y"=13.867429182914956}, {"x"=-0.248140176, "y"=48.73579162867171}, {"x"=-0.246211539, "y"=35.56758958347463}, {"x"=-0.244594126, "y"=817.3204625915234}, {"x"=-0.242670121, "y"=19.57324809169297}, {"x"=-0.240974151, "y"=55.31185927664324}, {"x"=-0.238953421, "y"=-168.43780831472986}, {"x"=-0.237098164, "y"=49.335497763544744}, {"x"=-0.235521425, "y"=39.93133253645086}, {"x"=-0.233516246, "y"=49.20867833026398}, {"x"=-0.231844197, "y"=88.48120157083711}, {"x"=-0.229783176, "y"=8.202539892588314}, {"x"=-0.227802205, "y"=10.937911207499342}, {"x"=-0.226111479, "y"=12.943299040658127}, {"x"=-0.224482412, "y"=16.553506921651888}, {"x"=-0.22395215, "y"=-14.678759705411418}, {"x"=-0.222945264, "y"=17.779527334100443}, {"x"=-0.221215758, "y"=17.3494709252612}, {"x"=-0.219232801, "y"=20.0738092497242}, {"x"=-0.217016729, "y"=38.16361636678784}, {"x"=-0.215488248, "y"=31.519138716255856}, {"x"=-0.213342378, "y"=28.08644462991057}, {"x"=-0.21162352, "y"=18.420584923752365}, {"x"=-0.209677239, "y"=28.72775546780428}, {"x"=-0.207802203, "y"=161.97179181245522}, {"x"=-0.205293229, "y"=33.389651664252334}, {"x"=-0.203199825, "y"=12.672963256800275}, {"x"=-0.20137161, "y"=18.883451677518153}, {"x"=-0.199508508, "y"=190.76840963157622}, {"x"=-0.19737781, "y"=33.02612948705384}, {"x"=-0.195573129, "y"=53.88673918315542}, {"x"=-0.193470874, "y"=25.008108548568547}, {"x"=-0.191832838, "y"=34.1860368171851}, {"x"=-0.191138425, "y"=2.3497809358423525}, {"x"=-0.189658678, "y"=4.272421921767929}, {"x"=-0.187703383, "y"=4.959597464430206}, {"x"=-0.185629928, "y"=8.72005638706392}, {"x"=-0.18382079, "y"=1.7966878957941264}, {"x"=-0.181788557, "y"=36.126052618142545}, {"x"=-0.179782592, "y"=44.666893279491305}, {"x"=-0.177990286, "y"=41.94605702518529}, {"x"=-0.175618776, "y"=44.70683278325653}, {"x"=-0.173936671, "y"=34.600004268202056}, {"x"=-0.172236219, "y"=46.821389283839444}, {"x"=-0.170233589, "y"=42.000800441601505}, {"x"=-0.168294763, "y"=45.035976334698006}, {"x"=-0.16643041, "y"=51.60964258594908}, {"x"=-0.164228563, "y"=56.51014536441861}, {"x"=-0.162114313, "y"=71.68789874407435}, {"x"=-0.160459775, "y"=48.39331963175463}, {"x"=-0.158291148, "y"=64.34497908674741}, {"x"=-0.156680405, "y"=34.83853068746807}, {"x"=-0.154827172, "y"=64.5689341197733}, {"x"=-0.152471832, "y"=47.023360403986096}, {"x"=-0.150809383, "y"=34.393010631680426}, {"x"=-0.148634945, "y"=42.83460486634582}, {"x"=-0.146749619, "y"=41.36769085325276}, {"x"=-0.145157296, "y"=41.88625009825457}, {"x"=-0.14280677, "y"=65.89591107653077}, {"x"=-0.137006255, "y"=22.761086657326587}, {"x"=-0.135267993, "y"=21.070501759527474}, {"x"=-0.133167177, "y"=24.400099856404402}, {"x"=-0.130865236, "y"=25.066722097607467}, {"x"=-0.129285093, "y"=31.89868656511745}, {"x"=-0.127078096, "y"=27.36830359338832}, {"x"=-0.125344703, "y"=31.572023613454608}, {"x"=-0.122925281, "y"=29.980484589940964}, {"x"=-0.121176743, "y"=40.68297911339099}, {"x"=-0.118619154, "y"=16.041035438240364}, {"x"=-0.117151046, "y"=21.751889694245936}, {"x"=-0.114917536, "y"=45.04027779147186}, {"x"=-0.112881645, "y"=55.4572878641065}, {"x"=-0.110946263, "y"=86.1636968453139}, {"x"=-0.109267506, "y"=-223.0756934235952}, {"x"=-0.107469592, "y"=24.796218416064693}, {"x"=-0.105157961, "y"=25.120830135206496}, {"x"=-0.103528003, "y"=41.21023711451793}, {"x"=-0.101574394, "y"=28.500609685175405}, {"x"=-0.0994831378, "y"=-1891.1589613094206}, {"x"=-0.0978756645, "y"=50.45196164744634}, {"x"=-0.0956713202, "y"=149.24389329656836}, {"x"=-0.0937902776, "y"=24.446210857188117}, {"x"=-0.092082075, "y"=56.78277562314769}, {"x"=-0.0901464766, "y"=45.215476066362285}, {"x"=-0.0879565344, "y"=22.97318224196671}, {"x"=-0.0859257596, "y"=148.09939045762655}, {"x"=-0.0840165846, "y"=15.750398090411515}, {"x"=-0.0822342902, "y"=17.766528780848542}, {"x"=-0.080622133, "y"=93.55176555328846}, {"x"=-0.0783561114, "y"=22.756006498980003}, {"x"=-0.0764459296, "y"=-30.80463698769502}, {"x"=-0.0744766918, "y"=-58.649274211164844}, {"x"=-0.0727752286, "y"=11.26123412470191}, {"x"=-0.0706377629, "y"=18.2231850581126}, {"x"=-0.0687834019, "y"=91.33217253417412}, {"x"=-0.067267852, "y"=-22.62243490299643}, {"x"=-0.0649109219, "y"=50.48462532428942}, {"x"=-0.0633371951, "y"=-52.01621750483901}, {"x"=-0.0614975702, "y"=51.8713659767444}, {"x"=-0.0596667688, "y"=-54.799223672730264}, {"x"=-0.0575341856, "y"=42.60498014252613}, {"x"=-0.0558201398, "y"=79.08838390821002}, {"x"=-0.0534663067, "y"=16.960461405367855}, {"x"=-0.0518633207, "y"=-23.160351326569202}, {"x"=-0.0500697023, "y"=65.67043715148087}, {"x"=-0.0478193066, "y"=38.30797331035716}, {"x"=-0.0462411904, "y"=33.75687125832537}, {"x"=-0.0444286992, "y"=108.30859759281182}, {"x"=-0.338726307, "y"=-11.566816115507722}, {"x"=-0.336933848, "y"=-12.483153856913328}, {"x"=-0.335312612, "y"=-33.22802679342729}, {"x"=-0.333588895, "y"=15.012517474794706}, {"x"=-0.331523407, "y"=9.581810895565193}, {"x"=-0.32981741, "y"=12.532066411538485}, {"x"=-0.328028071, "y"=51.90396117719565}, {"x"=-0.326401821, "y"=-168.18043058221897}, {"x"=-0.324984329, "y"=100.06887079053085}, {"x"=-0.323264419, "y"=-339.52954136541666}, {"x"=-0.321215795, "y"=-109.07257351964812}, {"x"=-0.319429341, "y"=-137.65796793390825}, {"x"=-0.317705652, "y"=-74.42663512066055}, {"x"=-0.316252294, "y"=-99.7757185559154}, {"x"=-0.314273418, "y"=-74.61899175942041}, {"x"=-0.312616976, "y"=-59.149541906963535}, {"x"=-0.311250279, "y"=-126.40516262597461}, {"x"=-0.309309309, "y"=-190.30519129654098}, {"x"=-0.307867444, "y"=-80.83438788688834}, {"x"=-0.306006106, "y"=-86.55468100198226}, {"x"=-0.304098247, "y"=-88.21289950197288}, {"x"=-0.302632408, "y"=-73.35977241488244}, {"x"=-0.300806821, "y"=-94.0182524006761}, {"x"=-0.298836948, "y"=-46.68164075928833}, {"x"=-0.297571904, "y"=-33.72373236617088}, {"x"=-0.295886637, "y"=-44.61906791234327}, {"x"=-0.294614436, "y"=-74.3953828601536}, {"x"=-0.293054135, "y"=-40.050879462786895}, {"x"=-0.291070233, "y"=-53.98983532694451}, {"x"=-0.289213666, "y"=-45.67082558280026}, {"x"=-0.287506173, "y"=-50.95196327598177}, {"x"=-0.286004532, "y"=-35.60298073992563}, {"x"=-0.284008765, "y"=-48.17646480267314}, {"x"=-0.282480195, "y"=-67.03689266095606}, {"x"=-0.281034734, "y"=-36.18272043953299}, {"x"=-0.278962449, "y"=-35.45618183945229}, {"x"=-0.277211169, "y"=-33.861872724965}, {"x"=-0.275869818, "y"=-23.91058923527929}, {"x"=-0.275858707, "y"=-45.969060343198755}, {"x"=-0.274265871, "y"=-198.33516876777563}, {"x"=-0.272790832, "y"=-46.51984469963305}, {"x"=-0.271063181, "y"=-68.29476141356099}, {"x"=-0.2691099, "y"=-47.852791733032674}, {"x"=-0.267199649, "y"=-40.16364901160454}, {"x"=-0.265874043, "y"=-40.30997911343495}, {"x"=-0.26388427, "y"=-31.42323318981678}, {"x"=-0.262478602, "y"=-25.676254900728637}, {"x"=-0.260488689, "y"=-26.793751481987233}, {"x"=-0.261151761, "y"=-50.25072068830284}, {"x"=-0.260207725, "y"=-33.47058449389789}, {"x"=-0.258501565, "y"=-66.11387498636887}, {"x"=-0.256827198, "y"=-30.709910555077293}, {"x"=-0.254823982, "y"=-10.486993130828314}, {"x"=-0.257024388, "y"=5.355794391740842}, {"x"=-0.255086829, "y"=-135.48291336062525}, {"x"=-0.253267682, "y"=-88.53928163106502}, {"x"=-0.251461911, "y"=-39.73166399488142}, {"x"=-0.250102396, "y"=-10.449373592025506}, {"x"=-0.25231274, "y"=15.757723289090674}, {"x"=-0.250012497, "y"=-16.25263065261404}, {"x"=-0.248991208, "y"=-31.21033708622895}, {"x"=-0.248949448, "y"=32.69087978467341}, {"x"=-0.246512783, "y"=-15.349415780794109}, {"x"=-0.244667033, "y"=-120.29929472699288}, {"x"=-0.243755129, "y"=2.0104199307576116}, {"x"=-0.241992414, "y"=-13.87212863621082}, {"x"=-0.239839622, "y"=-2.147899914852529}, {"x"=-0.239282604, "y"=-72.71501840668714}, {"x"=-0.239071311, "y"=85.58304946612881}, {"x"=-0.237169503, "y"=94.29524889796443}, {"x"=-0.235139523, "y"=49.001097819057755}, {"x"=-0.233476595, "y"=88.534740711516}, {"x"=-0.231414947, "y"=255.42965913757084}, {"x"=-0.229720153, "y"=-90.83209059162454}, {"x"=-0.227508415, "y"=126.390047915406}, {"x"=-0.225529067, "y"=-69.85108676904218}, {"x"=-0.223780059, "y"=399.6538315235296}, {"x"=-0.22195849, "y"=-38.64914616017509}, {"x"=-0.219702213, "y"=-16.338291585450825}, {"x"=-0.218086488, "y"=-9.77010530747978}, {"x"=-0.216224865, "y"=-9.831728959760657}, {"x"=-0.214102332, "y"=-17.000472864464946}, {"x"=-0.212315332, "y"=34.30723873239667}, {"x"=-0.210746278, "y"=15.982463159879952}, {"x"=-0.208862816, "y"=10.357166739400093}, {"x"=-0.206678716, "y"=19.53667655312523}, {"x"=-0.205282319, "y"=251.06867703778107}, {"x"=-0.203265687, "y"=66.29091035815685}, {"x"=-0.2015471, "y"=-40.208388053165685}, {"x"=-0.199490385, "y"=-16.739106390801485}, {"x"=-0.199987848, "y"=16.108854583101024}, {"x"=-0.19790616, "y"=78.8155775351019}, {"x"=-0.196052649, "y"=57.099122432054074}, {"x"=-0.194518356, "y"=39.64475944658027}, {"x"=-0.19240891, "y"=46.0044166497031}, {"x"=-0.190259549, "y"=63.68981383419547}, {"x"=-0.188408297, "y"=41.59236008996425}, {"x"=-0.186784842, "y"=42.75217996721546}, {"x"=-0.185015955, "y"=43.047637483082376}, {"x"=-0.182885565, "y"=51.645440852629335}, {"x"=-0.18075409, "y"=56.959449472693386}, {"x"=-0.178960146, "y"=31.011885265212012}, {"x"=-0.176972854, "y"=48.64335774088686}, {"x"=-0.17499795, "y"=88.50072100546899}, {"x"=-0.173542057, "y"=103.41259666438079}, {"x"=-0.171253542, "y"=24.75983548360353}, {"x"=-0.169640817, "y"=4.684442115599829}, {"x"=-0.167536408, "y"=2.4852964021051176}, {"x"=-0.165963029, "y"=3.393898661030884}, {"x"=-0.163859733, "y"=7.29219330184644}, {"x"=-0.162155989, "y"=14.455791341608288}, {"x"=-0.16020872, "y"=27.402022275352}, {"x"=-0.158036963, "y"=26.346569101550443}, {"x"=-0.15598597, "y"=35.878813239451745}, {"x"=-0.155628749, "y"=63.59958588335429}, {"x"=-0.153581019, "y"=46.54185675437374}, {"x"=-0.151648848, "y"=41.2359278582794}, {"x"=-0.149635681, "y"=48.62217859415845}, {"x"=-0.147979192, "y"=49.09802925517583}, {"x"=-0.145805958, "y"=51.61865313250581}, {"x"=-0.144300464, "y"=55.598849071984716}, {"x"=-0.142056117, "y"=58.26383132045788}, {"x"=-0.140047045, "y"=84.24264050503085}, {"x"=-0.138373454, "y"=51.78415389001386}, {"x"=-0.136218379, "y"=48.72628747199828}, {"x"=-0.134380383, "y"=89.95319825665834}, {"x"=-0.132730532, "y"=73.63113016615848}, {"x"=-0.130530307, "y"=59.70039431547731}, {"x"=-0.128886387, "y"=58.40586613428}, {"x"=-0.126604636, "y"=84.6741450680825}, {"x"=-0.124698588, "y"=64.19994330340714}, {"x"=-0.122838797, "y"=69.80227048566319}, {"x"=-0.121222399, "y"=68.42837773382726}, {"x"=-0.118909575, "y"=64.87464642469605}, {"x"=-0.117473761, "y"=62.411792088456856}, {"x"=-0.115477579, "y"=177.88775386138653}, {"x"=-0.110103078, "y"=19.01830147037301}, {"x"=-0.108224772, "y"=25.513793137460663}, {"x"=-0.105929355, "y"=25.740163191062837}, {"x"=-0.104081993, "y"=27.745578373192217}, {"x"=-0.102250618, "y"=27.45010655739881}, {"x"=-0.100195133, "y"=31.74483769222833}, {"x"=-0.098527987, "y"=30.416692245283382}, {"x"=-0.0965328678, "y"=36.53976470560146}, {"x"=-0.0942980484, "y"=32.90585052841349}, {"x"=-0.0922350638, "y"=39.40854000304685}, {"x"=-0.0906668875, "y"=37.40590912919674}, {"x"=-0.088716553, "y"=35.8440958881144}, {"x"=-0.0863975638, "y"=46.54183681991643}, {"x"=-0.0846814559, "y"=35.724452263647684}, {"x"=-0.083004609, "y"=42.77468057619818}, {"x"=-0.0810332006, "y"=52.589319160265}, {"x"=-0.0788357726, "y"=46.66388431883844}, {"x"=-0.0772556174, "y"=39.01466606720698}, {"x"=-0.075003195, "y"=50.46275594616215}, {"x"=-0.0734207429, "y"=42.528312834722385}, {"x"=-0.0712544511, "y"=38.21902538829689}, {"x"=-0.069650716, "y"=47.18716107950236}, {"x"=-0.0674068702, "y"=52.547990043020285}, {"x"=-0.0658028379, "y"=51.446075538315114}, {"x"=-0.0638702748, "y"=98.5611940926852}, {"x"=-0.0619029191, "y"=42.13900566312704}, {"x"=-0.0597272892, "y"=42.84335699736388}, {"x"=-0.0578072933, "y"=47.58921185892274}, {"x"=-0.0562117806, "y"=150.59839121536652}, {"x"=-0.05445193, "y"=53.027351625154715}, {"x"=-0.0525810858, "y"=52.88597406501465}, {"x"=-0.0502857008, "y"=53.47479447391408}, {"x"=-0.0486110902, "y"=51.14414708694318}, {"x"=-0.0464787007, "y"=57.8292957513574}, {"x"=-0.0446874833, "y"=53.13467468734832}]
  out "Bias":dbl=-0.05
  in  "NPLC Agi":dbl(ring)=10.0 items=["0.02"=0.02, "0.2"=0.2, "1"=1.0, "10"=10.0, "100"=100.0]
  in  "maxvolt_IV_DMM_abort_condition":dbl=10.0 format="%#_13g"
  out "initial valuefirst sweep":dbl=-0.05
  out "bias after mainsweep":dbl=-0.39000000000000024
  in  "min_LIA1_abort":dbl=1e-06
  in  "max_LIA1_abort":dbl=10.2
  in  "PLC_DMM_6500":dbl(ring)=0.2 items=["0.001"=0.001, "0.002"=0.002, "0.006"=0.006, "0.02"=0.02, "0.06"=0.06, "10"=0.2, "1"=1.0, "10"=10.0, "100"=100.0]
  in  "Set0 delay time (s)":dbl=0.7 caption="Delay Time (s)"
  in  "Delay Time (s)":dbl=1.0
  out "prefactor 2":dbl=0.0028681236734928017
  out "prefactor1":dbl=8.604269152950089
  in  "chart buffer":i32=750
  in  "bias_factor":dbl=-1.0
  in  "yoko_range":string="1V"
  in  "Reset graph":bool
  in  "VISA Agilent in":refnum<visa-resource-name>="GPIB0::10::INSTR"
  in  "34461A_2_Adrs":refnum<visa-resource-name>="USB0::0x2A8D::0x1401::MY57230853::INSTR"
  in  "Keith_DMM_VISA":refnum<visa-resource-name>="USB0::0x05E6::0x6500::04446089::INSTR"
  in  "34461A_1 Adrs":refnum<visa-resource-name>="USB0::0x2A8D::0x1401::MY59000923::INSTR"
  out "format ms":string="H:10:34,6412"
  out "LabVIEW TimeStamp":timestamp=timestamp(3700023034.641244 s since 1904-01-01)
  # "Abort sweeps"
  # "DMM_settings"
  # "Check"
  # "Sweep Settings"
  # "From Main Programm"
  # "Constants for calculations"
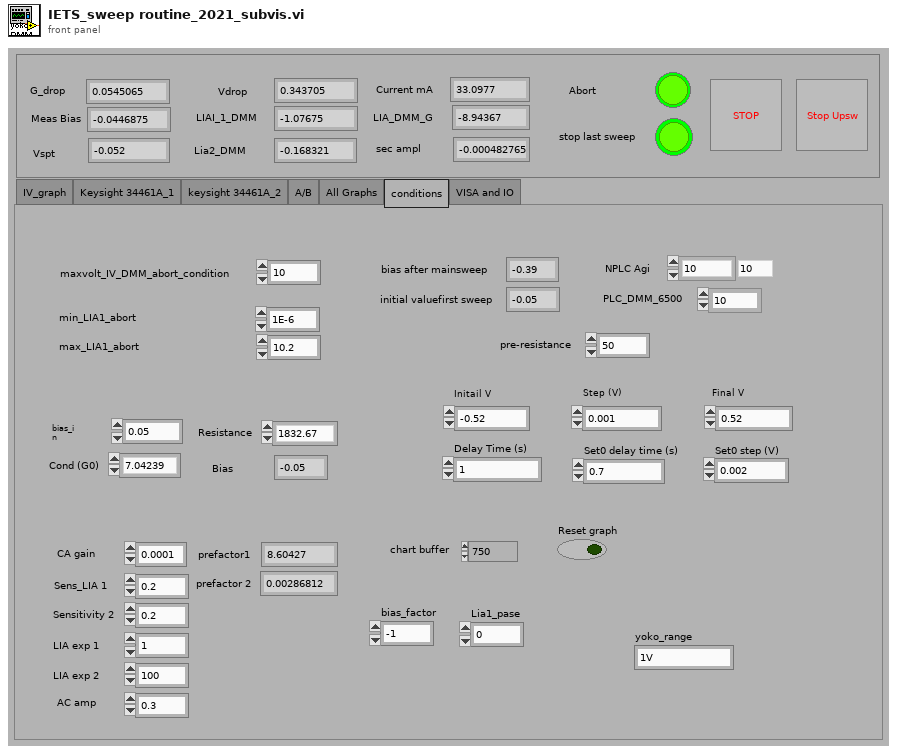
[diagram p1: front panel]
types:
  T1 = enum32{"IV_graph", "Keysight 34461A_1", "keysight 34461A_2", "A/B", "All Graphs", "conditions", "VISA and IO"}
  T2 = enum16{"open", "open or create", "create or replace", "create", "open (read only)"}
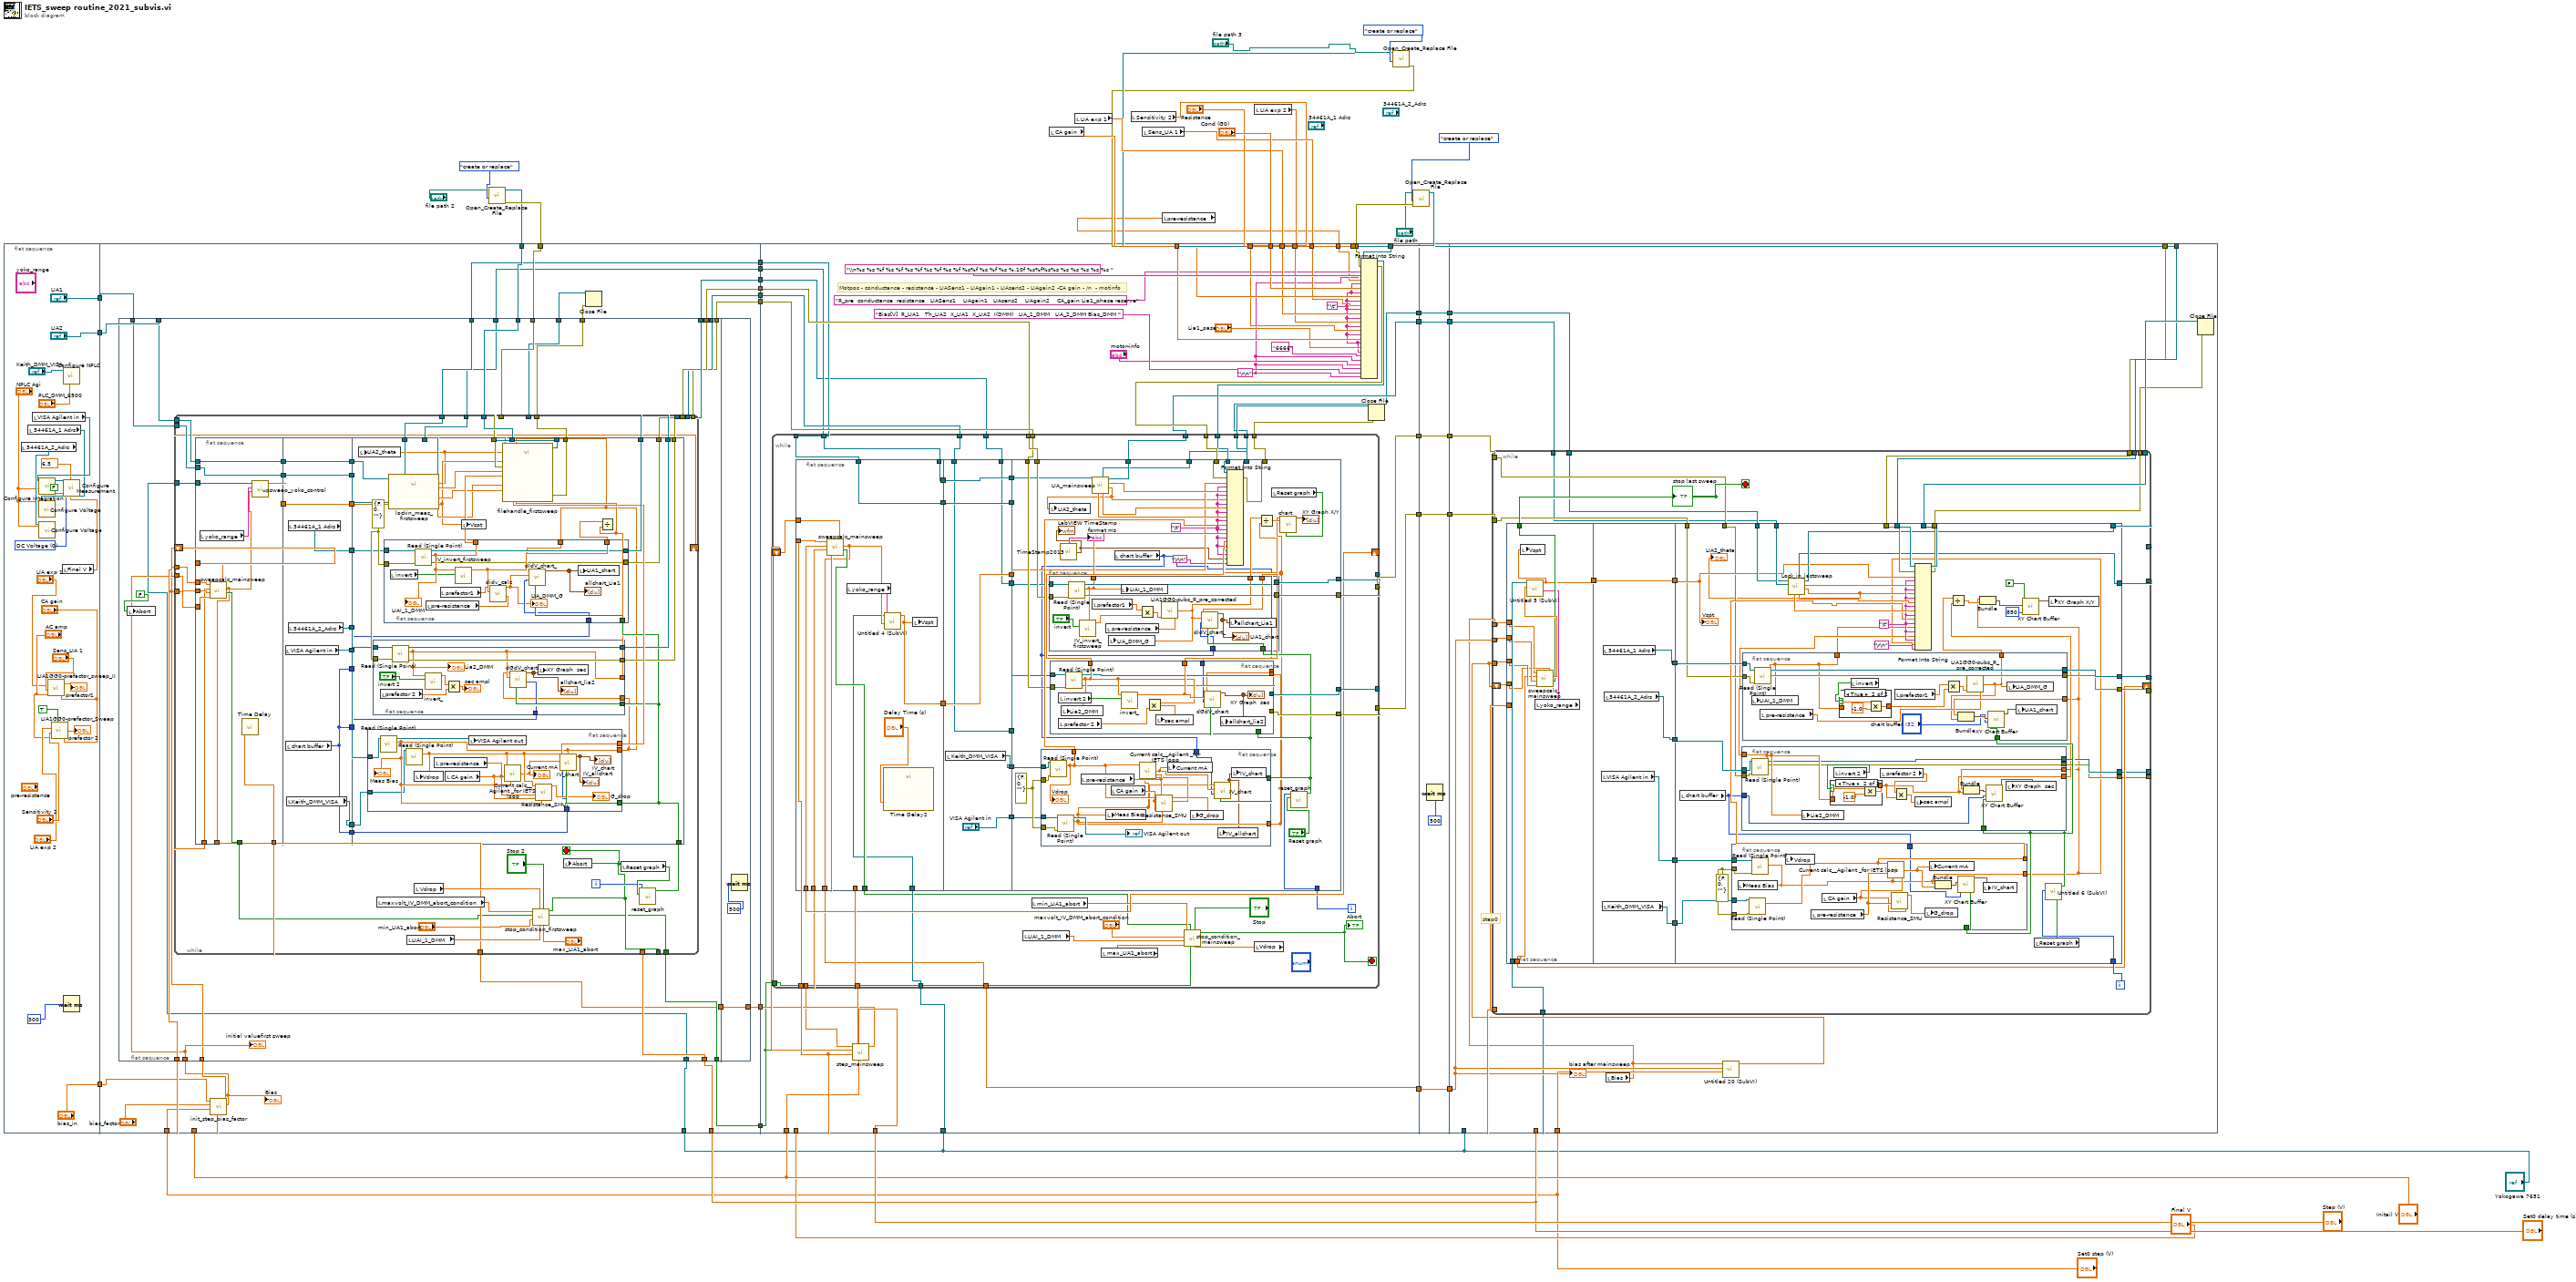
[diagram p0: block diagram]
diagram:
  n1 = flat-sequence {
    tunnel: ["bias_in"] -> w13
    tunnel: ["LIA1"] -> w6
    tunnel: ["LIA2"] -> w5
    tunnel: "Set0 delay time (s)" -> [w94]
    tunnel: "Initail V" -> [w82]
    tunnel: w28 -> [w93]
    tunnel: w29 -> [w92]
    tunnel: [w91] -> w33
    tunnel: [w90] -> w32
    tunnel: [w89] -> w31
    tunnel: [w88] -> w30
    tunnel: [w85] -> w21
    tunnel: [w84] -> w20
    tunnel: w13 -> [w74]
    tunnel: [w81] -> w8
    tunnel: [w79] -> w7
    tunnel: w6 -> [w78]
    tunnel: w5 -> [w77]
    tunnel: "Set0 step (V)" -> [w76]
    tunnel: "Yokogawa 7651" -> [w75]
    tunnel: "Step (V)" -> [w270]
    tunnel: "Final V" -> [w269]
    tunnel: "Initail V" -> [w263]
    tunnel: w42 -> [w290]
    tunnel: w41 -> [w291]
    tunnel: "Cond (G0)" -> [w287]
    tunnel: "Resistance" -> [w286]
    tunnel: w37 -> [w284]
    tunnel: w36 -> [w285]
    tunnel: w35 -> [w280]
    tunnel: w19 -> [w283]
    tunnel: w34 -> [w282]
    tunnel: w33 -> [w253]
    tunnel: w32 -> [w276]
    tunnel: w31 -> [w278]
    tunnel: w30 -> [w277]
    tunnel: [w275] -> w18
    tunnel: [w274] -> w17
    tunnel: w21 -> [w264]
    tunnel: w20 -> [w265]
    tunnel: [w273] -> w16
    tunnel: [w272] -> w15
    tunnel: "Yokogawa 7651" -> [w268]
    tunnel: [w266] -> w14
    tunnel: w8 -> [w254]
    tunnel: w7 -> [w262]
    tunnel: w1 -> [w260]
    tunnel: [w445] -> w12
    tunnel: [w444] -> w11
    tunnel: [w443] -> w10
    tunnel: [w442] -> w9
    tunnel: w14 -> [w442]
    tunnel: w15 -> [w443]
    tunnel: w16 -> [w444]
    tunnel: w17 -> [w445]
    tunnel: w18 -> [w440]
    tunnel: [w440] -> w2
    tunnel: "Set0 step (V)" -> [w453]
    tunnel: "Set0 delay time (s)" -> [w454]
    tunnel: w23 -> [w457]
    tunnel: w22 -> [w456]
    tunnel: w12 -> [w455]
    tunnel: w11 -> [w449]
    tunnel: w10 -> [w450]
    tunnel: w9 -> [w451]
    tunnel: "Yokogawa 7651" -> [w448]
    tunnel: w2 -> [w447]
    frame #0 {
      w48 = u16 0 items=["DC Voltage", "AC Voltage", "2 - Wire Resistance", "4 - Wire Resistance", "DC Current", "AC Current", "Frequency", "Period", "Continuity", "Diode Checking", "VDC:VDC Ratio", "Temperature", "Capacitance"] ("Function (0: DC Voltage)")
      w50 = 6.5 items=["4.5"=4.5, "5.5"=5.5, "6.5"=6.5] ("Manual Resolution (5.5 Digits)")
      (unwired) FALSE ("Enable Auto Range (T: Enable)")
      n2 = local read "34461A_2_Adrs"() -> (w55:refnum<visa-resource-name>)
      n3 = local read "34461A_1 Adrs"() -> (w56:refnum<visa-resource-name>)
      n4 = local read "VISA Agilent in"() -> (w57:refnum<visa-resource-name>)
      n5 = call "Configure Voltage.vi"("Voltage Integration Time (10: 10)"="NPLC Agi", "VISA resource name"=w56) -> ()  [unwired: 8 in, 2 out]
      n6 = call "Configure Integration.vi"("Integration Time (1 PLCs)"="NPLC Agi", "VISA resource name"=w57) -> ("error out"=w52:errorcluster, "VISA resource name out"=w51:refnum<visa-resource-name>)  [unwired: 8 in]
      n7 = call "Configure Voltage.vi"("Voltage Integration Time (10: 10)"="NPLC Agi", "VISA resource name"=w55) -> ()  [unwired: 8 in, 2 out]
      n8 = call "LIA1GG0-prefactor_sweep_II.vi"("CA gain"="CA gain", "AC amp"="AC amp", "Sensitivity"="Sens_LIA 1", "Expand"="LIA exp 1") -> ("prefactor_[S]"=→"prefactor1":dbl)  [unwired: 3 in]
      n9 = call "LIA1GG0-prefactor_Sweep.vi"("2nd Harm"=TRUE, "Expand"="LIA exp 2", "Sensitivity"="Sensitivity 2", "AC amp"="AC amp", "CA gain"="CA gain") -> ("prefactor"=→"prefactor 2":dbl)  [unwired: 3 in]
      n10 = local read "Final V"() -> (w49:dbl)
      n11 = call "Configure NPLC.vi"("Power Line Cycle (1)"="PLC_DMM_6500", "VISA resource name"="Keith_DMM_VISA") -> ()  [unwired: 8 in, 2 out]
      n12 = Wait (ms)(milliseconds to wait=u32 300) -> ()  [unwired: 1 out]
      n13 = call <instrlib>:"Configure Measurement.vi"("Manual Range (1.00)"=w49, "Manual Resolution (5.5 Digits)"=w50, "error in (no error)"=w52, "Function (0: DC Voltage)"=w48, "VISA resource name"=w51) -> ()  [unwired: 5 in, 2 out]
    }
    frame #1 {
      n14 = flat-sequence {
        tunnel: w94 -> [w106]
        tunnel: w82 -> [w103]
        tunnel: w93 -> [w114]
        tunnel: w92 -> [w113]
        tunnel: [w112] -> w91
        tunnel: [w111] -> w90
        tunnel: [w110] -> w89
        tunnel: [w109] -> w88
        tunnel: [w108] -> w87
        tunnel: [w107] -> w86
        tunnel: [w105] -> w85
        tunnel: [w99] -> w84
        tunnel: w83 -> [w96]
        tunnel: w72 -> [w102]
        tunnel: w75 -> [w95]
        tunnel: [w101] -> w81
        tunnel: [w100] -> w80
        tunnel: w78 -> [w98]
        tunnel: w77 -> [w97]
        tunnel: w80 -> [w251]
        tunnel: [w251] -> w79
        frame #0 {
          n15 = local write "Abort"(FALSE) -> ()
          n16 = while {
            tunnel: w114 -> [w159]
            tunnel: w113 -> [w158]
            tunnel: [w145] -> w112
            tunnel: [w146] -> w111
            tunnel: [w157] -> w110
            tunnel: [w156] -> w109
            tunnel: [w155] -> w108
            tunnel: [w154] -> w107
            tunnel: w95 -> [w153]
            tunnel: w96 -> [w152]
            tunnel: w106 -> [w151]
            tunnel: [w150] -> w105
            tunnel: [w149] -> w99
            tunnel: w98 -> [w148]
            tunnel: w97 -> [w147]
            tunnel: [w118] -> _
            tunnel: w102 -> [w138]
            tunnel: w103 -> [w137]
            shift-right: [w136] -> _
            shift-left: w96 -> [w135]
            tunnel: [w117] -> w101
            tunnel: [w134] -> w100
            i -> [w139]
            stop <- w118 stop-if-true
            n17 = flat-sequence {
              tunnel: w151 -> [w172]
              tunnel: w152 -> [w170]
              tunnel: w153 -> [w171]
              tunnel: [w164] -> w116
              tunnel: [w162] -> w132
              tunnel: [w161] -> w130
              tunnel: w148 -> [w162]
              tunnel: w147 -> [w161]
              tunnel: w138 -> [w169]
              tunnel: w137 -> [w168]
              tunnel: [w167] -> w136
              tunnel: w135 -> [w166]
              tunnel: [w165] -> w128
              tunnel: [w163] -> w134
              tunnel: w132 -> [w180]
              tunnel: [w180] -> w131
              tunnel: w130 -> [w179]
              tunnel: [w179] -> w129
              tunnel: w128 -> [w178]
              tunnel: [w178] -> w127
              tunnel: [w174] -> w126
              tunnel: [w177] -> w125
              tunnel: [w176] -> w124
              tunnel: [w175] -> w123
              tunnel: [w173] -> w122
              tunnel: [w173] -> w121
              tunnel: [w173] -> w120
              tunnel: w159 -> [w209]
              tunnel: w158 -> [w208]
              tunnel: [w207] -> w145
              tunnel: [w205] -> w146
              tunnel: [w204] -> w157
              tunnel: [w203] -> w156
              tunnel: [w202] -> w155
              tunnel: [w201] -> w154
              tunnel: [w197] -> w150
              tunnel: [w196] -> w149
              tunnel: w131 -> [w195]
              tunnel: w129 -> [w194]
              tunnel: w141 -> [w193]
              tunnel: w127 -> [w190]
              tunnel: w126 -> [w186]
              tunnel: w125 -> [w188]
              tunnel: w124 -> [w189]
              tunnel: w123 -> [w187]
              tunnel: w122 -> [w185]
              tunnel: w121 -> [w184]
              tunnel: w120 -> [w183]
              frame #0 {
                n18 = local read "yoko_range"() -> (w160:string)
                n19 = call "sweepcalc_mainsweep.vi"("loop in"=w166, "step"=w170, "initial"=w169, "final"=w168) -> ("stop condition"=w164:bool, "value to write"=w163:dbl, "loop out"=w167:dbl)  [unwired: 1 in]
                n20 = call "Time Delay"("Delay Time (s)"=w172) -> ()  [unwired: 10 in, 1 out]
                n21 = call "upsweep_yoko_control.vi"("value to write"=w163, "yoko_range"=w160, "VISA Refnum in"=w171) -> ("Numeric"=w165:dbl)  [unwired: 8 in]
              }
              frame #1 {
                n22 = local read "VISA Agilent in"() -> (w175:refnum<visa-resource-name>)
                n23 = local read "chart buffer"() -> (w173:i32)
                n24 = local read "Keith_DMM_VISA"() -> (w174:refnum<visa-resource-name>)
                n25 = local read "34461A_1 Adrs"() -> (w177:refnum<visa-resource-name>)
                n26 = local read "34461A_2_Adrs"() -> (w176:refnum<visa-resource-name>)
              }
              frame #2 {
                w191 = errorcluster {"status"=FALSE, "code"=0, "source"=""} ("error in (no error)")
                n27 = flat-sequence {
                  tunnel: [w250] -> w206
                  tunnel: [w249] -> w181
                  tunnel: w193 -> [w248]
                  tunnel: w187 -> [w242]
                  tunnel: w186 -> [w241]
                  tunnel: w185 -> [w240]
                  frame #0 {
                    n28 = call "Read (Single Point).vi"("VISA resource name"=w242) -> ("Measurement"=w249:dbl, "VISA resource name out"=w243:refnum<visa-resource-name>)  [unwired: 8 in, 1 out]
                    "Meas Bias" <- w249
                    n29 = call "Read (Single Point).vi"("VISA resource name"=w241) -> ("Measurement"=w250:dbl)  [unwired: 12 in, 2 out]
                    n30 = local write "Vdrop"(w250) -> ()
                    n31 = local read "pre-resistance"() -> (w245:dbl)
                    n32 = local read "CA gain"() -> (w246:dbl)
                    n33 = local write "VISA Agilent out"(w243) -> ()
                    n34 = call "Current calc__Agilent _for IETS loop.vi"("Vdrop"=w250, "pre-resistance"=w245, "Measurement Voltage"=w249, "CA gain"=w246) -> ("Current"=w247:dbl)  [unwired: 11 in]
                    "Current mA" <- w247
                    n35 = call "Resistance_SMU.vi"("CA gain"=w246, "Measurement Voltage"=w249, "cable and pre-resistance"=w245, "Input Value"=w250) -> ("Output conductance"=→"G_drop":dbl)  [unwired: 6 in, 1 out]
                    n36 = call "IV_chart.vi"("Boolean"=w248, "chart buffer"=w240, "G_subsR_pre"=w247, "Measurement"=w249) -> ("XY chart data"=→"IV_chart" →"IV_allchart":cluster{"x":dbl, "y":dbl}[])  [unwired: 7 in]
                  }
                }
                n37 = flat-sequence {
                  tunnel: [w238] -> w204
                  tunnel: [w237] -> w203
                  tunnel: w193 -> [w236]
                  tunnel: w181 -> [w226]
                  tunnel: [w227] -> w192
                  tunnel: w191 -> [w235]
                  tunnel: w189 -> [w234]
                  tunnel: w184 -> [w231]
                  frame #0 {
                    n38 = local read "prefactor 2"() -> (w230:dbl)
                    n39 = call "Read (Single Point).vi"("error in (no error)"=w235, "VISA resource name"=w234) -> ("error out"=w237:errorcluster, "Measurement"=w227:dbl, "VISA resource name out"=w238:refnum<visa-resource-name>)  [unwired: 7 in]
                    "Lia2_DMM" <- w227
                    n40 = call "invert_.vi"("invert in"="invert 2", "Measurement in"=w227) -> ("Measurement out"=w229:dbl)  [unwired: 9 in]
                    n41 = Multiply(x=w229, y=w230) -> (x*y=→"sec ampl":dbl)
                    n42 = call "dGdV_chart.vi"("Boolean"=w236, "chart buffer"=w231, "G_subsR_pre"=w227, "Measurement"=w226) -> ("XY chart data"=w228:cluster{"x":dbl, "y":dbl}[])  [unwired: 7 in]
                    "allchart_lia2" <- w228
                    n43 = local write "XY Graph  sec"(w228) -> ()
                  }
                }
                n44 = flat-sequence {
                  tunnel: [w225] -> w211
                  tunnel: [w224] -> w210
                  tunnel: [w223] -> w207
                  tunnel: [w222] -> w205
                  tunnel: w193 -> [w221]
                  tunnel: w181 -> [w220]
                  tunnel: w191 -> [w219]
                  tunnel: w188 -> [w218]
                  tunnel: w183 -> [w215]
                  frame #0 {
                    n45 = local read "invert"() -> (w217:bool)
                    n46 = call "Read (Single Point).vi"("error in (no error)"=w219, "VISA resource name"=w218) -> ("error out"=w222:errorcluster, "Measurement"=w224:dbl, "VISA resource name out"=w223:refnum<visa-resource-name>)  [unwired: 7 in]
                    "LIAI_1_DMM" <- w224
                    n47 = local read "pre-resistance"() -> (w214:dbl)
                    n48 = local read "prefactor1"() -> (w216:dbl)
                    n49 = call "IV_invert_firstsweep.vi"("invert"=w217, "Measurement in"=w224) -> ("Measurement out"=w225:dbl)  [unwired: 9 in]
                    n50 = call "didv_calc.vi"("pre-resistance"=w214, "Measurement"=w225, "prefactor1"=w216) -> ("G_subsR_pre"=w213:dbl)  [unwired: 8 in]
                    "LIA_DMM_G" <- w213
                    n51 = call "dIdV_chart_.vi"("Boolean"=w221, "chart buffer"=w215, "G_subsR_pre"=w213, "Measurement"=w220) -> ("XY chart data"=w212:cluster{"x":dbl, "y":dbl}[])  [unwired: 7 in]
                    "allchart_Lia1" <- w212
                    n52 = local write "LIA1_chart"(w212) -> ()
                  }
                }
                n53 = call "lockin_meas_firstsweep.vi"("LIA1"=w195, "VISA Refnum in"=w194) -> ("Measurement 2"=w198:dbl, "Measurement"=w182:dbl, "VISA Refnum out"=w197:refnum<visa-resource-name>, "Measurement 3"=w199:dbl, "VISA resource name out"=w196:refnum<visa-resource-name>, "Measurement 4"=w200:dbl)  [unwired: 4 in]
                n54 = local write "LIA2_theta"(w182) -> ()
                n55 = local write "Vspt"(w190) -> ()
                n56 = call "filehandle_firstsweep.vi"("Byte Stream File in"=w209, "Measurement 7"=w206, "Measurement 6"=w200, "Measurement 5"=w199, "Measurement 2"=w182, "Measurement"=w181, "Numeric"=w190, "error in (no error)"=w208, "Measurement 4"=w198, "Measurement 8"=w210, "Measurement 3"=w192) -> ("Byte Stream File out"=w202:refnum<file>, "error out"=w201:errorcluster)  [unwired: 3 in]
                n57 = Divide(x=w211, y=w192) -> ()  [unwired: 1 out]
              }
            }
            n58 = local read "maxvolt_IV_DMM_abort_condition"() -> (w143:dbl)
            n59 = local read "LIAI_1_DMM"() -> (w142:dbl)
            n60 = local read "Vdrop"() -> (w144:dbl)
            n61 = call "stop_condition_firstsweep.vi"("max_LIA1_abort"="max_LIA1_abort", "Stop in"="Stop 2", "LIAI_1_DMM"=w142, "Vdrop"=w144, "min_LIA1_abort"="min_LIA1_abort", "stop condition"=w116, "maxvolt_IV_DMM_abort_condition"=w143) -> ("Boolean"=w117:bool, "Boolean 2"=w118:bool)  [unwired: 3 in]
            n62 = local write "Abort"(w118) -> ()
            n63 = local read "Reset graph"() -> (w140:bool)
            n64 = call "reset_graph.vi"("Reset graph"=w140, "Numeric"=w139) -> ("Boolean"=w141:bool)  [unwired: 9 in]
          }
          "initial valuefirst sweep" <- w102
        }
        frame #1 {
          n65 = Wait (ms)(milliseconds to wait=u32 500) -> ()  [unwired: 1 out]
        }
      }
      n66 = call "init_step_bias_factor.vi"("Initail V"=w82, "Set0 step (V) in"=w76, "bias_factor"="bias_factor", "bias_in"=w74) -> ("Numeric"=w72:dbl, "Set0 step (V) out"=w83:dbl)  [unwired: 6 in]
      "Bias" <- w72
      n67 = Close File(refnum=w87, error in=w86) -> ()  [unwired: 2 out]
    }
    frame #2 {
      w256 = "\t"
      w257 = "\r\n"
      # "Motpos - conductance - resistance - LIASens1 - LIAgain1 - LIAsens2 - LIAgain2 -CA gain - /n  - motinfo"
      n68 = call "step_mainsweep.vi"("Initail V"=w263, "Step (V) in"=w270, "Final V"=w269, "Boolean"=w254, "value to write in"=w262) -> ("Step (V) out"=w267:dbl, "value to write out"=w261:dbl)  [unwired: 5 in]
      n69 = Format Into String(format string="\\n%s %s %f %s %f %s %f %s %f %s %f %s%f %s %f %s %.10f %s%f%s%s %s %s %s %s %s ", initial string=w291, error in=w290, "R_pre  conductance  resistance   LIASens1    LIAgain1   LIAsens2    LIAgain2    CA_gain Lia1_phase reserve" ("input 18"), w257, w260, w256, w287, w256, w286, w256, w285, w256, w284, w256, w280, w256, w283, w256, w282, w256, "Lia1_pase", w256, "6666" ("input 25"), w257, "motor-info", w257, "Bias[V]  R_LIA1   Th_LIA2  X_LIA1  X_LIA2  I(DMM)   LIA_1_DMM   LIA_2_DMM Bias_DMM " ("input 22"), w257) -> (resulting string=w281:refnum<file>, error out=w289:errorcluster)
      n70 = while {
        tunnel: w269 -> [w324]
        tunnel: [w336] -> _
        tunnel: [w335] -> w274
        tunnel: [w334] -> _
        tunnel: [w333] -> w275
        tunnel: [w332] -> w292
        tunnel: [w331] -> w293
        tunnel: w289 -> [w330]
        tunnel: w281 -> [w329]
        tunnel: w276 -> [w328]
        tunnel: w278 -> [w308]
        tunnel: w277 -> [w327]
        tunnel: [w326] -> w273
        tunnel: [w325] -> w272
        tunnel: w267 -> [w323]
        shift-right: [w322] -> _
        shift-left: w267 -> [w321]
        tunnel: w268 -> [w320]
        tunnel: [w319] -> w266
        tunnel: w254 -> [w296]
        tunnel: w265 -> [w318]
        tunnel: w264 -> [w317]
        tunnel: w261 -> [w316]
        tunnel: w253 -> [w309]
        i -> [w304]
        stop <- w294 stop-if-true
        n71 = flat-sequence {
          tunnel: [w344] -> w315
          tunnel: w320 -> [w341]
          tunnel: w324 -> [w349]
          tunnel: [w345] -> w295
          tunnel: w323 -> [w348]
          tunnel: [w346] -> w322
          tunnel: w321 -> [w347]
          tunnel: [w343] -> w319
          tunnel: w316 -> [w342]
          tunnel: w318 -> [w339]
          tunnel: w317 -> [w338]
          tunnel: [w338] -> w313
          tunnel: [w339] -> w311
          tunnel: w315 -> [w356]
          tunnel: [w356] -> w314
          tunnel: w313 -> [w355]
          tunnel: [w355] -> w312
          tunnel: w311 -> [w354]
          tunnel: [w354] -> w310
          tunnel: w309 -> [w353]
          tunnel: w308 -> [w352]
          tunnel: [w352] -> w307
          tunnel: [w353] -> w306
          tunnel: [w351] -> w305
          tunnel: ["VISA Agilent in"] -> w303
          tunnel: w314 -> [w372]
          tunnel: [w397] -> w336
          tunnel: [w396] -> w335
          tunnel: [w374] -> w334
          tunnel: [w375] -> w333
          tunnel: [w395] -> w332
          tunnel: [w394] -> w331
          tunnel: w330 -> [w393]
          tunnel: w329 -> [w389]
          tunnel: w328 -> [w387]
          tunnel: w327 -> [w386]
          tunnel: [w381] -> w326
          tunnel: [w380] -> w325
          tunnel: w312 -> [w379]
          tunnel: w310 -> [w378]
          tunnel: w307 -> [w376]
          tunnel: w306 -> [w377]
          tunnel: w305 -> [w367]
          tunnel: w304 -> [w369]
          tunnel: w303 -> [w368]
          frame #0 {
            n72 = call "sweepcalc_mainsweep.vi"("loop in"=w347, "step"=w348, "initial"=w342, "final"=w349) -> ("stop condition"=w345:bool, "value to write"=w343:dbl, "loop out"=w346:dbl)  [unwired: 1 in]
            n73 = local read "yoko_range"() -> (w337:string)
            n74 = call "Time Delay2"("Delay Time (s)"="Delay Time (s)") -> ()  [unwired: 10 in, 1 out]
            n75 = call "Untitled 4 (SubVI).vi"("value to write"=w343, "yoko_range"=w337, "VISA Refnum in"=w341) -> ("Numeric"=w344:dbl)  [unwired: 8 in]
            n76 = local write "Vspt"(w344) -> ()
          }
          frame #1 {
            n77 = local read "Keith_DMM_VISA"() -> (w351:refnum<visa-resource-name>)
          }
          frame #2 {
            w370 = errorcluster {"status"=FALSE, "code"=0, "source"=""} ("error out")
            w365 = "\t"
            n78 = flat-sequence {
              tunnel: w371 -> [w426]
              tunnel: [w418] -> w391
              tunnel: [w416] -> w362
              tunnel: w370 -> [w420]
              tunnel: w370 -> [w414]
              tunnel: w368 -> [w421]
              tunnel: w367 -> [w419]
              tunnel: w361 -> [w415]
              frame #0 {
                n79 = call "Read (Single Point).vi"("VISA resource name"=w419, "error in (no error)"=w414) -> ("Measurement"=w418:dbl)  [unwired: 11 in, 2 out]
                "Vdrop" <- w418
                n80 = call "Read (Single Point).vi"("error in (no error)"=w420, "VISA resource name"=w421) -> ("Measurement"=w416:dbl, "VISA resource name out"=→"VISA Agilent out":refnum<visa-resource-name>)  [unwired: 7 in, 1 out]
                n81 = local read "pre-resistance"() -> (w424:dbl)
                n82 = local write "Meas Bias"(w416) -> ()
                n83 = local read "CA gain"() -> (w422:dbl)
                n84 = call "Current calc__Agilent _for IETS loop.vi"("Vdrop"=w418, "pre-resistance"=w424, "Measurement Voltage"=w416, "CA gain"=w422) -> ("Current"=w425:dbl)  [unwired: 11 in]
                n85 = call "Resistance_SMU.vi"("CA gain"=w422, "Measurement Voltage"=w416, "cable and pre-resistance"=w424, "Input Value"=w418) -> ("Output conductance"=w423:dbl)  [unwired: 6 in, 1 out]
                n86 = local write "Current mA"(w425) -> ()
                n87 = local write "G_drop"(w423) -> ()
                n88 = call "IV_chart.vi"("Boolean"=w426, "chart buffer"=w415, "G_subsR_pre"=w425, "Measurement"=w416) -> ("XY chart data"=w413:cluster{"x":dbl, "y":dbl}[])  [unwired: 7 in]
                n89 = local write "IV_allchart"(w413) -> ()
                n90 = local write "IV_chart"(w413) -> ()
              }
            }
            n91 = flat-sequence {
              tunnel: [w412] -> w397
              tunnel: [w411] -> w396
              tunnel: w371 -> [w410]
              tunnel: [w409] -> w388
              tunnel: w387 -> [w408]
              tunnel: w362 -> [w407]
              tunnel: w377 -> [w406]
              tunnel: [w399] -> w373
              tunnel: w361 -> [w402]
              frame #0 {
                n92 = call "Read (Single Point).vi"("error in (no error)"=w408, "VISA resource name"=w406) -> ("error out"=w411:errorcluster, "Measurement"=w409:dbl, "VISA resource name out"=w412:refnum<visa-resource-name>)  [unwired: 7 in]
                n93 = call "IV_invert_firstsweep.vi"("invert"="invert", "Measurement in"=w409) -> ("Measurement out"=w403:dbl)  [unwired: 9 in]
                n94 = local read "prefactor1"() -> (w404:dbl)
                n95 = local read "pre-resistance"() -> (w400:dbl)
                n96 = local write "LIAI_1_DMM"(w409) -> ()
                n97 = Multiply(x=w404, y=w403) -> (x*y=w401:dbl)
                n98 = call "LIA1GG0-subs_R_pre_corrected.vi"("LIA_G_all"=w401, "R_pre"=w400) -> ("G_subsR_pre"=w399:dbl)  [unwired: 6 in]
                n99 = local write "LIA_DMM_G"(w399) -> ()
                n100 = call "dIdV_chart_.vi"("Boolean"=w410, "chart buffer"=w402, "G_subsR_pre"=w399, "Measurement"=w407) -> ("XY chart data"=w398:cluster{"x":dbl, "y":dbl}[])  [unwired: 7 in]
                "LIA1_chart" <- w398
                n101 = local write "allchart_Lia1"(w398) -> ()
              }
            }
            n102 = flat-sequence {
              tunnel: [w439] -> w392
              tunnel: w371 -> [w438]
              tunnel: [w437] -> w390
              tunnel: w386 -> [w436]
              tunnel: [w428] -> _
              tunnel: w376 -> [w435]
              tunnel: [w431] -> w374
              tunnel: [w430] -> w375
              tunnel: w361 -> [w429]
              tunnel: w362 -> [w428]
              frame #0 {
                n103 = local read "invert 2"() -> (w434:bool)
                n104 = local read "prefactor 2"() -> (w432:dbl)
                n105 = call "Read (Single Point).vi"("error in (no error)"=w436, "VISA resource name"=w435) -> ("error out"=w430:errorcluster, "Measurement"=w437:dbl, "VISA resource name out"=w431:refnum<visa-resource-name>)  [unwired: 7 in]
                n106 = local write "Lia2_DMM"(w437) -> ()
                n107 = call "invert_.vi"("invert in"=w434, "Measurement in"=w437) -> ("Measurement out"=w439:dbl)  [unwired: 9 in]
                n108 = Multiply(x=w437, y=w432) -> (x*y=w433:dbl)
                n109 = local write "sec ampl"(w433) -> ()
                n110 = call "dGdV_chart.vi"("Boolean"=w438, "chart buffer"=w429, "G_subsR_pre"=w439, "Measurement"=w428) -> ("XY chart data"=w427:cluster{"x":dbl, "y":dbl}[])  [unwired: 7 in]
                "XY Graph  sec" <- w427
                n111 = local write "allchart_lia2"(w427) -> ()
              }
            }
            n112 = call "TimeStamp2013.vi"() -> ("LabVIEW TimeStamp"=w363:timestamp, "Date Formatted with Milliseconds"=→"format ms":string)  [unwired: 1 in]
            "LabVIEW TimeStamp" <- w363
            n113 = call "LIA_mainsweep.vi"(10:"VISA Refnum in"=w379, 11:"VISA Refnum in"=w378) -> ("Measurement"=w357:dbl, "Measurement 4"=w384:dbl, "VISA Refnum out"=w381:refnum<visa-resource-name>, "Measurement 3"=w383:dbl, "VISA resource name out 2"=w380:refnum<visa-resource-name>, "Measurement 2"=w382:dbl)  [unwired: 4 in]
            n114 = local write "LIA2_theta"(w357) -> ()
            n115 = local read "chart buffer"() -> (w361:i32)
            n116 = Format Into String(initial string=w389, error in=w393, w372, w365, w384, w365, w357, w365, w383, w365, w382, w365, w391, w365, w388, w365, w390, w365, w362, w365, w363, "\r\n") -> (resulting string=w395:refnum<file>, error out=w394:errorcluster)  [unwired: 1 in]
            n117 = Divide(x=w373, y=w392) -> (x/y=w385:dbl)
            n118 = local read "Reset graph"() -> (w358:bool)
            n119 = call "chart.vi"("Boolean"=w358, "G_subsR_pre"=w385, "Measurement"=w362) -> ("XY chart data"=→"XY Graph X/Y":cluster{"x":dbl, "y":dbl}[])  [unwired: 8 in]
            n120 = call "reset_graph.vi"("Reset graph"="Reset graph", "Numeric"=w369) -> ("Boolean"=w371:bool)  [unwired: 9 in]
          }
        }
        n121 = local read "LIAI_1_DMM"() -> (w300:dbl)
        n122 = local read "min_LIA1_abort"() -> (w301:dbl)
        n123 = local read "max_LIA1_abort"() -> (w299:dbl)
        n124 = local read "Vdrop"() -> (w298:dbl)
        n125 = call "stop_condition_mainsweep.vi"("Vdrop"=w298, "Stop"="Stop", "Boolean in"=w296, "stop condition"=w295, "max_LIA1_abort"=w299, "LIAI_1_DMM"=w300, "maxvolt_IV_DMM_abort_condition"="maxvolt_IV_DMM_abort_condition", "min_LIA1_abort"=w301) -> ("Boolean out"=w294:bool)  [unwired: 3 in]
        "Abort" <- w294
      }
      n126 = Close File(refnum=w292, error in=w293) -> ()  [unwired: 2 out]
    }
    frame #3 {
      n127 = Wait (ms)(milliseconds to wait=u32 500) -> ()  [unwired: 1 out]
    }
    frame #4 {
      # "step0"
      n128 = local read "Bias"() -> (w446:dbl)
      n129 = call "Untitled 20 (SubVI).vi"("Set0 step (V) in"=w453, "value to write"=w451, "Bias"=w446) -> ("Set0 step (V) out"=w452:dbl)  [unwired: 8 in]
      n130 = while {
        tunnel: w454 -> [w488]
        tunnel: w455 -> [w465]
        tunnel: [w487] -> w459
        tunnel: [w486] -> w458
        tunnel: w457 -> [w485]
        tunnel: w456 -> [w484]
        tunnel: w447 -> [w466]
        tunnel: [w483] -> _
        tunnel: [w482] -> _
        tunnel: [w481] -> _
        tunnel: [w480] -> _
        tunnel: w448 -> [w478]
        tunnel: w451 -> [w477]
        tunnel: w452 -> [w476]
        shift-right: [w475] -> _
        shift-left: w452 -> [w474]
        tunnel: w446 -> [w473]
        tunnel: w450 -> [w461]
        tunnel: w449 -> [w460]
        tunnel: [w468] -> _
        tunnel: [w467] -> _
        i -> [w479]
        stop <- w472 stop-if-true
        n131 = flat-sequence {
          tunnel: [w493] -> w472
          tunnel: w488 -> [w499]
          tunnel: w478 -> [w498]
          tunnel: [w491] -> w471
          tunnel: w477 -> [w497]
          tunnel: w476 -> [w496]
          tunnel: [w492] -> w475
          tunnel: w474 -> [w494]
          tunnel: w473 -> [w490]
          tunnel: w471 -> [w504]
          tunnel: [w504] -> w470
          tunnel: [w500] -> w469
          tunnel: [w501] -> w464
          tunnel: [w502] -> w463
          tunnel: [w503] -> w462
          tunnel: [w540] -> w481
          tunnel: [w539] -> w480
          tunnel: [w538] -> w487
          tunnel: [w537] -> w486
          tunnel: w485 -> [w536]
          tunnel: w484 -> [w535]
          tunnel: w460 -> [w531]
          tunnel: w461 -> [w530]
          tunnel: [w529] -> w483
          tunnel: [w528] -> w482
          tunnel: w470 -> [w522]
          tunnel: w479 -> [w523]
          tunnel: w469 -> [w520]
          tunnel: [w518] -> w468
          tunnel: [w517] -> w467
          tunnel: w466 -> [w512]
          tunnel: w465 -> [w511]
          tunnel: w464 -> [w521]
          tunnel: w463 -> [w508]
          tunnel: w462 -> [w515]
          frame #0 {
            # "initial"
            n132 = call "Time Delay3"("Delay Time (s)"=w499) -> ()  [unwired: 10 in, 1 out]
            n133 = local read "yoko_range"() -> (w489:string)
            n134 = call "sweepcalc_mainsweep.vi"("loop in"=w494, "step"=w496, "initial"=w497, "final"=w490) -> ("stop condition"=w493:bool, "value to write"=w495:dbl, "loop out"=w492:dbl)  [unwired: 1 in]
            n135 = call "Untitled 5 (SubVI).vi"("yoko_range"=w489, "value to write"=w495, "VISA Refnum in"=w498) -> ("Numeric"=w491:dbl)  [unwired: 8 in]
            n136 = local write "Vspt"(w491) -> ()
          }
          frame #1 {
            n137 = local read "VISA Agilent in"() -> (w502:refnum<visa-resource-name>)
            n138 = local read "Keith_DMM_VISA"() -> (w503:refnum<visa-resource-name>)
            n139 = local read "34461A_1 Adrs"() -> (w501:refnum<visa-resource-name>)
            n140 = local read "34461A_2_Adrs"() -> (w500:refnum<visa-resource-name>)
          }
          frame #2 {
            w514 = errorcluster {"status"=FALSE, "code"=0, "source"=""} ("error out")
            w525 = "\t"
            n141 = local read "chart buffer"() -> (w507:i32)
            n142 = flat-sequence {
              tunnel: w519 -> [w559]
              tunnel: w515 -> [w558]
              tunnel: w508 -> [w557]
              tunnel: w514 -> [w556]
              tunnel: w514 -> [w550]
              tunnel: [w547] -> w505
              tunnel: [w548] -> w513
              tunnel: w507 -> [w546]
              frame #0 {
                n143 = call "Read (Single Point).vi"("VISA resource name"=w558, "error in (no error)"=w550) -> ("Measurement"=w548:dbl)  [unwired: 11 in, 2 out]
                n144 = call "Read (Single Point).vi"("error in (no error)"=w556, "VISA resource name"=w557) -> ("Measurement"=w547:dbl)  [unwired: 7 in, 2 out]
                n145 = local write "Meas Bias"(w547) -> ()
                n146 = local write "Vdrop"(w548) -> ()
                n147 = local read "pre-resistance"() -> (w553:dbl)
                n148 = local read "CA gain"() -> (w552:dbl)
                n149 = call "Current calc__Agilent _for IETS loop.vi"("Vdrop"=w548, "pre-resistance"=w553, "Measurement Voltage"=w547, "CA gain"=w552) -> ("Current"=w555:dbl)  [unwired: 11 in]
                n150 = call "Resistance_SMU.vi"("CA gain"=w552, "cable and pre-resistance"=w553) -> ("Output conductance"=w551:dbl)  [unwired: 8 in, 1 out]
                n151 = local write "G_drop"(w551) -> ()
                n152 = local write "Current mA"(w555) -> ()
                n153 = Bundle("Measurement"=w547, "Current"=w555) -> (w549:cluster{"Measurement":dbl, "Current":dbl})  [unwired: 1 in]
                n154 = call "XY Chart Buffer.vi"("clear first (no:F)"=w559, "chart length (points)"=w546, "new point"=w549) -> ("XY chart data"=w554:cluster{"x":dbl, "y":dbl}[])  [unwired: 8 in]
                n155 = local write "IV_chart"(w554) -> ()
              }
            }
            n156 = flat-sequence {
              tunnel: [w573] -> w510
              tunnel: w505 -> [w572]
              tunnel: w520 -> [w571]
              tunnel: w519 -> [w570]
              tunnel: [w564] -> w518
              tunnel: [w563] -> w517
              tunnel: [w562] -> w516
              tunnel: w511 -> [w561]
              tunnel: w507 -> [w560]
              frame #0 {
                n157 = call "Read (Single Point).vi"("error in (no error)"=w561, "VISA resource name"=w571) -> ("error out"=w563:errorcluster, "Measurement"=w573:dbl, "VISA resource name out"=w564:refnum<visa-resource-name>)  [unwired: 7 in]
                n158 = local write "Lia2_DMM"(w573) -> ()
                n159 = local read "invert 2"() -> (w569:bool)
                n160 = case shown="True" w569 {
                  tunnel: w573 -> [w574 w577]
                  tunnel: [w574 w575] -> w562
                  frame False {
                  }
                  frame True {
                    n161 = Multiply(x=w577, y=-1.0) -> (x*y=w575:dbl)
                  }
                }
                n162 = local read "prefactor 2"() -> (w566:dbl)
                n163 = Multiply(x=w566, y=w562) -> (x*y=w565:dbl)
                n164 = local write "sec ampl"(w565) -> ()
                n165 = Bundle("Measurement"=w572, "Measurement"=w562) -> (w568:cluster{"Measurement":dbl, "Measurement":dbl})  [unwired: 1 in]
                n166 = call "XY Chart Buffer.vi"("clear first (no:F)"=w570, "chart length (points)"=w560, "new point"=w568) -> ("XY chart data"=w567:cluster{"x":dbl, "y":dbl}[])  [unwired: 8 in]
                n167 = local write "XY Graph  sec"(w567) -> ()
              }
            }
            n168 = flat-sequence {
              tunnel: [w578] -> w542
              tunnel: w512 -> [w593]
              tunnel: [w592] -> w540
              tunnel: [w591] -> w539
              tunnel: w519 -> [w590]
              tunnel: w505 -> [w589]
              tunnel: w521 -> [w588]
              tunnel: [w582] -> w509
              frame #0 {
                n169 = call "Read (Single Point).vi"("error in (no error)"=w593, "VISA resource name"=w588) -> ("error out"=w591:errorcluster, "Measurement"=w582:dbl, "VISA resource name out"=w592:refnum<visa-resource-name>)  [unwired: 7 in]
                n170 = local write "LIAI_1_DMM"(w582) -> ()
                n171 = local read "pre-resistance"() -> (w579:dbl)
                n172 = local read "invert"() -> (w587:bool)
                n173 = case shown="True" w587 {
                  tunnel: w582 -> [w594 w597]
                  tunnel: [w594 w595] -> w583
                  frame False {
                  }
                  frame True {
                    n174 = Multiply(x=w597, y=-1.0) -> (x*y=w595:dbl)
                  }
                }
                n175 = local read "prefactor1"() -> (w584:dbl)
                n176 = Multiply(x=w584, y=w583) -> (x*y=w580:dbl)
                n177 = call "LIA1GG0-subs_R_pre_corrected.vi"("LIA_G_all"=w580, "R_pre"=w579) -> ("G_subsR_pre"=w578:dbl)  [unwired: 6 in]
                n178 = Bundle("Measurement"=w589, "G_subsR_pre"=w578) -> (w586:cluster{"Measurement":dbl, "G_subsR_pre":dbl})  [unwired: 1 in]
                n179 = call "XY Chart Buffer.vi"("clear first (no:F)"=w590, "chart length (points)"="chart buffer", "new point"=w586) -> ("XY chart data"=w585:cluster{"x":dbl, "y":dbl}[])  [unwired: 8 in]
                n180 = local write "LIA_DMM_G"(w578) -> ()
                n181 = local write "LIA1_chart"(w585) -> ()
              }
            }
            n182 = call "Lock_in_lastsweep.vi"(10:"VISA Refnum in"=w531, 11:"VISA Refnum in"=w530) -> ("Measurement"=w506:dbl, "Measurement 4"=w534:dbl, "VISA Refnum out"=w529:refnum<visa-resource-name>, "Measurement 3"=w533:dbl, "VISA resource name out"=w528:refnum<visa-resource-name>, "Measurement 2"=w532:dbl)  [unwired: 4 in]
            "LIA2_theta" <- w506
            n183 = Format Into String(initial string=w536, error in=w535, w522, w525, w534, w525, w506, w525, w533, w525, w532, w525, w513, w525, w509, w525, w510, w525, w505, "\r\n") -> (resulting string=w538:refnum<file>, error out=w537:errorcluster)  [unwired: 1 in]
            n184 = Divide(x=w542, y=w516) -> (x/y=w541:dbl)
            n185 = Bundle("Measurement"=w505, w541) -> (w545:cluster{"Measurement":dbl, dbl})  [unwired: 1 in]
            n186 = call "XY Chart Buffer.vi"("clear first (no:F)"=FALSE, "chart length (points)"=850, "new point"=w545) -> ("XY chart data"=w527:cluster{"x":dbl, "y":dbl}[])  [unwired: 8 in]
            n187 = local read "Reset graph"() -> (w524:bool)
            n188 = call "Untitled 6 (SubVI).vi"("Numeric"=w523, "Reset graph"=w524) -> ("Boolean"=w519:bool)  [unwired: 9 in]
            n189 = local write "XY Graph X/Y"(w527) -> ()
            "Vspt" <- w522
          }
        }
        "stop last sweep" <- w472
      }
      n190 = Close File(refnum=w459, error in=w458) -> ()  [unwired: 2 out]
      "bias after mainsweep" <- w451
    }
  }
  n191 = call <vilib>:"Open_Create_Replace File.vi"("function (open:0)"=T2."create or replace", "file path"="file path 2") -> ("error out"=w29:errorcluster, "refnum"=w28:refnum<file>)  [unwired: 6 in, 2 out]
  n192 = local read "CA gain"() -> (w34:dbl)
  n193 = local read "LIA exp 1"() -> (w37:dbl)
  n194 = local read "Sensitivity 2"() -> (w35:dbl)
  n195 = local read "Sens_LIA 1"() -> (w36:dbl)
  n196 = local read "pre-resistance"() -> (w1:dbl)
  n197 = local read "LIA exp 2"() -> (w19:dbl)
  n198 = call <vilib>:"Open_Create_Replace File.vi"("function (open:0)"=T2."create or replace", "file path"="file path 3") -> ("error out"=w22:errorcluster, "refnum"=w23:refnum<file>)  [unwired: 6 in, 2 out]
  n199 = call <vilib>:"Open_Create_Replace File.vi"("function (open:0)"=T2."create or replace", "file path"="file path") -> ("error out"=w42:errorcluster, "refnum"=w41:refnum<file>)  [unwired: 6 in, 2 out]
